vi "Autonomous Independent.vi"() -> ()   [LabVIEW 2017]
doc: "This VI is called when autonomous begins, and will automatically be terminated when autonomous ends. You can carry out timed or sensor driven robot movement independently without needing to return to the caller."
uses:
  <vilib>/Rock Robotics/WPI/Solenoid/WPI_SolenoidValue.ctl
  <vilib>/Rock Robotics/WPI/Utilities/WPI_GetSetVariantRefNum.vi
  <vilib>/Rock Robotics/Network Tables/NT Read String.vi
  <vilib>/Rock Robotics/Network Tables/NT Write Numeric Array.vi
  <vilib>/Rock Robotics/WPI/ThirdParty/Phoenix-LabVIEW/Motor Controller/Get/CTRE_Phoenix_MotorController_GetQuadratureData.vi
  Robot Global Data.vi
  <vilib>/addons/control/pid/pid.llb/PID (DBL).vi
  <vilib>/Rock Robotics/WPI/RobotDrive/WPI_RobotDriveArcadeDrive_Standard(NoSaturation).vi
  <vilib>/Rock Robotics/WPI/Solenoid/WPI_SolenoidSetEnum.vi
  <vilib>/Rock Robotics/WPI/Solenoid/Deprecated/WPI_SolenoidGetBool.vi
  <vilib>/Rock Robotics/WPI/ThirdParty/Phoenix-LabVIEW/Motor Controller/Get/CTRE_Phoenix_MotorController_GetGeneralStatus.vi
  <vilib>/addons/control/pid/NI_PID_pid.lvlib
panel:
  out "Place 2 Scale":bool
  out "Place 1 Scale":bool
  out "Robots Decision 2":string
  out "Place Switch and Scale":bool
  out "Drive Forward":bool
  out "Place 2 Switch":bool
  out "Center Place 1 Switch":bool
  out "Game Data":string
  out "Right":bool
  out "Center":bool
  out "Left":bool
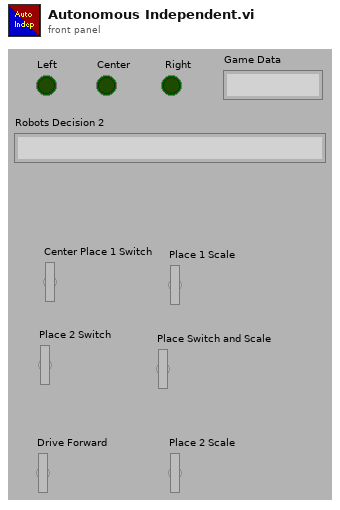
[diagram p1: front panel]
types:
  T1 = enum16{"Drive Forward", "None", "Right", "Center", "Left"}
  T2 = typedef "WPI_JoystickDevRef.ctl" = cluster{"Device":T3}
  T3 = typedef "WPI_JoystickDeviceEnum.ctl" = enum16{"USB 0", "USB 1", "USB 2", "USB 3", "USB 4", "USB 5"}
  T4 = enum16{"Place 2 Scale Left", "Place 2 Scale Right", "Place Scale Right", "Place Switch and Scale Right", "Place 2 Switch Right", "Center Place 2 Switch Right", "Center Place 1 Switch Right", "Center Place 2 Switch Left", "Center Place 1 Switch Left", "Place Scale Left", "Place Switch and Scale Left", "Place 2 Switch Left", "Drive forward", "Do Nothing"}
  T5 = enum16{"Place 2 Scale", "Place 1 Scale", "Place Switch and Scale", "Place 2 Switch", "Center Place 2 Switch", "Center Place 1 Switch", "None"}
  T6 = typedef "WPI_SolenoidValue.ctl" = enum16{"Off", "On", "Forward", "Reverse"}
  T7 = cluster{"proportional gain (Kc)":dbl, "integral time (Ti, min)":dbl, "derivative time (Td, min)":dbl}
  T8 = typedef "WPI_MotorControlDeviceRef.ctl" = cluster{"DeviceStatus":errorcluster, "Type":T9, "PWM":cluster{"PWM Channel":T10, "DeadBand":T11}, "CAN":cluster{"Device Number":u8, "SetOutput VI Ref":variant, "GetOutput VI Ref":variant, "Enable VI Ref":variant, "Disable VI Ref":variant, "Data":variant}, "Invert":bool, "DIO PWM":cluster{"PWM \"Enable\" Channel":T10, "DIOChannel":T12, "PWM Rate":dbl}}
  T9 = typedef "WPI_MotorControlType.ctl" = enum16{"PWM", "CAN", "DIO PWM"}
  T10 = typedef "FPGA_DIOPWMChannel.ctl" = enum8{"PWM 0", "PWM 1", "PWM 2", "PWM 3", "PWM 4", "PWM 5", "PWM 6", "PWM 7", "PWM 8", "PWM 9", "PWM MXP 0", "PWM MXP 1", "PWM MXP 2", "PWM MXP 3", "PWM MXP 4", "PWM MXP 5", "PWM MXP 6", "PWM MXP 7", "PWM MXP 8", "PWM MXP 9", "Invalid"}
  T11 = typedef "WPI_PWMDeadband.ctl" = cluster{"Name":string, "maxPositivePwm":i32, "minPositivePwm":i32, "centerPwm":i32, "maxNegativePwm":i32, "minNegativePwm":i32, "angularRange":u16}
  T12 = typedef "FPGA_DIOChannel.ctl" = enum8{"DIO 0", "DIO 1", "DIO 2", "DIO 3", "DIO 4", "DIO 5", "DIO 6", "DIO 7", "DIO 8", "DIO 9", "DIO MXP 0", "DIO MXP 1", "DIO MXP 2", "DIO MXP 3", "DIO MXP 4", "DIO MXP 5", "DIO MXP 6", "DIO MXP 7", "DIO MXP 8", "DIO MXP 9", "DIO MXP 10", "DIO MXP 11", "DIO MXP 12", "DIO MXP 13", "DIO MXP 14", "DIO MXP 15", "SPI Port CS1", "SPI Port CS2", "SPI Port CS3", "SPI Port MISO", "SPI Port MOSI", "Invalid"}
  T13 = typedef "CTRE_PigeonIMU_DeviceRef.ctl" = cluster{"DeviceStatus":errorcluster, "Device Number":u8, "Type":T14, "Device ID":u32, "Handle":u64, "UsageFrame":u32, "Library Path":path}
  T14 = typedef "CTRE_PigeonIMU_ConnectionType.ctl" = u32
  T15 = typedef "WPI_RobotDriveDevRef.ctl" = cluster{"DevStatus":errorcluster, "Motors[]":T8[], "Square Inputs":bool, "Max Output":dbl}
  T16 = typedef "WPI_SolenoidDevRef.ctl" = cluster{"DevStatus":errorcluster, "Pneumatics Control Module":u8, "Forward Solenoid Channel":T17, "Reverse Solenoid Channel":T17}
  T17 = typedef "WPI_SolenoidChannel.ctl" = enum8{"Solenoid 0", "Solenoid 1", "Solenoid 2", "Solenoid 3", "Solenoid 4", "Solenoid 5", "Solenoid 6", "Solenoid 7", "Invalid"}
  T18 = typedef "WPI_DigitalInputDevRef.ctl" = cluster{"DevStatus":errorcluster, "DIO Channel":T12}
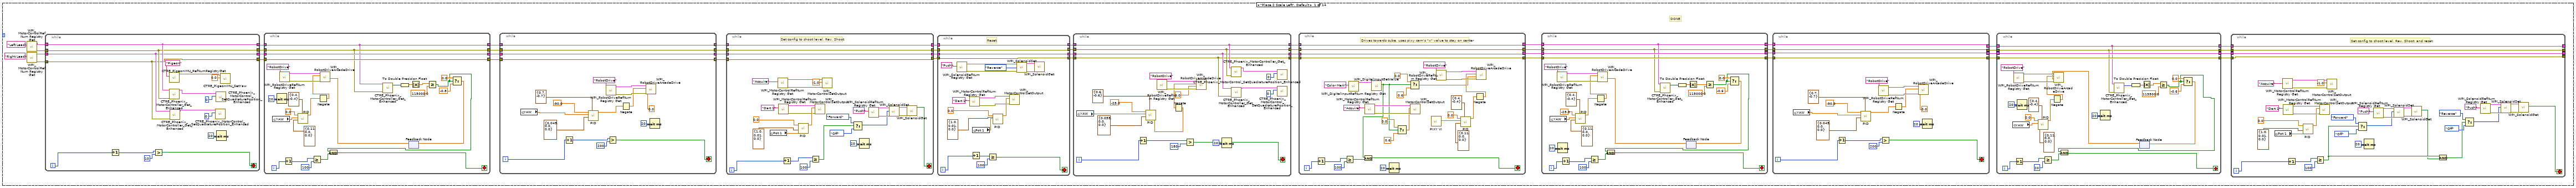
[diagram p2: hidden frame]
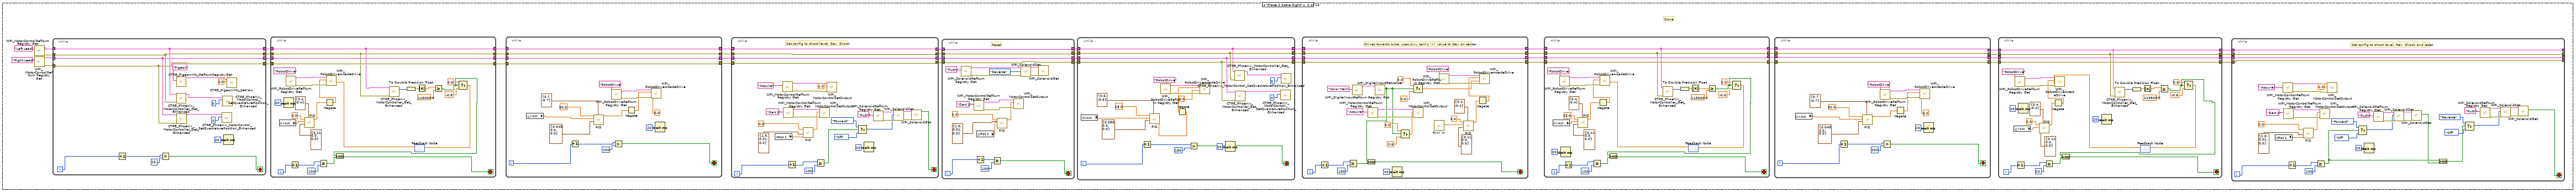
[diagram p3: hidden frame]
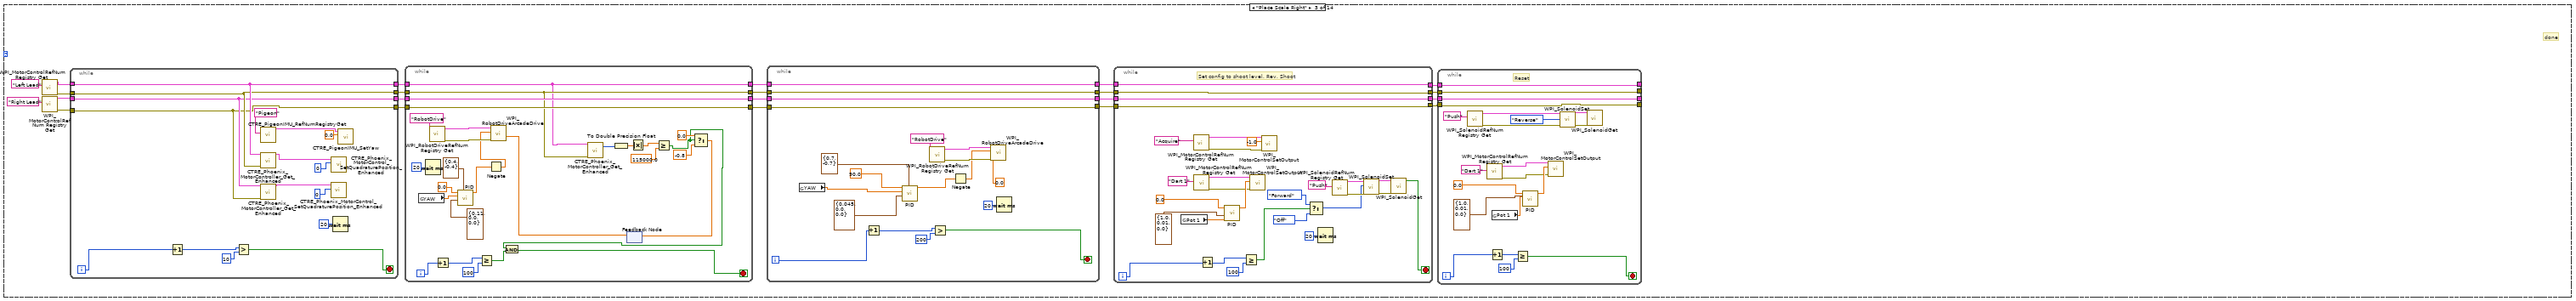
[diagram p4: hidden frame]
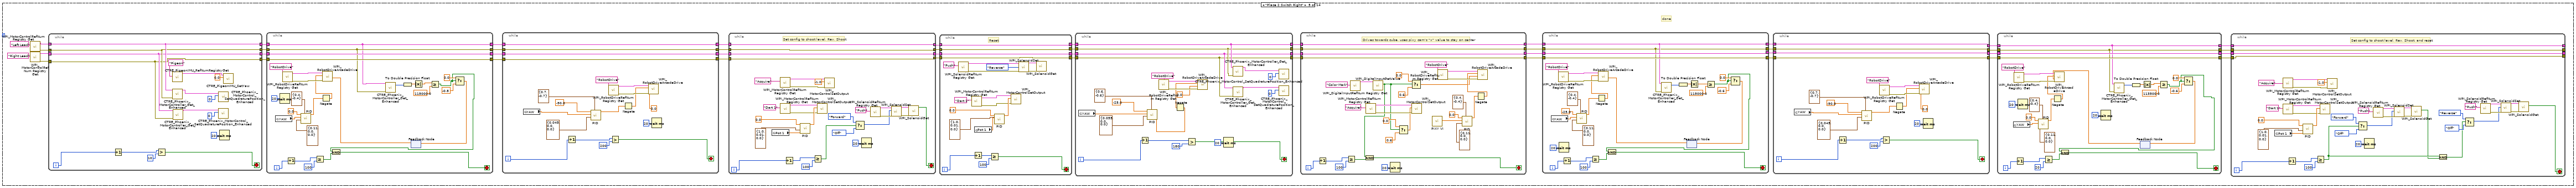
[diagram p5: hidden frame]
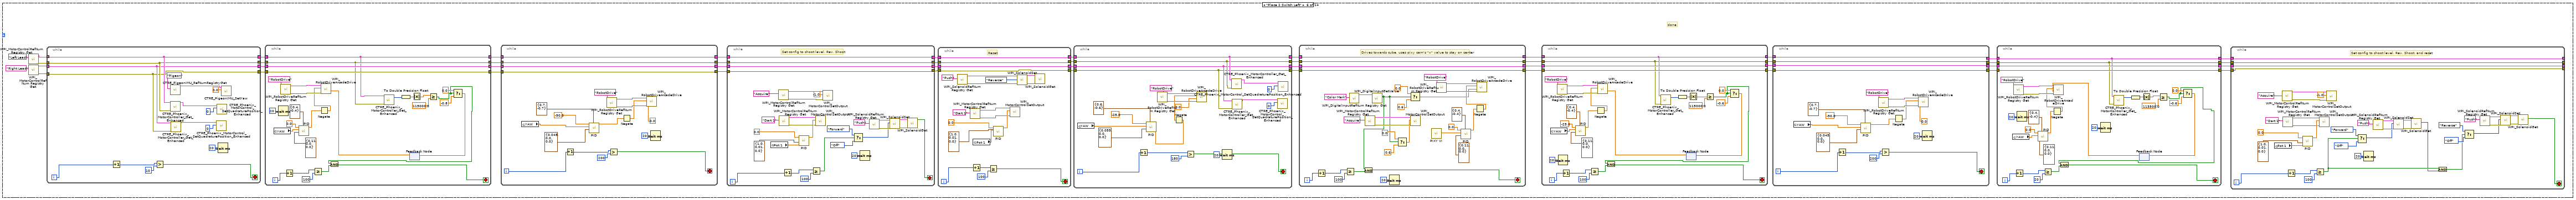
[diagram p6: hidden frame]
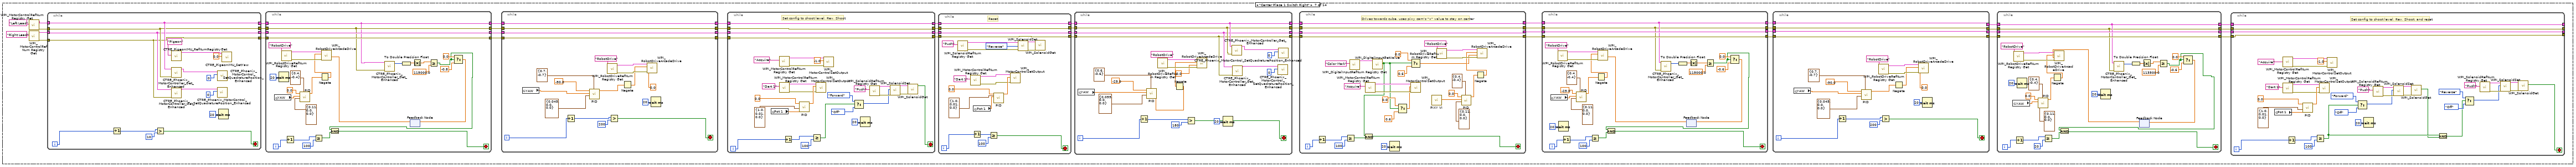
[diagram p7: hidden frame]
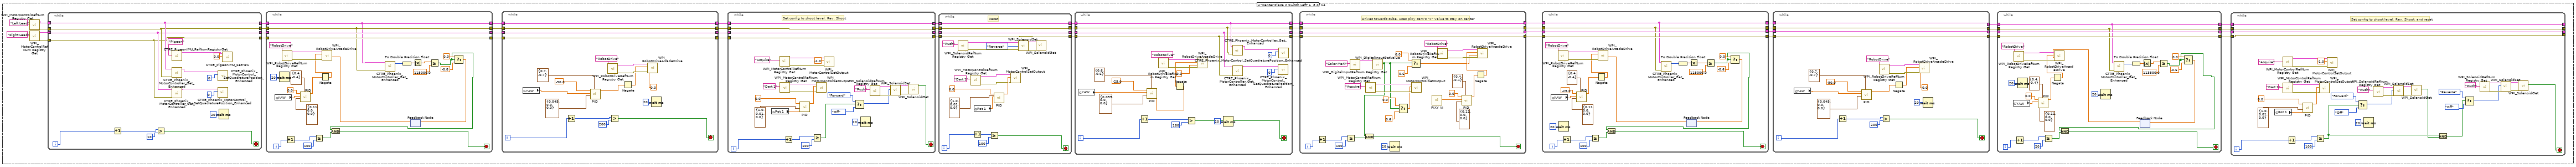
[diagram p8: hidden frame]
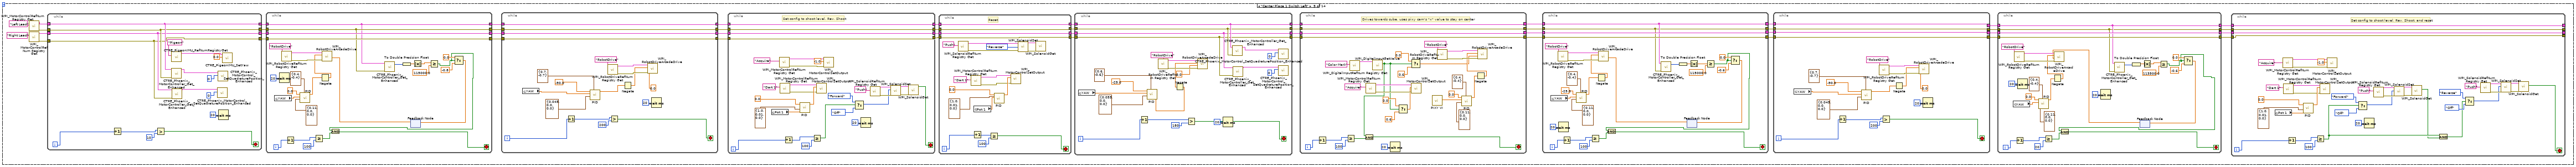
[diagram p9: hidden frame]
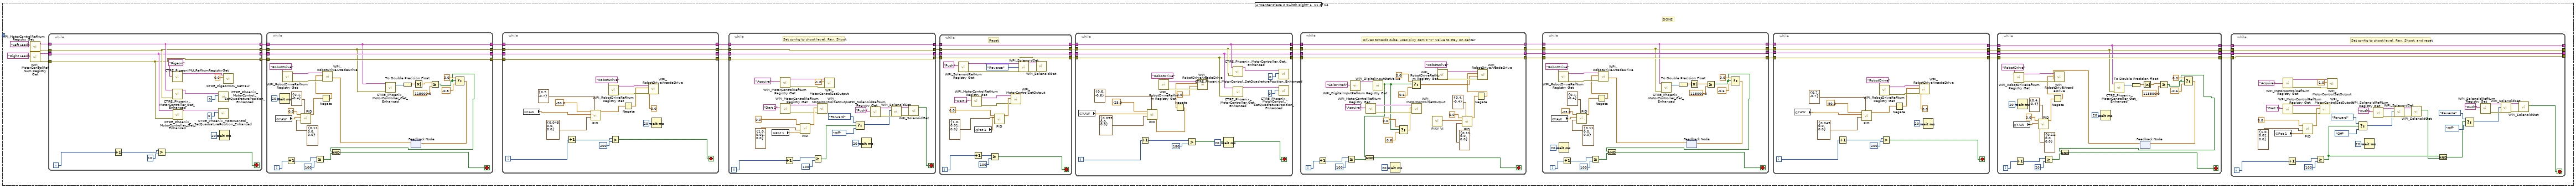
[diagram p11: hidden frame]
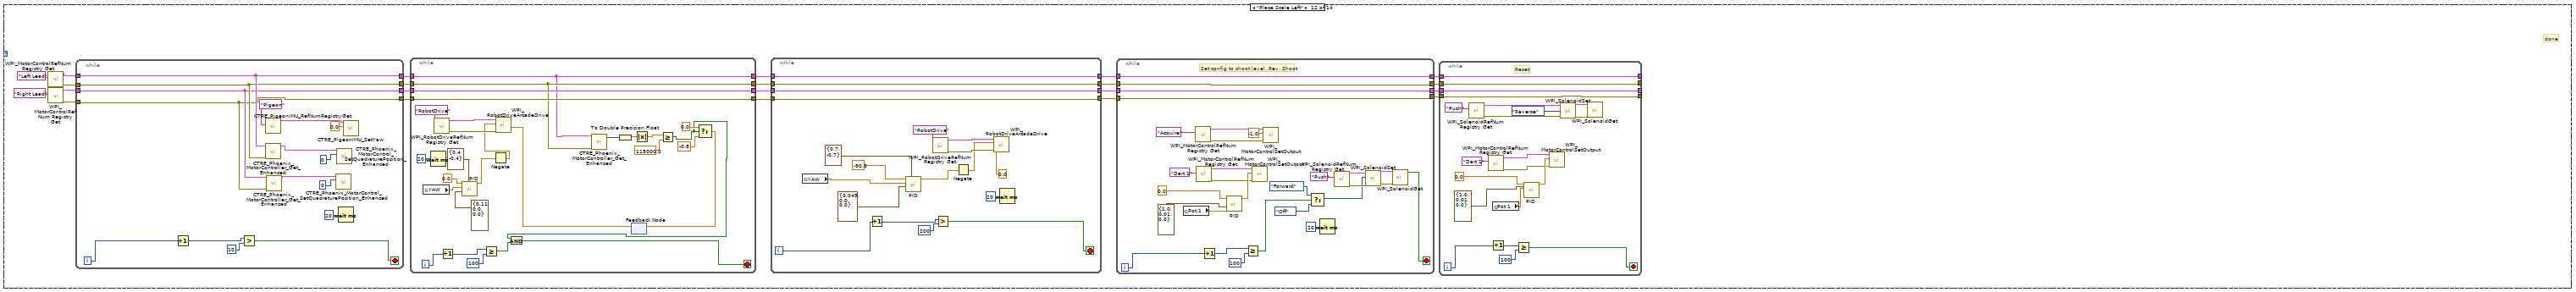
[diagram p12: hidden frame]
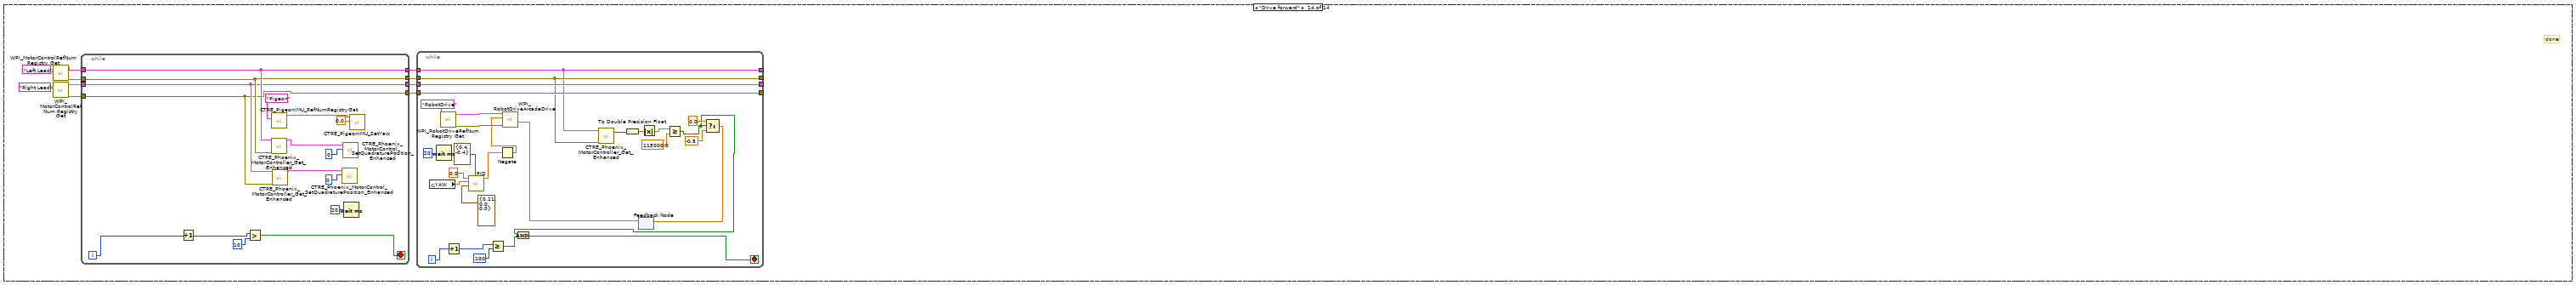
[diagram p14: hidden frame]
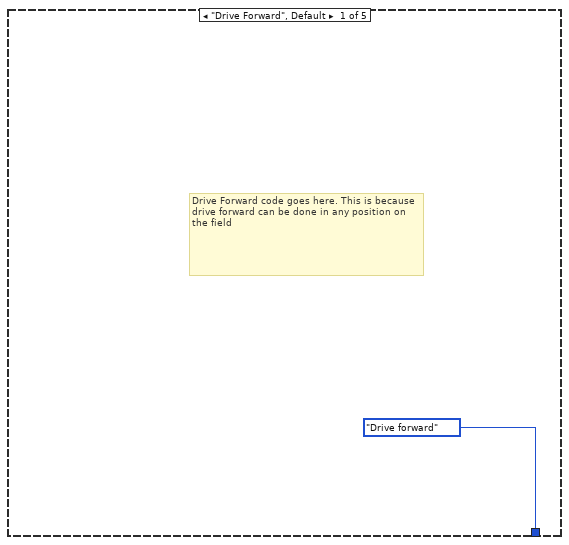
[diagram p15: hidden frame]
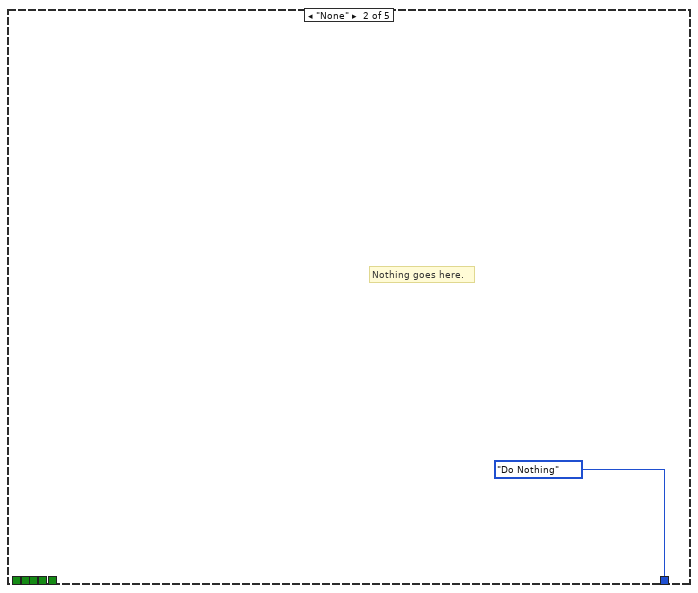
[diagram p16: hidden frame]
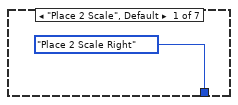
[diagram p17: hidden frame]
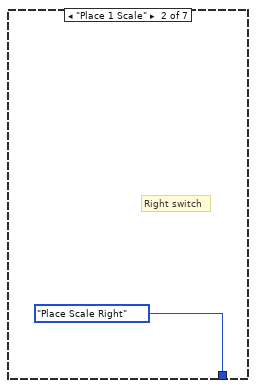
[diagram p18: hidden frame]
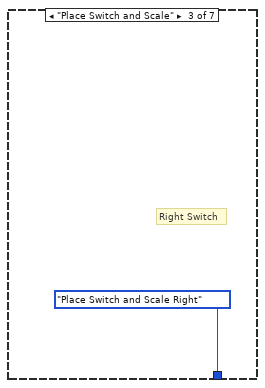
[diagram p19: hidden frame]
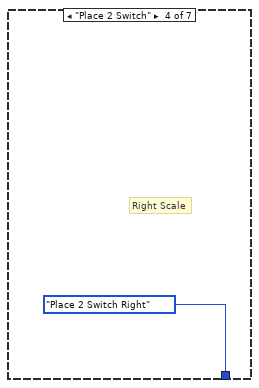
[diagram p20: hidden frame]
diagram:
  (unwired) "This function is run in parallel when the autonomous period begins. It will be terminated automatically when the period ends.\n\nNote that all Driver Station inputs are automatically latched and will not change once auto begins."
  # "5"
  # "LOGIC ALGORITHM"
  # "ALL AUTON STEPS GOES HERE"
  # "Players Choice"
  # "Order of difficulty"
  # "4"
  # "3"
  # "2"
  # "1"
  # "Game Data"
  # "Position"
  # "Position"
  # "LOGIC ALGORITHM"
  # "ALL AUTON STEPS GOES HERE"
  # "Position"
  # "This tells you the autonomous selected\nfrom the dashboard"
  # "Every 20ms, report that we are running autonomous\ncode. Loop will abort the same time as the VI."
  # "This gives you the joystick value\nthat is often the throttle"
  # "This tells you the driver position\nand alliance color"
  n1 = call <vilib>:"WPI_JoystickRefNum Registry Get.vi"("refnum name"="Autons") -> ("error out"=w43:errorcluster, "JoystickDevRef"=w44:T2)  [unwired: 9 in]
  n2 = call <vilib>:"WPI_JoystickGetValues.vi"("error in (no error)"=w43, "JoystickDevRef"=w44) -> ("Buttons"=w41:bool[])  [unwired: 5 in, 4 out]
  n3 = Index Array(array=w41) -> (element #1=w10:bool, element #2=w9:bool, element #3=w8:bool, element #4=w7:bool, element #5=w6:bool, element #6=w5:bool, element #7=w4:bool, element #8=w3:bool, element #9=w2:bool)  [unwired: 19 in, 10 out]
  "Left" <- w10
  "Center" <- w9
  "Right" <- w8
  "Center Place 1 Switch" <- w6
  "Place 2 Switch" <- w5
  "Drive Forward" <- w7
  "Place Switch and Scale" <- w2
  "Place 1 Scale" <- w4
  "Place 2 Scale" <- w3
  n4 = call <vilib>:"WPI_DriverStationGame Specific Data.vi"() -> ("Game Specific Data"=w1:string)  [unwired: 11 in]
  "Game Data" <- w1
  n5 = Select(t=T1."Right", s=w8, f=T1."None") -> (s? t:f=w37:T1)
  n6 = String Subset(string=w1, length (rest)=2 ("length (rest)")) -> (substring=w32:string)  [unwired: 1 in]
  n7 = Select(t=T1."Center", s=w9, f=w37) -> (s? t:f=w38:T1)
  n8 = Equal?(x=w32, y="RL") -> (x = y?=w26:bool)
  n9 = Equal?(x=w32, y="LR") -> (x = y?=w25:bool)
  n10 = Equal?(x=w32, y="LL") -> (x = y?=w28:bool)
  n11 = Equal?(x=w32, y="RR") -> (x = y?=w27:bool)
  n12 = Select(t=T1."Left", s=w10, f=w38) -> (s? t:f=w15:T1)
  n13 = Select(t=enum16{"None", "LR", "RL", "LL", "RR"}."LR", s=w25, f=enum16{"None", "LR", "RL", "LL", "RR"}."None") -> (s? t:f=w22:enum16{"None", "LR", "RL", "LL", "RR"})
  n14 = Select(t=enum16{"None", "LR", "RL", "LL", "RR"}."RL", s=w26, f=w22) -> (s? t:f=w23:enum16{"None", "LR", "RL", "LL", "RR"})
  n15 = Select(t=enum16{"None", "LR", "RL", "LL", "RR"}."RR", s=w27, f=w23) -> (s? t:f=w24:enum16{"None", "LR", "RL", "LL", "RR"})
  n16 = Select(t=enum16{"None", "LR", "RL", "LL", "RR"}."LL", s=w28, f=w24) -> (s? t:f=w16:enum16{"None", "LR", "RL", "LL", "RR"})
  n17 = Select(t=T1."Drive Forward", s=w7, f=w15) -> (s? t:f=w13:T1)
  n18 = case shown="\"Right\"" w13 {
    tunnel: w16 -> [_ _ w59 w140 w244]
    tunnel: w6 -> [_ _ w56 w136 w243]
    tunnel: w5 -> [_ _ w57 w137 w242]
    tunnel: w4 -> [_ _ w55 w138 w241]
    tunnel: w2 -> [_ _ w58 w139 w240]
    tunnel: w3 -> [_ _ w54 w134 w238]
    tunnel: [T4."Drive forward" T4."Do Nothing" w53 w135 w239] -> w11
    frame "Drive Forward", Default {
      # "Drive Forward code goes here. This is because drive forward can be done in any position on the field"
    }
    frame "None" {
      # "Nothing goes here."
    }
    frame "Right" {
      # "Game Data"
      n19 = case shown="\"RR\"" w59 {
        tunnel: w58 -> [w68 _ w91 w111 _]
        tunnel: w55 -> [w73 _ w89 w113 _]
        tunnel: w57 -> [w72 _ w88 w114 _]
        tunnel: w56 -> [w71 _ w87 w115 _]
        tunnel: w54 -> [w67 _ w90 w112 _]
        tunnel: [w61 T4."Drive forward" w86 w109 T4."Do Nothing"] -> w53
        frame "RR" {
          # "Can do any auton"
          # "Right RR"
          n20 = Select(t=T5."Place Switch and Scale", s=w68, f=T5."None") -> (s? t:f=w69:T5)
          n21 = Select(t=T5."Place 2 Scale", s=w67, f=w69) -> (s? t:f=w76:T5)
          n22 = Select(t=T5."Place 1 Scale", s=w73, f=w76) -> (s? t:f=w75:T5)
          n23 = Select(t=T5."Place 2 Switch", s=w72, f=w75) -> (s? t:f=w74:T5)
          n24 = Select(t=T5."Place 1 Scale", s=w71, f=w74) -> (s? t:f=w70:T5)
          n25 = case shown="\"None\"" w70 {
            tunnel: [T4."Place 2 Scale Right" T4."Place Scale Right" T4."Place Switch and Scale Right" T4."Place 2 Switch Right" T4."Do Nothing" T4."Do Nothing" T4."Do Nothing"] -> w61
            frame "Place 2 Scale", Default {
            }
            frame "Place 1 Scale" {
              # "Right switch"
            }
            frame "Place Switch and Scale" {
              # "Right Switch"
            }
            frame "Place 2 Switch" {
              # "Right Scale"
            }
            frame "Center Place 2 Switch" {
              # "Right Side"
            }
            frame "Center Place 1 Switch" {
            }
            frame "None" {
            }
          }
        }
        frame "LL" {
          # "All code gets written into a seperate case strucutre that is linked with the robot deicision made here.\nThis allows us to use the auton code \"universal\" and acts as an extension for ease of writing as well."
          # "You can not score a cube so drive forward code goes here"
          # "Right LL"
        }
        frame "RL" {
          # "Can do any auton"
          # "Right RL"
          n26 = Select(t=T5."Place 2 Switch", s=w91, f=T5."None") -> (s? t:f=w97:T5)
          n27 = Select(t=T5."Place 2 Switch", s=w90, f=w97) -> (s? t:f=w101:T5)
          n28 = Select(t=T5."Place 2 Switch", s=w89, f=w101) -> (s? t:f=w100:T5)
          n29 = Select(t=T5."Place 2 Switch", s=w88, f=w100) -> (s? t:f=w99:T5)
          n30 = Select(t=T5."Place 2 Switch", s=w87, f=w99) -> (s? t:f=w98:T5)
          n31 = case shown="\"Center Place 2 Switch\"" w98 {
            tunnel: [T4."Place 2 Scale Right" T4."Place Scale Right" T4."Place Switch and Scale Right" T4."Place 2 Switch Right" T4."Do Nothing" T4."Do Nothing" T4."Do Nothing"] -> w86
            frame "Place 2 Scale", Default {
            }
            frame "Place 1 Scale" {
              # "Right switch"
            }
            frame "Place Switch and Scale" {
              # "Right Switch"
            }
            frame "Place 2 Switch" {
              # "Right Scale"
            }
            frame "Center Place 2 Switch" {
              # "Right Side"
            }
            frame "Center Place 1 Switch" {
            }
            frame "None" {
            }
          }
        }
        frame "LR" {
          # "Can do any auton"
          # "Right LR"
          n32 = Select(t=T5."Place 2 Scale", s=w111, f=T5."None") -> (s? t:f=w121:T5)
          n33 = Select(t=T5."Place 2 Scale", s=w112, f=w121) -> (s? t:f=w125:T5)
          n34 = Select(t=T5."Place 1 Scale", s=w113, f=w125) -> (s? t:f=w124:T5)
          n35 = Select(t=T5."Place 2 Scale", s=w114, f=w124) -> (s? t:f=w123:T5)
          n36 = Select(t=T5."Place 2 Scale", s=w115, f=w123) -> (s? t:f=w122:T5)
          n37 = case shown="\"Place 1 Scale\"" w122 {
            tunnel: [T4."Place 2 Scale Right" T4."Place Scale Right" T4."Place Switch and Scale Right" T4."Place 2 Switch Right" T4."Do Nothing" T4."Do Nothing" T4."Do Nothing"] -> w109
            frame "Place 2 Scale", Default {
            }
            frame "Place 1 Scale" {
              # "Right switch"
            }
            frame "Place Switch and Scale" {
              # "Right Switch"
            }
            frame "Place 2 Switch" {
              # "Right Scale"
            }
            frame "Center Place 2 Switch" {
              # "Right Side"
            }
            frame "Center Place 1 Switch" {
            }
            frame "None" {
            }
          }
        }
        frame "None" {
          # "Nothing goes here."
        }
      }
    }
    frame "Center" {
      # "Game Data"
      n38 = case shown="\"LR\"" w140 {
        tunnel: w139 -> [w146 w170 w191 w216 _]
        tunnel: w138 -> [w144 w168 w192 w217 _]
        tunnel: w137 -> [w143 w167 w193 w218 _]
        tunnel: w136 -> [w142 w166 w194 w219 _]
        tunnel: [w141 w165 w189 w214 T4."Do Nothing"] -> w135
        tunnel: w134 -> [w145 w169 w190 w213 _]
        frame "RR" {
          # "Can do any auton"
          # "Center RR"
          n39 = Select(t=T5."Place 2 Switch", s=w146, f=T5."None") -> (s? t:f=w153:T5)
          n40 = Select(t=T5."Place 2 Switch", s=w145, f=w153) -> (s? t:f=w157:T5)
          n41 = Select(t=T5."Place 2 Switch", s=w144, f=w157) -> (s? t:f=w156:T5)
          n42 = Select(t=T5."Place 2 Switch", s=w143, f=w156) -> (s? t:f=w155:T5)
          n43 = Select(t=T5."Center Place 1 Switch", s=w142, f=w155) -> (s? t:f=w154:T5)
          n44 = case shown="\"Place 2 Scale\", Default" w154 {
            tunnel: [T4."Place 2 Scale Right" T4."Place Scale Right" T4."Place Switch and Scale Right" T4."Center Place 2 Switch Right" T4."Center Place 2 Switch Right" T4."Center Place 1 Switch Right" T4."Do Nothing"] -> w141
            frame "Place 2 Scale", Default {
            }
            frame "Place 1 Scale" {
              # "Right switch"
            }
            frame "Place Switch and Scale" {
              # "Right Switch"
            }
            frame "Place 2 Switch" {
            }
            frame "Center Place 2 Switch" {
            }
            frame "Center Place 1 Switch" {
            }
            frame "None" {
            }
          }
        }
        frame "LL" {
          # "Can do any auton"
          # "Center LL"
          n45 = Select(t=T5."Place 2 Switch", s=w170, f=T5."None") -> (s? t:f=w177:T5)
          n46 = Select(t=T5."Place 2 Switch", s=w169, f=w177) -> (s? t:f=w181:T5)
          n47 = Select(t=T5."Place 2 Switch", s=w168, f=w181) -> (s? t:f=w180:T5)
          n48 = Select(t=T5."Place 2 Switch", s=w167, f=w180) -> (s? t:f=w179:T5)
          n49 = Select(t=T5."Center Place 1 Switch", s=w166, f=w179) -> (s? t:f=w178:T5)
          n50 = case shown="\"None\"" w178 {
            tunnel: [T4."Place 2 Scale Right" T4."Place Scale Right" T4."Place Switch and Scale Right" T4."Center Place 2 Switch Left" T4."Center Place 2 Switch Left" T4."Center Place 1 Switch Left" T4."Do Nothing"] -> w165
            frame "Place 2 Scale", Default {
            }
            frame "Place 1 Scale" {
              # "Right switch"
            }
            frame "Place Switch and Scale" {
              # "Right Switch"
            }
            frame "Place 2 Switch" {
            }
            frame "Center Place 2 Switch" {
            }
            frame "Center Place 1 Switch" {
            }
            frame "None" {
            }
          }
        }
        frame "RL" {
          # "Can do any auton"
          # "Center RL"
          n51 = Select(t=T5."Place 2 Switch", s=w191, f=T5."None") -> (s? t:f=w201:T5)
          n52 = Select(t=T5."Place 2 Switch", s=w190, f=w201) -> (s? t:f=w205:T5)
          n53 = Select(t=T5."Place 2 Switch", s=w192, f=w205) -> (s? t:f=w204:T5)
          n54 = Select(t=T5."Place 2 Switch", s=w193, f=w204) -> (s? t:f=w203:T5)
          n55 = Select(t=T5."Center Place 1 Switch", s=w194, f=w203) -> (s? t:f=w202:T5)
          n56 = case shown="\"Center Place 1 Switch\"" w202 {
            tunnel: [T4."Place 2 Scale Right" T4."Place Scale Right" T4."Place Switch and Scale Right" T4."Center Place 2 Switch Right" T4."Center Place 2 Switch Right" T4."Center Place 1 Switch Right" T4."Do Nothing"] -> w189
            frame "Place 2 Scale", Default {
            }
            frame "Place 1 Scale" {
              # "Right switch"
            }
            frame "Place Switch and Scale" {
              # "Right Switch"
            }
            frame "Place 2 Switch" {
            }
            frame "Center Place 2 Switch" {
            }
            frame "Center Place 1 Switch" {
            }
            frame "None" {
            }
          }
        }
        frame "LR" {
          # "Can do any auton"
          # "Center LR"
          n57 = Select(t=T5."Place 2 Switch", s=w216, f=T5."None") -> (s? t:f=w225:T5)
          n58 = Select(t=T5."Place 2 Switch", s=w213, f=w225) -> (s? t:f=w229:T5)
          n59 = Select(t=T5."Place 2 Switch", s=w217, f=w229) -> (s? t:f=w228:T5)
          n60 = Select(t=T5."Place 2 Switch", s=w218, f=w228) -> (s? t:f=w227:T5)
          n61 = Select(t=T5."Center Place 1 Switch", s=w219, f=w227) -> (s? t:f=w226:T5)
          n62 = case shown="\"Center Place 1 Switch\"" w226 {
            tunnel: [T4."Place 2 Scale Right" T4."Place Scale Right" T4."Place Switch and Scale Right" T4."Center Place 2 Switch Left" T4."Center Place 2 Switch Left" T4."Center Place 1 Switch Left" T4."Do Nothing"] -> w214
            frame "Place 2 Scale", Default {
            }
            frame "Place 1 Scale" {
              # "Right switch"
            }
            frame "Place Switch and Scale" {
              # "Right Switch"
            }
            frame "Place 2 Switch" {
            }
            frame "Center Place 2 Switch" {
            }
            frame "Center Place 1 Switch" {
            }
            frame "None" {
            }
          }
        }
        frame "None" {
          # "Nothing goes here."
        }
      }
    }
    frame "Left" {
      n63 = case shown="\"RR\"" w244 {
        tunnel: w243 -> [_ w246 w270 w294 _]
        tunnel: w242 -> [_ w247 w271 w295 _]
        tunnel: w241 -> [_ w248 w272 w296 _]
        tunnel: w240 -> [_ w250 w274 w298 _]
        tunnel: [T4."Drive forward" w251 w275 w299 T4."Do Nothing"] -> w239
        tunnel: w238 -> [_ w249 w273 w297 _]
        frame "RR" {
          # "Game Data"
          # "You can not score a cube so drive forward code goes here"
          # "Left RR"
        }
        frame "LL" {
          # "Can do any auton"
          # "Left LL"
          n64 = Select(t=T5."Place Switch and Scale", s=w250, f=T5."None") -> (s? t:f=w258:T5)
          n65 = Select(t=T5."Place 2 Scale", s=w249, f=w258) -> (s? t:f=w262:T5)
          n66 = Select(t=T5."Place 1 Scale", s=w248, f=w262) -> (s? t:f=w261:T5)
          n67 = Select(t=T5."Place 2 Switch", s=w247, f=w261) -> (s? t:f=w260:T5)
          n68 = Select(t=T5."Place Switch and Scale", s=w246, f=w260) -> (s? t:f=w259:T5)
          n69 = case shown="\"None\"" w259 {
            tunnel: [T4."Place 2 Scale Left" T4."Place Scale Left" T4."Place Switch and Scale Left" T4."Place 2 Switch Left" T4."Center Place 2 Switch Right" T4."Center Place 1 Switch Right" T4."Do Nothing"] -> w251
            frame "Place 2 Scale", Default {
            }
            frame "Place 1 Scale" {
              # "Right switch"
            }
            frame "Place Switch and Scale" {
            }
            frame "Place 2 Switch" {
            }
            frame "Center Place 2 Switch" {
            }
            frame "Center Place 1 Switch" {
            }
            frame "None" {
            }
          }
        }
        frame "RL" {
          # "Can do any auton"
          # "Left RL"
          n70 = Select(t=T5."Place 2 Scale", s=w274, f=T5."None") -> (s? t:f=w282:T5)
          n71 = Select(t=T5."Place 2 Scale", s=w273, f=w282) -> (s? t:f=w286:T5)
          n72 = Select(t=T5."Place 1 Scale", s=w272, f=w286) -> (s? t:f=w285:T5)
          n73 = Select(t=T5."Place 2 Scale", s=w271, f=w285) -> (s? t:f=w284:T5)
          n74 = Select(t=T5."Place 2 Scale", s=w270, f=w284) -> (s? t:f=w283:T5)
          n75 = case shown="\"None\"" w283 {
            tunnel: [T4."Place 2 Scale Left" T4."Place Scale Left" T4."Place Switch and Scale Right" T4."Place 2 Switch Left" T4."Center Place 2 Switch Right" T4."Center Place 1 Switch Right" T4."Do Nothing"] -> w275
            frame "Place 2 Scale", Default {
            }
            frame "Place 1 Scale" {
              # "Right switch"
            }
            frame "Place Switch and Scale" {
              # "Right Switch"
            }
            frame "Place 2 Switch" {
            }
            frame "Center Place 2 Switch" {
            }
            frame "Center Place 1 Switch" {
            }
            frame "None" {
            }
          }
        }
        frame "LR" {
          # "Can do any auton"
          # "Left LR"
          n76 = Select(t=T5."Place 2 Switch", s=w298, f=T5."None") -> (s? t:f=w306:T5)
          n77 = Select(t=T5."Place 2 Switch", s=w297, f=w306) -> (s? t:f=w310:T5)
          n78 = Select(t=T5."Place 2 Switch", s=w296, f=w310) -> (s? t:f=w309:T5)
          n79 = Select(t=T5."Place 2 Switch", s=w295, f=w309) -> (s? t:f=w308:T5)
          n80 = Select(t=T5."Place 2 Switch", s=w294, f=w308) -> (s? t:f=w307:T5)
          n81 = case shown="\"Place 2 Switch\"" w307 {
            tunnel: [T4."Place 2 Scale Right" T4."Place Scale Right" T4."Place Switch and Scale Right" T4."Place 2 Switch Left" T4."Center Place 2 Switch Right" T4."Center Place 1 Switch Right" T4."Do Nothing"] -> w299
            frame "Place 2 Scale", Default {
            }
            frame "Place 1 Scale" {
              # "Right switch"
            }
            frame "Place Switch and Scale" {
              # "Right Switch"
            }
            frame "Place 2 Switch" {
            }
            frame "Center Place 2 Switch" {
            }
            frame "Center Place 1 Switch" {
            }
            frame "None" {
            }
          }
        }
        frame "None" {
          # "Nothing goes here."
        }
      }
    }
  }
  n82 = case shown="\"Place Switch and Scale Right\"" w11 {
    frame "Place 2 Scale Left", Default {
      # "DONE"
      n83 = call <vilib>:"WPI_MotorControlRefNum Registry Get.vi"("refnum name"="Left Lead") -> ("error out"=w323:errorcluster, "MotorControlDevRef"=w324:T8)  [unwired: 9 in]
      n84 = call <vilib>:"WPI_MotorControlRefNum Registry Get.vi"("refnum name"="Right Lead") -> ("error out"=w321:errorcluster, "MotorControlDevRef"=w322:T8)  [unwired: 9 in]
      n85 = while {
        tunnel: w324 -> [w606]
        tunnel: w323 -> [w605]
        tunnel: w322 -> [w604]
        tunnel: w321 -> [w603]
        tunnel: [w606] -> w364
        tunnel: [w605] -> w363
        tunnel: [w604] -> w362
        tunnel: [w603] -> w361
        i -> [w616]
        stop <- w615 stop-if-true
        n86 = Increment(x=w616) -> (x+1=w618:i32)
        n87 = Greater?(x=w618, y=10) -> (0:w615:bool)
        n88 = call <vilib>:"CTRE_PigeonIMU_RefNumRegistryGet.vi"("refnum name"="Pigeon") -> ("PigeonIMUDevRef"=w613:T13)  [unwired: 9 in, 1 out]
        n89 = call-poly <vilib>:"CTRE_Phoenix_MotorController_Get_Enhanced.vi"("PhoenixMotorControlDevRef"=w606, "error in"=w605) -> ("PhoenixMotorControlDevRef"=w608:T8)  [unwired: 10 in, 3 out]
        n90 = call-poly <vilib>:"CTRE_Phoenix_MotorController_Get_Enhanced.vi"("PhoenixMotorControlDevRef"=w604, "error in"=w603) -> ("PhoenixMotorControlDevRef"=w607:T8)  [unwired: 10 in, 3 out]
        n91 = call "CTRE_Phoenix_MotorControl_SetQuadraturePosition_Enhanced.vi"("New Position"=0, "PhoenixMotorControlDevRef"=w607) -> ()  [unwired: 8 in, 2 out]
        n92 = call "CTRE_Phoenix_MotorControl_SetQuadraturePosition_Enhanced.vi"("New Position"=0, "PhoenixMotorControlDevRef"=w608) -> ()  [unwired: 8 in, 2 out]
        n93 = Wait (ms)(milliseconds to wait=u32 20) -> ()  [unwired: 1 out]
        n94 = call <vilib>:"CTRE_PigeonIMU_SetYaw.vi"("Value"=0.0, "PigeonIMUDevRef"=w613) -> ()  [unwired: 8 in, 2 out]
      }
      n95 = while {
        tunnel: [w621] -> w360
        tunnel: w364 -> [w621]
        tunnel: [w622] -> w359
        tunnel: w363 -> [w622]
        tunnel: [w629] -> w358
        tunnel: w362 -> [w629]
        tunnel: [w628] -> w357
        tunnel: w361 -> [w628]
        i -> [w645]
        stop <- w641 stop-if-true
        n96 = global read "Robot Global Data.vi" "YAW"() -> (w630:dbl)
        n97 = Wait (ms)(milliseconds to wait=u32 20) -> ()  [unwired: 1 out]
        n98 = call <vilib>:"WPI_RobotDriveRefNum Registry Get.vi"("refnum name"="RobotDrive") -> ("error out"=w626:errorcluster, "RobotDriveDevRef"=w627:T15)  [unwired: 9 in]
        n99 = Increment(x=w645) -> (x+1=w644:i32)
        n100 = call-poly <vilib>:"PID.vi"("output range"=cluster{"output high":dbl, "output low":dbl} {"output high"=0.4, "output low"=-0.4}, "PID gains"=T7 {"proportional gain (Kc)"=0.11, "integral time (Ti, min)"=0.0, "derivative time (Td, min)"=0.0}, "process variable"=w630, "setpoint"=0.0) -> ("output"=w620:dbl)  [unwired: 6 in, 1 out]
        n101 = Greater Or Equal?(x=w644, y=100) -> (x >= y?=w642:bool)
        n102 = Negate(x=w620) -> (-x=w619:dbl)
        n103 = call-poly <vilib>:"CTRE_Phoenix_MotorController_Get_Enhanced.vi"("PhoenixMotorControlDevRef"=w621, "error in"=w622) -> ("Quadrature Position"=w640:i32)  [unwired: 10 in, 3 out]
        n104 = To Double Precision Float(number=w640) -> (double precision float=w639:dbl)
        n105 = feedback #1() -> (w623:dbl)  [unwired: 1 in]
        n106 = call-poly <vilib>:"WPI_RobotDriveArcadeDrive.vi"("error in (no error)"=w626, "Y axis value"=w623, "X axis value"=w619, "RobotDriveDevRef"=w627) -> ()  [unwired: 5 in, 3 out]
        n107 = Absolute Value(x=w639) -> (abs(x)=w635:dbl)
        n108 = Greater Or Equal?(x=w635, y=115000.0 ("upper limit")) -> (x >= y?=w624:bool)
        n109 = And(x=w624, y=w642) -> (x .and. y?=w641:bool)
        n110 = Select(t=0.0, s=w624, f=-0.8) -> (s? t:f=w636:dbl)
        n111 = feedback-in #1(w636) -> ()
      }
      n112 = while {
        tunnel: w360 -> [w593]
        tunnel: w359 -> [w592]
        tunnel: w358 -> [w591]
        tunnel: w357 -> [w590]
        tunnel: [w593] -> w356
        tunnel: [w592] -> w355
        tunnel: [w591] -> w354
        tunnel: [w590] -> w353
        i -> [w596]
        stop <- w594 stop-if-true
        n113 = global read "Robot Global Data.vi" "YAW"() -> (w600:dbl)
        n114 = Increment(x=w596) -> (x+1=w598:i32)
        n115 = call-poly <vilib>:"PID.vi"("output range"=cluster{"output high":dbl, "output low":dbl} {"output high"=0.7, "output low"=-0.7}, "PID gains"=T7 {"proportional gain (Kc)"=0.045, "integral time (Ti, min)"=0.0, "derivative time (Td, min)"=0.0}, "process variable"=w600, "setpoint"=-90.0) -> ("output"=w585:dbl)  [unwired: 6 in, 1 out]
        n116 = call <vilib>:"WPI_RobotDriveRefNum Registry Get.vi"("refnum name"="RobotDrive") -> ("error out"=w588:errorcluster, "RobotDriveDevRef"=w589:T15)  [unwired: 9 in]
        n117 = Greater?(x=w598, y=200) -> (0:w594:bool)
        n118 = Negate(x=w585) -> (-x=w584:dbl)
        n119 = call-poly <vilib>:"WPI_RobotDriveArcadeDrive.vi"("error in (no error)"=w588, "Y axis value"=0.0, "X axis value"=w584, "RobotDriveDevRef"=w589) -> ()  [unwired: 5 in, 3 out]
        n120 = Wait (ms)(milliseconds to wait=u32 20) -> ()  [unwired: 1 out]
      }
      n121 = while {
        tunnel: [w493] -> w352
        tunnel: w356 -> [w493]
        tunnel: [w492] -> w351
        tunnel: w355 -> [w492]
        tunnel: [w491] -> w350
        tunnel: w354 -> [w491]
        tunnel: [w494] -> w349
        tunnel: w353 -> [w494]
        i -> [w487]
        stop <- w473 stop-if-true
        # "Set config to shoot level, Rev, Shoot"
        n122 = global read "Robot Global Data.vi" "Pot 1"() -> (w495:dbl)
        n123 = call <vilib>:"WPI_MotorControlRefNum Registry Get.vi"("refnum name"="Acquire") -> ("error out"=w488:errorcluster, "MotorControlDevRef"=w489:T8)  [unwired: 9 in]
        n124 = call <vilib>:"WPI_MotorControlRefNum Registry Get.vi"("refnum name"="Dart 1") -> ("error out"=w499:errorcluster, "MotorControlDevRef"=w498:T8)  [unwired: 9 in]
        n125 = Increment(x=w487) -> (x+1=w474:i32)
        n126 = call-poly <vilib>:"PID.vi"("PID gains"=T7 {"proportional gain (Kc)"=1.0, "integral time (Ti, min)"=0.01, "derivative time (Td, min)"=0.0}, "process variable"=w495, "setpoint"=0.0) -> ("output"=w500:dbl)  [unwired: 7 in, 1 out]
        n127 = Greater Or Equal?(x=w474, y=100) -> (x >= y?=w479:bool)
        n128 = call <vilib>:"WPI_MotorControlSetOutput.vi"("error in (no error)"=w499, "Output"=w500, "MotorControlDevRef"=w498) -> ()  [unwired: 6 in, 3 out]
        n129 = call <vilib>:"WPI_MotorControlSetOutput.vi"("error in (no error)"=w488, "Output"=-1.0, "MotorControlDevRef"=w489) -> ()  [unwired: 6 in, 3 out]
        n130 = Select(t=WPI_SolenoidValue."Forward" ("Value"), s=w479, f=WPI_SolenoidValue."Off" ("Value")) -> (s? t:f=w482:T6)
        n131 = Wait (ms)(milliseconds to wait=u32 20) -> ()  [unwired: 1 out]
        n132 = call <vilib>:"WPI_SolenoidRefNum Registry Get.vi"("refnum name"="Push") -> ("error out"=w483:errorcluster, "SolenoidDevRef"=w484:T16)  [unwired: 9 in]
        n133 = call-poly <vilib>:"WPI_SolenoidSet.vi"("error in (no error)"=w483, "Value"=w482, "SolenoidDevRef"=w484) -> ("error out"=w475:errorcluster, "SolenoidDevRef"=w476:T16)  [unwired: 7 in]
        n134 = call-poly <vilib>:"WPI_SolenoidGet.vi"("error in (no error)"=w475, "SolenoidDevRef"=w476) -> ("Value"=w473:bool)  [unwired: 7 in, 2 out]
      }
      n135 = while {
        tunnel: w352 -> [w379]
        tunnel: w351 -> [w378]
        tunnel: w350 -> [w377]
        tunnel: w349 -> [w376]
        tunnel: [w379] -> w348
        tunnel: [w378] -> w347
        tunnel: [w377] -> w346
        tunnel: [w376] -> w345
        i -> [w367]
        stop <- w366 stop-if-true
        # "Reset"
        n136 = call <vilib>:"WPI_SolenoidRefNum Registry Get.vi"("refnum name"="Push") -> ("error out"=w383:errorcluster, "SolenoidDevRef"=w384:T16)  [unwired: 9 in]
        n137 = call <vilib>:"WPI_MotorControlRefNum Registry Get.vi"("refnum name"="Dart 1") -> ("error out"=w374:errorcluster, "MotorControlDevRef"=w373:T8)  [unwired: 9 in]
        n138 = Increment(x=w367) -> (x+1=w380:i32)
        n139 = global read "Robot Global Data.vi" "Pot 1"() -> (w370:dbl)
        n140 = Greater Or Equal?(x=w380, y=100) -> (x >= y?=w366:bool)
        n141 = call-poly <vilib>:"PID.vi"("PID gains"=T7 {"proportional gain (Kc)"=1.0, "integral time (Ti, min)"=0.01, "derivative time (Td, min)"=0.0}, "process variable"=w370, "setpoint"=0.0) -> ("output"=w375:dbl)  [unwired: 7 in, 1 out]
        n142 = call <vilib>:"WPI_MotorControlSetOutput.vi"("error in (no error)"=w374, "Output"=w375, "MotorControlDevRef"=w373) -> ()  [unwired: 6 in, 3 out]
        n143 = call-poly <vilib>:"WPI_SolenoidSet.vi"("error in (no error)"=w383, "Value"=WPI_SolenoidValue."Reverse", "SolenoidDevRef"=w384) -> ("error out"=w381:errorcluster, "SolenoidDevRef"=w382:T16)  [unwired: 7 in]
        n144 = call-poly <vilib>:"WPI_SolenoidGet.vi"("error in (no error)"=w381, "SolenoidDevRef"=w382) -> ()  [unwired: 7 in, 3 out]
      }
      n145 = while {
        tunnel: [w564] -> w344
        tunnel: w348 -> [w564]
        tunnel: [w563] -> w343
        tunnel: w347 -> [w563]
        tunnel: [w562] -> w342
        tunnel: w346 -> [w562]
        tunnel: [w561] -> w341
        tunnel: w345 -> [w561]
        i -> [w577]
        stop <- w575 stop-if-true
        n146 = global read "Robot Global Data.vi" "YAW"() -> (w581:dbl)
        n147 = Increment(x=w577) -> (x+1=w579:i32)
        n148 = call-poly <vilib>:"PID.vi"("output range"=cluster{"output high":dbl, "output low":dbl} {"output high"=0.6, "output low"=-0.6}, "PID gains"=T7 {"proportional gain (Kc)"=0.055, "integral time (Ti, min)"=0.0, "derivative time (Td, min)"=0.0}, "process variable"=w581, "setpoint"=-25.0) -> ("output"=w571:dbl)  [unwired: 6 in, 1 out]
        n149 = call <vilib>:"WPI_RobotDriveRefNum Registry Get.vi"("refnum name"="RobotDrive") -> ("error out"=w572:errorcluster, "RobotDriveDevRef"=w573:T15)  [unwired: 9 in]
        n150 = Negate(x=w571) -> (-x=w570:dbl)
        n151 = Greater?(x=w579, y=180) -> (0:w575:bool)
        n152 = call-poly <vilib>:"WPI_RobotDriveArcadeDrive.vi"("error in (no error)"=w572, "Y axis value"=0.0, "X axis value"=w570, "RobotDriveDevRef"=w573) -> ()  [unwired: 5 in, 3 out]
        n153 = Wait (ms)(milliseconds to wait=u32 20) -> ()  [unwired: 1 out]
        n154 = call-poly <vilib>:"CTRE_Phoenix_MotorController_Get_Enhanced.vi"("PhoenixMotorControlDevRef"=w564, "error in"=w563) -> ("PhoenixMotorControlDevRef"=w566:T8)  [unwired: 8 in, 5 out]
        n155 = call-poly <vilib>:"CTRE_Phoenix_MotorController_Get_Enhanced.vi"("PhoenixMotorControlDevRef"=w562, "error in"=w561) -> ("PhoenixMotorControlDevRef"=w565:T8)  [unwired: 8 in, 5 out]
        n156 = call "CTRE_Phoenix_MotorControl_SetQuadraturePosition_Enhanced.vi"("New Position"=0, "PhoenixMotorControlDevRef"=w565) -> ()  [unwired: 8 in, 2 out]
        n157 = call "CTRE_Phoenix_MotorControl_SetQuadraturePosition_Enhanced.vi"("New Position"=0, "PhoenixMotorControlDevRef"=w566) -> ()  [unwired: 8 in, 2 out]
      }
      n158 = while {
        tunnel: [w534] -> w340
        tunnel: w344 -> [w534]
        tunnel: [w533] -> w339
        tunnel: w343 -> [w533]
        tunnel: [w532] -> w338
        tunnel: w342 -> [w532]
        tunnel: [w531] -> w337
        tunnel: w341 -> [w531]
        i -> [w559]
        stop <- w555 stop-if-true
        # "Drives towards cube, uses pixy cam's \"x\" value to stay on center"
        n159 = Increment(x=w559) -> (x+1=w558:i32)
        n160 = Greater Or Equal?(x=w558, y=100) -> (x >= y?=w556:bool)
        n161 = call <vilib>:"WPI_DigitalInputRefNum Registry Get.vi"("refnum name"="Color Mark") -> ("DigitalInputDevRef"=w545:T18)  [unwired: 9 in, 1 out]
        n162 = call <vilib>:"WPI_MotorControlRefNum Registry Get.vi"("refnum name"="Acquire") -> ("error out"=w542:errorcluster, "MotorControlDevRef"=w543:T8)  [unwired: 9 in]
        n163 = call <vilib>:"WPI_DigitalInputGetValue.vi"("DigitalInputDevRef"=w545) -> ("Value"=w535:bool)  [unwired: 8 in, 2 out]
        n164 = And(x=w535, y=w556) -> (x .and. y?=w555:bool)
        n165 = Wait (ms)(milliseconds to wait=u32 20) -> ()  [unwired: 1 out]
        n166 = Select(t=0.0, s=w535, f=0.6) -> (s? t:f=w536:dbl)
        n167 = Select(t=0.0, s=w535, f=0.6) -> (s? t:f=w539:dbl)
        n168 = call <vilib>:"WPI_MotorControlSetOutput.vi"("error in (no error)"=w542, "Output"=w536, "MotorControlDevRef"=w543) -> ()  [unwired: 6 in, 3 out]
        n169 = call "PIXY VI.vi"() -> ("X"=w546:dbl)  [unwired: 14 in, 5 out]
        n170 = call <vilib>:"WPI_RobotDriveRefNum Registry Get.vi"("refnum name"="RobotDrive") -> ("error out"=w551:errorcluster, "RobotDriveDevRef"=w552:T15)  [unwired: 9 in]
        n171 = call-poly <vilib>:"PID.vi"("output range"=cluster{"output high":dbl, "output low":dbl} {"output high"=0.4, "output low"=-0.4}, "PID gains"=T7 {"proportional gain (Kc)"=0.11, "integral time (Ti, min)"=0.0, "derivative time (Td, min)"=0.0}, "process variable"=w546, "setpoint"=0.0) -> ("output"=w549:dbl)  [unwired: 6 in, 1 out]
        n172 = Negate(x=w549) -> (-x=w548:dbl)
        n173 = call-poly <vilib>:"WPI_RobotDriveArcadeDrive.vi"("error in (no error)"=w551, "Y axis value"=w539, "X axis value"=w548, "RobotDriveDevRef"=w552) -> ()  [unwired: 5 in, 3 out]
      }
      n174 = while {
        tunnel: [w445] -> w336
        tunnel: w340 -> [w445]
        tunnel: [w444] -> w335
        tunnel: w339 -> [w444]
        tunnel: [w447] -> w334
        tunnel: w338 -> [w447]
        tunnel: [w446] -> w333
        tunnel: w337 -> [w446]
        i -> [w470]
        stop <- w466 stop-if-true
        n175 = global read "Robot Global Data.vi" "YAW"() -> (w455:dbl)
        n176 = call <vilib>:"WPI_RobotDriveRefNum Registry Get.vi"("refnum name"="RobotDrive") -> ("error out"=w453:errorcluster, "RobotDriveDevRef"=w454:T15)  [unwired: 9 in]
        n177 = Wait (ms)(milliseconds to wait=u32 20) -> ()  [unwired: 1 out]
        n178 = Increment(x=w470) -> (x+1=w469:i32)
        n179 = call-poly <vilib>:"PID.vi"("output range"=cluster{"output high":dbl, "output low":dbl} {"output high"=0.4, "output low"=-0.4}, "PID gains"=T7 {"proportional gain (Kc)"=0.11, "integral time (Ti, min)"=0.0, "derivative time (Td, min)"=0.0}, "process variable"=w455, "setpoint"=-25.0) -> ("output"=w449:dbl)  [unwired: 6 in, 1 out]
        n180 = Greater Or Equal?(x=w469, y=100) -> (x >= y?=w467:bool)
        n181 = Negate(x=w449) -> (-x=w448:dbl)
        n182 = call-poly <vilib>:"CTRE_Phoenix_MotorController_Get_Enhanced.vi"("PhoenixMotorControlDevRef"=w445, "error in"=w444) -> ("Quadrature Position"=w465:i32)  [unwired: 10 in, 3 out]
        n183 = To Double Precision Float(number=w465) -> (double precision float=w464:dbl)
        n184 = feedback #2() -> (w450:dbl)  [unwired: 1 in]
        n185 = call-poly <vilib>:"WPI_RobotDriveArcadeDrive.vi"("error in (no error)"=w453, "Y axis value"=w450, "X axis value"=w448, "RobotDriveDevRef"=w454) -> ()  [unwired: 5 in, 3 out]
        n186 = Absolute Value(x=w464) -> (abs(x)=w460:dbl)
        n187 = Greater Or Equal?(x=w460, y=115000.0 ("upper limit")) -> (x >= y?=w451:bool)
        n188 = And(x=w451, y=w467) -> (x .and. y?=w466:bool)
        n189 = Select(t=0.0, s=w451, f=-0.6) -> (s? t:f=w461:dbl)
        n190 = feedback-in #2(w461) -> ()
      }
      n191 = while {
        tunnel: w336 -> [w428]
        tunnel: w335 -> [w427]
        tunnel: w334 -> [w426]
        tunnel: w333 -> [w425]
        tunnel: [w428] -> w332
        tunnel: [w427] -> w331
        tunnel: [w426] -> w330
        tunnel: [w425] -> w329
        i -> [w437]
        stop <- w435 stop-if-true
        n192 = global read "Robot Global Data.vi" "YAW"() -> (w441:dbl)
        n193 = Increment(x=w437) -> (x+1=w439:i32)
        n194 = call-poly <vilib>:"PID.vi"("output range"=cluster{"output high":dbl, "output low":dbl} {"output high"=0.7, "output low"=-0.7}, "PID gains"=T7 {"proportional gain (Kc)"=0.045, "integral time (Ti, min)"=0.0, "derivative time (Td, min)"=0.0}, "process variable"=w441, "setpoint"=-90.0) -> ("output"=w430:dbl)  [unwired: 6 in, 1 out]
        n195 = call <vilib>:"WPI_RobotDriveRefNum Registry Get.vi"("refnum name"="RobotDrive") -> ("error out"=w433:errorcluster, "RobotDriveDevRef"=w434:T15)  [unwired: 9 in]
        n196 = Greater?(x=w439, y=200) -> (0:w435:bool)
        n197 = Negate(x=w430) -> (-x=w429:dbl)
        n198 = call-poly <vilib>:"WPI_RobotDriveArcadeDrive.vi"("error in (no error)"=w433, "Y axis value"=0.0, "X axis value"=w429, "RobotDriveDevRef"=w434) -> ()  [unwired: 5 in, 3 out]
        n199 = Wait (ms)(milliseconds to wait=u32 20) -> ()  [unwired: 1 out]
      }
      n200 = while {
        tunnel: [w502] -> w328
        tunnel: w332 -> [w502]
        tunnel: w331 -> [w501]
        tunnel: [w501] -> w327
        tunnel: [w504] -> w326
        tunnel: w330 -> [w504]
        tunnel: [w503] -> w325
        tunnel: w329 -> [w503]
        i -> [w528]
        stop <- w524 stop-if-true
        n201 = global read "Robot Global Data.vi" "YAW"() -> (w512:dbl)
        n202 = call <vilib>:"WPI_RobotDriveRefNum Registry Get.vi"("refnum name"="RobotDrive") -> ("error out"=w510:errorcluster, "RobotDriveDevRef"=w511:T15)  [unwired: 9 in]
        n203 = Increment(x=w528) -> (x+1=w527:i32)
        n204 = Wait (ms)(milliseconds to wait=u32 20) -> ()  [unwired: 1 out]
        n205 = call-poly <vilib>:"PID.vi"("output range"=cluster{"output high":dbl, "output low":dbl} {"output high"=0.4, "output low"=-0.4}, "PID gains"=T7 {"proportional gain (Kc)"=0.11, "integral time (Ti, min)"=0.0, "derivative time (Td, min)"=0.0}, "process variable"=w512, "setpoint"=0.0) -> ("output"=w508:dbl)  [unwired: 6 in, 1 out]
        n206 = Greater Or Equal?(x=w527, y=20) -> (x >= y?=w525:bool)
        n207 = Negate(x=w508) -> (-x=w507:dbl)
        n208 = Wait (ms)(milliseconds to wait=u32 20) -> ()  [unwired: 1 out]
        n209 = call-poly <vilib>:"CTRE_Phoenix_MotorController_Get_Enhanced.vi"("PhoenixMotorControlDevRef"=w502, "error in"=w501) -> ("Quadrature Position"=w523:i32)  [unwired: 10 in, 3 out]
        n210 = To Double Precision Float(number=w523) -> (double precision float=w522:dbl)
        n211 = feedback #3() -> (w506:dbl)  [unwired: 1 in]
        n212 = call-poly <vilib>:"WPI_RobotDriveArcadeDrive.vi"("error in (no error)"=w510, "Y axis value"=w506, "X axis value"=w507, "RobotDriveDevRef"=w511) -> ()  [unwired: 5 in, 3 out]
        n213 = Absolute Value(x=w522) -> (abs(x)=w518:dbl)
        n214 = Greater Or Equal?(x=w518, y=113500.0 ("upper limit")) -> (x >= y?=w516:bool)
        n215 = And(x=w516, y=w525) -> (x .and. y?=w524:bool)
        n216 = Select(t=0.0, s=w516, f=-0.6) -> (s? t:f=w519:dbl)
        n217 = feedback-in #3(w519) -> ()
      }
      n218 = while {
        tunnel: [w390] -> _
        tunnel: w328 -> [w390]
        tunnel: [w389] -> _
        tunnel: w327 -> [w389]
        tunnel: [w388] -> _
        tunnel: w326 -> [w388]
        tunnel: [w387] -> _
        tunnel: w325 -> [w387]
        i -> [w414]
        stop <- w391 stop-if-true
        # "Set config to shoot level, Rev, Shoot, and reset"
        n219 = global read "Robot Global Data.vi" "Pot 1"() -> (w419:dbl)
        n220 = call <vilib>:"WPI_MotorControlRefNum Registry Get.vi"("refnum name"="Acquire") -> ("error out"=w416:errorcluster, "MotorControlDevRef"=w417:T8)  [unwired: 9 in]
        n221 = call <vilib>:"WPI_MotorControlRefNum Registry Get.vi"("refnum name"="Dart 1") -> ("error out"=w423:errorcluster, "MotorControlDevRef"=w422:T8)  [unwired: 9 in]
        n222 = Increment(x=w414) -> (x+1=w415:i32)
        n223 = call-poly <vilib>:"PID.vi"("PID gains"=T7 {"proportional gain (Kc)"=1.0, "integral time (Ti, min)"=0.01, "derivative time (Td, min)"=0.0}, "process variable"=w419, "setpoint"=0.0) -> ("output"=w424:dbl)  [unwired: 7 in, 1 out]
        n224 = Greater Or Equal?(x=w415, y=100) -> (x >= y?=w406:bool)
        n225 = call <vilib>:"WPI_MotorControlSetOutput.vi"("error in (no error)"=w423, "Output"=w424, "MotorControlDevRef"=w422) -> ()  [unwired: 6 in, 3 out]
        n226 = call <vilib>:"WPI_MotorControlSetOutput.vi"("error in (no error)"=w416, "Output"=-1.0, "MotorControlDevRef"=w417) -> ()  [unwired: 6 in, 3 out]
        n227 = Select(t=WPI_SolenoidValue."Forward" ("Value"), s=w406, f=WPI_SolenoidValue."Off" ("Value")) -> (s? t:f=w409:T6)
        n228 = Wait (ms)(milliseconds to wait=u32 20) -> ()  [unwired: 1 out]
        n229 = call <vilib>:"WPI_SolenoidRefNum Registry Get.vi"("refnum name"="Push") -> ("error out"=w410:errorcluster, "SolenoidDevRef"=w411:T16)  [unwired: 9 in]
        n230 = call-poly <vilib>:"WPI_SolenoidSet.vi"("error in (no error)"=w410, "Value"=w409, "SolenoidDevRef"=w411) -> ("error out"=w402:errorcluster, "SolenoidDevRef"=w403:T16)  [unwired: 7 in]
        n231 = call-poly <vilib>:"WPI_SolenoidGet.vi"("error in (no error)"=w402, "SolenoidDevRef"=w403) -> ("Value"=w401:bool)  [unwired: 7 in, 2 out]
        n232 = And(x=w406, y=w401) -> (x .and. y?=w392:bool)
        n233 = Select(t=WPI_SolenoidValue."Reverse" ("Value"), s=w392, f=WPI_SolenoidValue."Off" ("Value")) -> (s? t:f=w397:T6)
        n234 = call <vilib>:"WPI_SolenoidRefNum Registry Get.vi"("refnum name"="Push") -> ("error out"=w398:errorcluster, "SolenoidDevRef"=w399:T16)  [unwired: 9 in]
        n235 = call-poly <vilib>:"WPI_SolenoidSet.vi"("error in (no error)"=w398, "Value"=w397, "SolenoidDevRef"=w399) -> ("error out"=w393:errorcluster, "SolenoidDevRef"=w394:T16)  [unwired: 7 in]
        n236 = call-poly <vilib>:"WPI_SolenoidGet.vi"("error in (no error)"=w393, "SolenoidDevRef"=w394) -> ("Value"=w391:bool)  [unwired: 7 in, 2 out]
      }
    }
    frame "Place 2 Scale Right" {
      # "Done"
      n237 = call <vilib>:"WPI_MotorControlRefNum Registry Get.vi"("refnum name"="Left Lead") -> ("error out"=w651:errorcluster, "MotorControlDevRef"=w652:T8)  [unwired: 9 in]
      n238 = call <vilib>:"WPI_MotorControlRefNum Registry Get.vi"("refnum name"="Right Lead") -> ("error out"=w649:errorcluster, "MotorControlDevRef"=w650:T8)  [unwired: 9 in]
      n239 = while {
        tunnel: w652 -> [w934]
        tunnel: w651 -> [w933]
        tunnel: w650 -> [w932]
        tunnel: w649 -> [w931]
        tunnel: [w934] -> w692
        tunnel: [w933] -> w691
        tunnel: [w932] -> w690
        tunnel: [w931] -> w689
        i -> [w944]
        stop <- w943 stop-if-true
        n240 = Increment(x=w944) -> (x+1=w946:i32)
        n241 = Greater?(x=w946, y=10) -> (0:w943:bool)
        n242 = call <vilib>:"CTRE_PigeonIMU_RefNumRegistryGet.vi"("refnum name"="Pigeon") -> ("PigeonIMUDevRef"=w941:T13)  [unwired: 9 in, 1 out]
        n243 = call-poly <vilib>:"CTRE_Phoenix_MotorController_Get_Enhanced.vi"("PhoenixMotorControlDevRef"=w934, "error in"=w933) -> ("PhoenixMotorControlDevRef"=w936:T8)  [unwired: 10 in, 3 out]
        n244 = call-poly <vilib>:"CTRE_Phoenix_MotorController_Get_Enhanced.vi"("PhoenixMotorControlDevRef"=w932, "error in"=w931) -> ("PhoenixMotorControlDevRef"=w935:T8)  [unwired: 10 in, 3 out]
        n245 = call "CTRE_Phoenix_MotorControl_SetQuadraturePosition_Enhanced.vi"("New Position"=0, "PhoenixMotorControlDevRef"=w935) -> ()  [unwired: 8 in, 2 out]
        n246 = call "CTRE_Phoenix_MotorControl_SetQuadraturePosition_Enhanced.vi"("New Position"=0, "PhoenixMotorControlDevRef"=w936) -> ()  [unwired: 8 in, 2 out]
        n247 = Wait (ms)(milliseconds to wait=u32 20) -> ()  [unwired: 1 out]
        n248 = call <vilib>:"CTRE_PigeonIMU_SetYaw.vi"("Value"=0.0, "PigeonIMUDevRef"=w941) -> ()  [unwired: 8 in, 2 out]
      }
      n249 = while {
        tunnel: [w949] -> w688
        tunnel: w692 -> [w949]
        tunnel: [w950] -> w687
        tunnel: w691 -> [w950]
        tunnel: [w957] -> w686
        tunnel: w690 -> [w957]
        tunnel: [w956] -> w685
        tunnel: w689 -> [w956]
        i -> [w973]
        stop <- w969 stop-if-true
        n250 = global read "Robot Global Data.vi" "YAW"() -> (w958:dbl)
        n251 = Wait (ms)(milliseconds to wait=u32 20) -> ()  [unwired: 1 out]
        n252 = call <vilib>:"WPI_RobotDriveRefNum Registry Get.vi"("refnum name"="RobotDrive") -> ("error out"=w954:errorcluster, "RobotDriveDevRef"=w955:T15)  [unwired: 9 in]
        n253 = Increment(x=w973) -> (x+1=w972:i32)
        n254 = call-poly <vilib>:"PID.vi"("output range"=cluster{"output high":dbl, "output low":dbl} {"output high"=0.4, "output low"=-0.4}, "PID gains"=T7 {"proportional gain (Kc)"=0.11, "integral time (Ti, min)"=0.0, "derivative time (Td, min)"=0.0}, "process variable"=w958, "setpoint"=0.0) -> ("output"=w948:dbl)  [unwired: 6 in, 1 out]
        n255 = Greater Or Equal?(x=w972, y=100) -> (x >= y?=w970:bool)
        n256 = Negate(x=w948) -> (-x=w947:dbl)
        n257 = call-poly <vilib>:"CTRE_Phoenix_MotorController_Get_Enhanced.vi"("PhoenixMotorControlDevRef"=w949, "error in"=w950) -> ("Quadrature Position"=w968:i32)  [unwired: 10 in, 3 out]
        n258 = To Double Precision Float(number=w968) -> (double precision float=w967:dbl)
        n259 = feedback #4() -> (w951:dbl)  [unwired: 1 in]
        n260 = call-poly <vilib>:"WPI_RobotDriveArcadeDrive.vi"("error in (no error)"=w954, "Y axis value"=w951, "X axis value"=w947, "RobotDriveDevRef"=w955) -> ()  [unwired: 5 in, 3 out]
        n261 = Absolute Value(x=w967) -> (abs(x)=w963:dbl)
        n262 = Greater Or Equal?(x=w963, y=115000.0 ("upper limit")) -> (x >= y?=w952:bool)
        n263 = And(x=w952, y=w970) -> (x .and. y?=w969:bool)
        n264 = Select(t=0.0, s=w952, f=-0.8) -> (s? t:f=w964:dbl)
        n265 = feedback-in #4(w964) -> ()
      }
      n266 = while {
        tunnel: w688 -> [w921]
        tunnel: w687 -> [w920]
        tunnel: w686 -> [w919]
        tunnel: w685 -> [w918]
        tunnel: [w921] -> w684
        tunnel: [w920] -> w683
        tunnel: [w919] -> w682
        tunnel: [w918] -> w681
        i -> [w924]
        stop <- w922 stop-if-true
        n267 = global read "Robot Global Data.vi" "YAW"() -> (w928:dbl)
        n268 = Increment(x=w924) -> (x+1=w926:i32)
        n269 = call-poly <vilib>:"PID.vi"("output range"=cluster{"output high":dbl, "output low":dbl} {"output high"=0.7, "output low"=-0.7}, "PID gains"=T7 {"proportional gain (Kc)"=0.045, "integral time (Ti, min)"=0.0, "derivative time (Td, min)"=0.0}, "process variable"=w928, "setpoint"=90.0) -> ("output"=w913:dbl)  [unwired: 6 in, 1 out]
        n270 = call <vilib>:"WPI_RobotDriveRefNum Registry Get.vi"("refnum name"="RobotDrive") -> ("error out"=w916:errorcluster, "RobotDriveDevRef"=w917:T15)  [unwired: 9 in]
        n271 = Greater?(x=w926, y=200) -> (0:w922:bool)
        n272 = Negate(x=w913) -> (-x=w912:dbl)
        n273 = call-poly <vilib>:"WPI_RobotDriveArcadeDrive.vi"("error in (no error)"=w916, "Y axis value"=0.0, "X axis value"=w912, "RobotDriveDevRef"=w917) -> ()  [unwired: 5 in, 3 out]
        n274 = Wait (ms)(milliseconds to wait=u32 20) -> ()  [unwired: 1 out]
      }
      n275 = while {
        tunnel: [w821] -> w680
        tunnel: w684 -> [w821]
        tunnel: [w820] -> w679
        tunnel: w683 -> [w820]
        tunnel: [w819] -> w678
        tunnel: w682 -> [w819]
        tunnel: [w822] -> w677
        tunnel: w681 -> [w822]
        i -> [w815]
        stop <- w801 stop-if-true
        # "Set config to shoot level, Rev, Shoot"
        n276 = global read "Robot Global Data.vi" "Pot 1"() -> (w823:dbl)
        n277 = call <vilib>:"WPI_MotorControlRefNum Registry Get.vi"("refnum name"="Acquire") -> ("error out"=w816:errorcluster, "MotorControlDevRef"=w817:T8)  [unwired: 9 in]
        n278 = call <vilib>:"WPI_MotorControlRefNum Registry Get.vi"("refnum name"="Dart 1") -> ("error out"=w827:errorcluster, "MotorControlDevRef"=w826:T8)  [unwired: 9 in]
        n279 = Increment(x=w815) -> (x+1=w802:i32)
        n280 = call-poly <vilib>:"PID.vi"("PID gains"=T7 {"proportional gain (Kc)"=1.0, "integral time (Ti, min)"=0.01, "derivative time (Td, min)"=0.0}, "process variable"=w823, "setpoint"=0.0) -> ("output"=w828:dbl)  [unwired: 7 in, 1 out]
        n281 = Greater Or Equal?(x=w802, y=100) -> (x >= y?=w807:bool)
        n282 = call <vilib>:"WPI_MotorControlSetOutput.vi"("error in (no error)"=w827, "Output"=w828, "MotorControlDevRef"=w826) -> ()  [unwired: 6 in, 3 out]
        n283 = call <vilib>:"WPI_MotorControlSetOutput.vi"("error in (no error)"=w816, "Output"=-1.0, "MotorControlDevRef"=w817) -> ()  [unwired: 6 in, 3 out]
        n284 = Select(t=WPI_SolenoidValue."Forward" ("Value"), s=w807, f=WPI_SolenoidValue."Off" ("Value")) -> (s? t:f=w810:T6)
        n285 = Wait (ms)(milliseconds to wait=u32 20) -> ()  [unwired: 1 out]
        n286 = call <vilib>:"WPI_SolenoidRefNum Registry Get.vi"("refnum name"="Push") -> ("error out"=w811:errorcluster, "SolenoidDevRef"=w812:T16)  [unwired: 9 in]
        n287 = call-poly <vilib>:"WPI_SolenoidSet.vi"("error in (no error)"=w811, "Value"=w810, "SolenoidDevRef"=w812) -> ("error out"=w803:errorcluster, "SolenoidDevRef"=w804:T16)  [unwired: 7 in]
        n288 = call-poly <vilib>:"WPI_SolenoidGet.vi"("error in (no error)"=w803, "SolenoidDevRef"=w804) -> ("Value"=w801:bool)  [unwired: 7 in, 2 out]
      }
      n289 = while {
        tunnel: w680 -> [w707]
        tunnel: w679 -> [w706]
        tunnel: w678 -> [w705]
        tunnel: w677 -> [w704]
        tunnel: [w707] -> w676
        tunnel: [w706] -> w675
        tunnel: [w705] -> w674
        tunnel: [w704] -> w673
        i -> [w695]
        stop <- w694 stop-if-true
        # "Reset"
        n290 = call <vilib>:"WPI_SolenoidRefNum Registry Get.vi"("refnum name"="Push") -> ("error out"=w711:errorcluster, "SolenoidDevRef"=w712:T16)  [unwired: 9 in]
        n291 = call <vilib>:"WPI_MotorControlRefNum Registry Get.vi"("refnum name"="Dart 1") -> ("error out"=w702:errorcluster, "MotorControlDevRef"=w701:T8)  [unwired: 9 in]
        n292 = Increment(x=w695) -> (x+1=w708:i32)
        n293 = global read "Robot Global Data.vi" "Pot 1"() -> (w698:dbl)
        n294 = Greater Or Equal?(x=w708, y=100) -> (x >= y?=w694:bool)
        n295 = call-poly <vilib>:"PID.vi"("PID gains"=T7 {"proportional gain (Kc)"=1.0, "integral time (Ti, min)"=0.01, "derivative time (Td, min)"=0.0}, "process variable"=w698, "setpoint"=0.0) -> ("output"=w703:dbl)  [unwired: 7 in, 1 out]
        n296 = call <vilib>:"WPI_MotorControlSetOutput.vi"("error in (no error)"=w702, "Output"=w703, "MotorControlDevRef"=w701) -> ()  [unwired: 6 in, 3 out]
        n297 = call-poly <vilib>:"WPI_SolenoidSet.vi"("error in (no error)"=w711, "Value"=WPI_SolenoidValue."Reverse", "SolenoidDevRef"=w712) -> ("error out"=w709:errorcluster, "SolenoidDevRef"=w710:T16)  [unwired: 7 in]
        n298 = call-poly <vilib>:"WPI_SolenoidGet.vi"("error in (no error)"=w709, "SolenoidDevRef"=w710) -> ()  [unwired: 7 in, 3 out]
      }
      n299 = while {
        tunnel: [w892] -> w672
        tunnel: w676 -> [w892]
        tunnel: [w891] -> w671
        tunnel: w675 -> [w891]
        tunnel: [w890] -> w670
        tunnel: w674 -> [w890]
        tunnel: [w889] -> w669
        tunnel: w673 -> [w889]
        i -> [w905]
        stop <- w903 stop-if-true
        n300 = global read "Robot Global Data.vi" "YAW"() -> (w909:dbl)
        n301 = Increment(x=w905) -> (x+1=w907:i32)
        n302 = call-poly <vilib>:"PID.vi"("output range"=cluster{"output high":dbl, "output low":dbl} {"output high"=0.6, "output low"=-0.6}, "PID gains"=T7 {"proportional gain (Kc)"=0.055, "integral time (Ti, min)"=0.0, "derivative time (Td, min)"=0.0}, "process variable"=w909, "setpoint"=25.0) -> ("output"=w899:dbl)  [unwired: 6 in, 1 out]
        n303 = call <vilib>:"WPI_RobotDriveRefNum Registry Get.vi"("refnum name"="RobotDrive") -> ("error out"=w900:errorcluster, "RobotDriveDevRef"=w901:T15)  [unwired: 9 in]
        n304 = Negate(x=w899) -> (-x=w898:dbl)
        n305 = Greater?(x=w907, y=180) -> (0:w903:bool)
        n306 = call-poly <vilib>:"WPI_RobotDriveArcadeDrive.vi"("error in (no error)"=w900, "Y axis value"=0.0, "X axis value"=w898, "RobotDriveDevRef"=w901) -> ()  [unwired: 5 in, 3 out]
        n307 = Wait (ms)(milliseconds to wait=u32 20) -> ()  [unwired: 1 out]
        n308 = call-poly <vilib>:"CTRE_Phoenix_MotorController_Get_Enhanced.vi"("PhoenixMotorControlDevRef"=w892, "error in"=w891) -> ("PhoenixMotorControlDevRef"=w894:T8)  [unwired: 8 in, 5 out]
        n309 = call-poly <vilib>:"CTRE_Phoenix_MotorController_Get_Enhanced.vi"("PhoenixMotorControlDevRef"=w890, "error in"=w889) -> ("PhoenixMotorControlDevRef"=w893:T8)  [unwired: 8 in, 5 out]
        n310 = call "CTRE_Phoenix_MotorControl_SetQuadraturePosition_Enhanced.vi"("New Position"=0, "PhoenixMotorControlDevRef"=w893) -> ()  [unwired: 8 in, 2 out]
        n311 = call "CTRE_Phoenix_MotorControl_SetQuadraturePosition_Enhanced.vi"("New Position"=0, "PhoenixMotorControlDevRef"=w894) -> ()  [unwired: 8 in, 2 out]
      }
      n312 = while {
        tunnel: [w862] -> w668
        tunnel: w672 -> [w862]
        tunnel: [w861] -> w667
        tunnel: w671 -> [w861]
        tunnel: [w860] -> w666
        tunnel: w670 -> [w860]
        tunnel: [w859] -> w665
        tunnel: w669 -> [w859]
        i -> [w887]
        stop <- w883 stop-if-true
        # "Drives towards cube, uses pixy cam's \"x\" value to stay on center"
        n313 = Increment(x=w887) -> (x+1=w886:i32)
        n314 = Greater Or Equal?(x=w886, y=100) -> (x >= y?=w884:bool)
        n315 = call <vilib>:"WPI_DigitalInputRefNum Registry Get.vi"("refnum name"="Color Mark") -> ("DigitalInputDevRef"=w873:T18)  [unwired: 9 in, 1 out]
        n316 = call <vilib>:"WPI_MotorControlRefNum Registry Get.vi"("refnum name"="Acquire") -> ("error out"=w870:errorcluster, "MotorControlDevRef"=w871:T8)  [unwired: 9 in]
        n317 = call <vilib>:"WPI_DigitalInputGetValue.vi"("DigitalInputDevRef"=w873) -> ("Value"=w863:bool)  [unwired: 8 in, 2 out]
        n318 = And(x=w863, y=w884) -> (x .and. y?=w883:bool)
        n319 = Wait (ms)(milliseconds to wait=u32 20) -> ()  [unwired: 1 out]
        n320 = Select(t=0.0, s=w863, f=0.6) -> (s? t:f=w864:dbl)
        n321 = Select(t=0.0, s=w863, f=0.6) -> (s? t:f=w867:dbl)
        n322 = call <vilib>:"WPI_MotorControlSetOutput.vi"("error in (no error)"=w870, "Output"=w864, "MotorControlDevRef"=w871) -> ()  [unwired: 6 in, 3 out]
        n323 = call "PIXY VI.vi"() -> ("X"=w874:dbl)  [unwired: 14 in, 5 out]
        n324 = call <vilib>:"WPI_RobotDriveRefNum Registry Get.vi"("refnum name"="RobotDrive") -> ("error out"=w879:errorcluster, "RobotDriveDevRef"=w880:T15)  [unwired: 9 in]
        n325 = call-poly <vilib>:"PID.vi"("output range"=cluster{"output high":dbl, "output low":dbl} {"output high"=0.4, "output low"=-0.4}, "PID gains"=T7 {"proportional gain (Kc)"=0.11, "integral time (Ti, min)"=0.0, "derivative time (Td, min)"=0.0}, "process variable"=w874, "setpoint"=0.0) -> ("output"=w877:dbl)  [unwired: 6 in, 1 out]
        n326 = Negate(x=w877) -> (-x=w876:dbl)
        n327 = call-poly <vilib>:"WPI_RobotDriveArcadeDrive.vi"("error in (no error)"=w879, "Y axis value"=w867, "X axis value"=w876, "RobotDriveDevRef"=w880) -> ()  [unwired: 5 in, 3 out]
      }
      n328 = while {
        tunnel: [w773] -> w664
        tunnel: w668 -> [w773]
        tunnel: [w772] -> w663
        tunnel: w667 -> [w772]
        tunnel: [w775] -> w662
        tunnel: w666 -> [w775]
        tunnel: [w774] -> w661
        tunnel: w665 -> [w774]
        i -> [w798]
        stop <- w794 stop-if-true
        n329 = global read "Robot Global Data.vi" "YAW"() -> (w783:dbl)
        n330 = call <vilib>:"WPI_RobotDriveRefNum Registry Get.vi"("refnum name"="RobotDrive") -> ("error out"=w781:errorcluster, "RobotDriveDevRef"=w782:T15)  [unwired: 9 in]
        n331 = Wait (ms)(milliseconds to wait=u32 20) -> ()  [unwired: 1 out]
        n332 = Increment(x=w798) -> (x+1=w797:i32)
        n333 = call-poly <vilib>:"PID.vi"("output range"=cluster{"output high":dbl, "output low":dbl} {"output high"=0.4, "output low"=-0.4}, "PID gains"=T7 {"proportional gain (Kc)"=0.11, "integral time (Ti, min)"=0.0, "derivative time (Td, min)"=0.0}, "process variable"=w783, "setpoint"=25.0) -> ("output"=w777:dbl)  [unwired: 6 in, 1 out]
        n334 = Greater Or Equal?(x=w797, y=100) -> (x >= y?=w795:bool)
        n335 = Negate(x=w777) -> (-x=w776:dbl)
        n336 = call-poly <vilib>:"CTRE_Phoenix_MotorController_Get_Enhanced.vi"("PhoenixMotorControlDevRef"=w773, "error in"=w772) -> ("Quadrature Position"=w793:i32)  [unwired: 10 in, 3 out]
        n337 = To Double Precision Float(number=w793) -> (double precision float=w792:dbl)
        n338 = feedback #5() -> (w778:dbl)  [unwired: 1 in]
        n339 = call-poly <vilib>:"WPI_RobotDriveArcadeDrive.vi"("error in (no error)"=w781, "Y axis value"=w778, "X axis value"=w776, "RobotDriveDevRef"=w782) -> ()  [unwired: 5 in, 3 out]
        n340 = Absolute Value(x=w792) -> (abs(x)=w788:dbl)
        n341 = Greater Or Equal?(x=w788, y=115000.0 ("upper limit")) -> (x >= y?=w779:bool)
        n342 = And(x=w779, y=w795) -> (x .and. y?=w794:bool)
        n343 = Select(t=0.0, s=w779, f=-0.6) -> (s? t:f=w789:dbl)
        n344 = feedback-in #5(w789) -> ()
      }
      n345 = while {
        tunnel: w664 -> [w756]
        tunnel: w663 -> [w755]
        tunnel: w662 -> [w754]
        tunnel: w661 -> [w753]
        tunnel: [w756] -> w660
        tunnel: [w755] -> w659
        tunnel: [w754] -> w658
        tunnel: [w753] -> w657
        i -> [w765]
        stop <- w763 stop-if-true
        n346 = global read "Robot Global Data.vi" "YAW"() -> (w769:dbl)
        n347 = Increment(x=w765) -> (x+1=w767:i32)
        n348 = call-poly <vilib>:"PID.vi"("output range"=cluster{"output high":dbl, "output low":dbl} {"output high"=0.7, "output low"=-0.7}, "PID gains"=T7 {"proportional gain (Kc)"=0.045, "integral time (Ti, min)"=0.0, "derivative time (Td, min)"=0.0}, "process variable"=w769, "setpoint"=90.0) -> ("output"=w758:dbl)  [unwired: 6 in, 1 out]
        n349 = call <vilib>:"WPI_RobotDriveRefNum Registry Get.vi"("refnum name"="RobotDrive") -> ("error out"=w761:errorcluster, "RobotDriveDevRef"=w762:T15)  [unwired: 9 in]
        n350 = Greater?(x=w767, y=200) -> (0:w763:bool)
        n351 = Negate(x=w758) -> (-x=w757:dbl)
        n352 = call-poly <vilib>:"WPI_RobotDriveArcadeDrive.vi"("error in (no error)"=w761, "Y axis value"=0.0, "X axis value"=w757, "RobotDriveDevRef"=w762) -> ()  [unwired: 5 in, 3 out]
        n353 = Wait (ms)(milliseconds to wait=u32 20) -> ()  [unwired: 1 out]
      }
      n354 = while {
        tunnel: [w830] -> w656
        tunnel: w660 -> [w830]
        tunnel: w659 -> [w829]
        tunnel: [w829] -> w655
        tunnel: [w832] -> w654
        tunnel: w658 -> [w832]
        tunnel: [w831] -> w653
        tunnel: w657 -> [w831]
        i -> [w856]
        stop <- w852 stop-if-true
        n355 = global read "Robot Global Data.vi" "YAW"() -> (w840:dbl)
        n356 = call <vilib>:"WPI_RobotDriveRefNum Registry Get.vi"("refnum name"="RobotDrive") -> ("error out"=w838:errorcluster, "RobotDriveDevRef"=w839:T15)  [unwired: 9 in]
        n357 = Increment(x=w856) -> (x+1=w855:i32)
        n358 = Wait (ms)(milliseconds to wait=u32 20) -> ()  [unwired: 1 out]
        n359 = call-poly <vilib>:"PID.vi"("output range"=cluster{"output high":dbl, "output low":dbl} {"output high"=0.4, "output low"=-0.4}, "PID gains"=T7 {"proportional gain (Kc)"=0.11, "integral time (Ti, min)"=0.0, "derivative time (Td, min)"=0.0}, "process variable"=w840, "setpoint"=0.0) -> ("output"=w836:dbl)  [unwired: 6 in, 1 out]
        n360 = Greater Or Equal?(x=w855, y=20) -> (x >= y?=w853:bool)
        n361 = Negate(x=w836) -> (-x=w835:dbl)
        n362 = Wait (ms)(milliseconds to wait=u32 20) -> ()  [unwired: 1 out]
        n363 = call-poly <vilib>:"CTRE_Phoenix_MotorController_Get_Enhanced.vi"("PhoenixMotorControlDevRef"=w830, "error in"=w829) -> ("Quadrature Position"=w851:i32)  [unwired: 10 in, 3 out]
        n364 = To Double Precision Float(number=w851) -> (double precision float=w850:dbl)
        n365 = feedback #6() -> (w834:dbl)  [unwired: 1 in]
        n366 = call-poly <vilib>:"WPI_RobotDriveArcadeDrive.vi"("error in (no error)"=w838, "Y axis value"=w834, "X axis value"=w835, "RobotDriveDevRef"=w839) -> ()  [unwired: 5 in, 3 out]
        n367 = Absolute Value(x=w850) -> (abs(x)=w846:dbl)
        n368 = Greater Or Equal?(x=w846, y=113500.0 ("upper limit")) -> (x >= y?=w844:bool)
        n369 = And(x=w844, y=w853) -> (x .and. y?=w852:bool)
        n370 = Select(t=0.0, s=w844, f=-0.6) -> (s? t:f=w847:dbl)
        n371 = feedback-in #6(w847) -> ()
      }
      n372 = while {
        tunnel: [w718] -> _
        tunnel: w656 -> [w718]
        tunnel: [w717] -> _
        tunnel: w655 -> [w717]
        tunnel: [w716] -> _
        tunnel: w654 -> [w716]
        tunnel: [w715] -> _
        tunnel: w653 -> [w715]
        i -> [w742]
        stop <- w719 stop-if-true
        # "Set config to shoot level, Rev, Shoot, and reset"
        n373 = global read "Robot Global Data.vi" "Pot 1"() -> (w747:dbl)
        n374 = call <vilib>:"WPI_MotorControlRefNum Registry Get.vi"("refnum name"="Acquire") -> ("error out"=w744:errorcluster, "MotorControlDevRef"=w745:T8)  [unwired: 9 in]
        n375 = call <vilib>:"WPI_MotorControlRefNum Registry Get.vi"("refnum name"="Dart 1") -> ("error out"=w751:errorcluster, "MotorControlDevRef"=w750:T8)  [unwired: 9 in]
        n376 = Increment(x=w742) -> (x+1=w743:i32)
        n377 = call-poly <vilib>:"PID.vi"("PID gains"=T7 {"proportional gain (Kc)"=1.0, "integral time (Ti, min)"=0.01, "derivative time (Td, min)"=0.0}, "process variable"=w747, "setpoint"=0.0) -> ("output"=w752:dbl)  [unwired: 7 in, 1 out]
        n378 = Greater Or Equal?(x=w743, y=100) -> (x >= y?=w734:bool)
        n379 = call <vilib>:"WPI_MotorControlSetOutput.vi"("error in (no error)"=w751, "Output"=w752, "MotorControlDevRef"=w750) -> ()  [unwired: 6 in, 3 out]
        n380 = call <vilib>:"WPI_MotorControlSetOutput.vi"("error in (no error)"=w744, "Output"=-1.0, "MotorControlDevRef"=w745) -> ()  [unwired: 6 in, 3 out]
        n381 = Select(t=WPI_SolenoidValue."Forward" ("Value"), s=w734, f=WPI_SolenoidValue."Off" ("Value")) -> (s? t:f=w737:T6)
        n382 = Wait (ms)(milliseconds to wait=u32 20) -> ()  [unwired: 1 out]
        n383 = call <vilib>:"WPI_SolenoidRefNum Registry Get.vi"("refnum name"="Push") -> ("error out"=w738:errorcluster, "SolenoidDevRef"=w739:T16)  [unwired: 9 in]
        n384 = call-poly <vilib>:"WPI_SolenoidSet.vi"("error in (no error)"=w738, "Value"=w737, "SolenoidDevRef"=w739) -> ("error out"=w730:errorcluster, "SolenoidDevRef"=w731:T16)  [unwired: 7 in]
        n385 = call-poly <vilib>:"WPI_SolenoidGet.vi"("error in (no error)"=w730, "SolenoidDevRef"=w731) -> ("Value"=w729:bool)  [unwired: 7 in, 2 out]
        n386 = And(x=w734, y=w729) -> (x .and. y?=w720:bool)
        n387 = Select(t=WPI_SolenoidValue."Reverse" ("Value"), s=w720, f=WPI_SolenoidValue."Off" ("Value")) -> (s? t:f=w725:T6)
        n388 = call <vilib>:"WPI_SolenoidRefNum Registry Get.vi"("refnum name"="Push") -> ("error out"=w726:errorcluster, "SolenoidDevRef"=w727:T16)  [unwired: 9 in]
        n389 = call-poly <vilib>:"WPI_SolenoidSet.vi"("error in (no error)"=w726, "Value"=w725, "SolenoidDevRef"=w727) -> ("error out"=w721:errorcluster, "SolenoidDevRef"=w722:T16)  [unwired: 7 in]
        n390 = call-poly <vilib>:"WPI_SolenoidGet.vi"("error in (no error)"=w721, "SolenoidDevRef"=w722) -> ("Value"=w719:bool)  [unwired: 7 in, 2 out]
      }
    }
    frame "Place Scale Right" {
      # "done"
      n391 = call <vilib>:"WPI_MotorControlRefNum Registry Get.vi"("refnum name"="Left Lead") -> ("error out"=w979:errorcluster, "MotorControlDevRef"=w980:T8)  [unwired: 9 in]
      n392 = call <vilib>:"WPI_MotorControlRefNum Registry Get.vi"("refnum name"="Right Lead") -> ("error out"=w977:errorcluster, "MotorControlDevRef"=w978:T8)  [unwired: 9 in]
      n393 = while {
        tunnel: w980 -> [w1069]
        tunnel: w979 -> [w1068]
        tunnel: w978 -> [w1067]
        tunnel: w977 -> [w1066]
        tunnel: [w1069] -> w996
        tunnel: [w1068] -> w995
        tunnel: [w1067] -> w994
        tunnel: [w1066] -> w993
        i -> [w1079]
        stop <- w1078 stop-if-true
        n394 = Increment(x=w1079) -> (x+1=w1081:i32)
        n395 = Greater?(x=w1081, y=10) -> (0:w1078:bool)
        n396 = call <vilib>:"CTRE_PigeonIMU_RefNumRegistryGet.vi"("refnum name"="Pigeon") -> ("PigeonIMUDevRef"=w1076:T13)  [unwired: 9 in, 1 out]
        n397 = call-poly <vilib>:"CTRE_Phoenix_MotorController_Get_Enhanced.vi"("PhoenixMotorControlDevRef"=w1069, "error in"=w1068) -> ("PhoenixMotorControlDevRef"=w1071:T8)  [unwired: 10 in, 3 out]
        n398 = call-poly <vilib>:"CTRE_Phoenix_MotorController_Get_Enhanced.vi"("PhoenixMotorControlDevRef"=w1067, "error in"=w1066) -> ("PhoenixMotorControlDevRef"=w1070:T8)  [unwired: 10 in, 3 out]
        n399 = call "CTRE_Phoenix_MotorControl_SetQuadraturePosition_Enhanced.vi"("New Position"=0, "PhoenixMotorControlDevRef"=w1070) -> ()  [unwired: 8 in, 2 out]
        n400 = call "CTRE_Phoenix_MotorControl_SetQuadraturePosition_Enhanced.vi"("New Position"=0, "PhoenixMotorControlDevRef"=w1071) -> ()  [unwired: 8 in, 2 out]
        n401 = Wait (ms)(milliseconds to wait=u32 20) -> ()  [unwired: 1 out]
        n402 = call <vilib>:"CTRE_PigeonIMU_SetYaw.vi"("Value"=0.0, "PigeonIMUDevRef"=w1076) -> ()  [unwired: 8 in, 2 out]
      }
      n403 = while {
        tunnel: [w1084] -> w992
        tunnel: w996 -> [w1084]
        tunnel: [w1085] -> w991
        tunnel: w995 -> [w1085]
        tunnel: [w1092] -> w990
        tunnel: w994 -> [w1092]
        tunnel: [w1091] -> w989
        tunnel: w993 -> [w1091]
        i -> [w1108]
        stop <- w1104 stop-if-true
        n404 = global read "Robot Global Data.vi" "YAW"() -> (w1093:dbl)
        n405 = Wait (ms)(milliseconds to wait=u32 20) -> ()  [unwired: 1 out]
        n406 = call <vilib>:"WPI_RobotDriveRefNum Registry Get.vi"("refnum name"="RobotDrive") -> ("error out"=w1089:errorcluster, "RobotDriveDevRef"=w1090:T15)  [unwired: 9 in]
        n407 = Increment(x=w1108) -> (x+1=w1107:i32)
        n408 = call-poly <vilib>:"PID.vi"("output range"=cluster{"output high":dbl, "output low":dbl} {"output high"=0.4, "output low"=-0.4}, "PID gains"=T7 {"proportional gain (Kc)"=0.11, "integral time (Ti, min)"=0.0, "derivative time (Td, min)"=0.0}, "process variable"=w1093, "setpoint"=0.0) -> ("output"=w1083:dbl)  [unwired: 6 in, 1 out]
        n409 = Greater Or Equal?(x=w1107, y=100) -> (x >= y?=w1105:bool)
        n410 = Negate(x=w1083) -> (-x=w1082:dbl)
        n411 = call-poly <vilib>:"CTRE_Phoenix_MotorController_Get_Enhanced.vi"("PhoenixMotorControlDevRef"=w1084, "error in"=w1085) -> ("Quadrature Position"=w1103:i32)  [unwired: 10 in, 3 out]
        n412 = To Double Precision Float(number=w1103) -> (double precision float=w1102:dbl)
        n413 = feedback #7() -> (w1086:dbl)  [unwired: 1 in]
        n414 = call-poly <vilib>:"WPI_RobotDriveArcadeDrive.vi"("error in (no error)"=w1089, "Y axis value"=w1086, "X axis value"=w1082, "RobotDriveDevRef"=w1090) -> ()  [unwired: 5 in, 3 out]
        n415 = Absolute Value(x=w1102) -> (abs(x)=w1098:dbl)
        n416 = Greater Or Equal?(x=w1098, y=115000.0 ("upper limit")) -> (x >= y?=w1087:bool)
        n417 = And(x=w1087, y=w1105) -> (x .and. y?=w1104:bool)
        n418 = Select(t=0.0, s=w1087, f=-0.8) -> (s? t:f=w1099:dbl)
        n419 = feedback-in #7(w1099) -> ()
      }
      n420 = while {
        tunnel: w992 -> [w1056]
        tunnel: w991 -> [w1055]
        tunnel: w990 -> [w1054]
        tunnel: w989 -> [w1053]
        tunnel: [w1056] -> w988
        tunnel: [w1055] -> w987
        tunnel: [w1054] -> w986
        tunnel: [w1053] -> w985
        i -> [w1059]
        stop <- w1057 stop-if-true
        n421 = global read "Robot Global Data.vi" "YAW"() -> (w1063:dbl)
        n422 = Increment(x=w1059) -> (x+1=w1061:i32)
        n423 = call-poly <vilib>:"PID.vi"("output range"=cluster{"output high":dbl, "output low":dbl} {"output high"=0.7, "output low"=-0.7}, "PID gains"=T7 {"proportional gain (Kc)"=0.045, "integral time (Ti, min)"=0.0, "derivative time (Td, min)"=0.0}, "process variable"=w1063, "setpoint"=90.0) -> ("output"=w1048:dbl)  [unwired: 6 in, 1 out]
        n424 = call <vilib>:"WPI_RobotDriveRefNum Registry Get.vi"("refnum name"="RobotDrive") -> ("error out"=w1051:errorcluster, "RobotDriveDevRef"=w1052:T15)  [unwired: 9 in]
        n425 = Greater?(x=w1061, y=200) -> (0:w1057:bool)
        n426 = Negate(x=w1048) -> (-x=w1047:dbl)
        n427 = call-poly <vilib>:"WPI_RobotDriveArcadeDrive.vi"("error in (no error)"=w1051, "Y axis value"=0.0, "X axis value"=w1047, "RobotDriveDevRef"=w1052) -> ()  [unwired: 5 in, 3 out]
        n428 = Wait (ms)(milliseconds to wait=u32 20) -> ()  [unwired: 1 out]
      }
      n429 = while {
        tunnel: [w1039] -> w984
        tunnel: w988 -> [w1039]
        tunnel: [w1038] -> w983
        tunnel: w987 -> [w1038]
        tunnel: [w1037] -> w982
        tunnel: w986 -> [w1037]
        tunnel: [w1040] -> w981
        tunnel: w985 -> [w1040]
        i -> [w1033]
        stop <- w1019 stop-if-true
        # "Set config to shoot level, Rev, Shoot"
        n430 = global read "Robot Global Data.vi" "Pot 1"() -> (w1041:dbl)
        n431 = call <vilib>:"WPI_MotorControlRefNum Registry Get.vi"("refnum name"="Acquire") -> ("error out"=w1034:errorcluster, "MotorControlDevRef"=w1035:T8)  [unwired: 9 in]
        n432 = call <vilib>:"WPI_MotorControlRefNum Registry Get.vi"("refnum name"="Dart 1") -> ("error out"=w1045:errorcluster, "MotorControlDevRef"=w1044:T8)  [unwired: 9 in]
        n433 = Increment(x=w1033) -> (x+1=w1020:i32)
        n434 = call-poly <vilib>:"PID.vi"("PID gains"=T7 {"proportional gain (Kc)"=1.0, "integral time (Ti, min)"=0.01, "derivative time (Td, min)"=0.0}, "process variable"=w1041, "setpoint"=0.0) -> ("output"=w1046:dbl)  [unwired: 7 in, 1 out]
        n435 = Greater Or Equal?(x=w1020, y=100) -> (x >= y?=w1025:bool)
        n436 = call <vilib>:"WPI_MotorControlSetOutput.vi"("error in (no error)"=w1045, "Output"=w1046, "MotorControlDevRef"=w1044) -> ()  [unwired: 6 in, 3 out]
        n437 = call <vilib>:"WPI_MotorControlSetOutput.vi"("error in (no error)"=w1034, "Output"=-1.0, "MotorControlDevRef"=w1035) -> ()  [unwired: 6 in, 3 out]
        n438 = Select(t=WPI_SolenoidValue."Forward" ("Value"), s=w1025, f=WPI_SolenoidValue."Off" ("Value")) -> (s? t:f=w1028:T6)
        n439 = Wait (ms)(milliseconds to wait=u32 20) -> ()  [unwired: 1 out]
        n440 = call <vilib>:"WPI_SolenoidRefNum Registry Get.vi"("refnum name"="Push") -> ("error out"=w1029:errorcluster, "SolenoidDevRef"=w1030:T16)  [unwired: 9 in]
        n441 = call-poly <vilib>:"WPI_SolenoidSet.vi"("error in (no error)"=w1029, "Value"=w1028, "SolenoidDevRef"=w1030) -> ("error out"=w1021:errorcluster, "SolenoidDevRef"=w1022:T16)  [unwired: 7 in]
        n442 = call-poly <vilib>:"WPI_SolenoidGet.vi"("error in (no error)"=w1021, "SolenoidDevRef"=w1022) -> ("Value"=w1019:bool)  [unwired: 7 in, 2 out]
      }
      n443 = while {
        tunnel: w984 -> [w1011]
        tunnel: w983 -> [w1010]
        tunnel: w982 -> [w1009]
        tunnel: w981 -> [w1008]
        tunnel: [w1011] -> _
        tunnel: [w1010] -> _
        tunnel: [w1009] -> _
        tunnel: [w1008] -> _
        i -> [w999]
        stop <- w998 stop-if-true
        # "Reset"
        n444 = call <vilib>:"WPI_SolenoidRefNum Registry Get.vi"("refnum name"="Push") -> ("error out"=w1015:errorcluster, "SolenoidDevRef"=w1016:T16)  [unwired: 9 in]
        n445 = call <vilib>:"WPI_MotorControlRefNum Registry Get.vi"("refnum name"="Dart 1") -> ("error out"=w1006:errorcluster, "MotorControlDevRef"=w1005:T8)  [unwired: 9 in]
        n446 = Increment(x=w999) -> (x+1=w1012:i32)
        n447 = global read "Robot Global Data.vi" "Pot 1"() -> (w1002:dbl)
        n448 = Greater Or Equal?(x=w1012, y=100) -> (x >= y?=w998:bool)
        n449 = call-poly <vilib>:"PID.vi"("PID gains"=T7 {"proportional gain (Kc)"=1.0, "integral time (Ti, min)"=0.01, "derivative time (Td, min)"=0.0}, "process variable"=w1002, "setpoint"=0.0) -> ("output"=w1007:dbl)  [unwired: 7 in, 1 out]
        n450 = call <vilib>:"WPI_MotorControlSetOutput.vi"("error in (no error)"=w1006, "Output"=w1007, "MotorControlDevRef"=w1005) -> ()  [unwired: 6 in, 3 out]
        n451 = call-poly <vilib>:"WPI_SolenoidSet.vi"("error in (no error)"=w1015, "Value"=WPI_SolenoidValue."Reverse", "SolenoidDevRef"=w1016) -> ("error out"=w1013:errorcluster, "SolenoidDevRef"=w1014:T16)  [unwired: 7 in]
        n452 = call-poly <vilib>:"WPI_SolenoidGet.vi"("error in (no error)"=w1013, "SolenoidDevRef"=w1014) -> ()  [unwired: 7 in, 3 out]
      }
    }
    frame "Place Switch and Scale Right" {
      # "DONE"
      n453 = call <vilib>:"WPI_MotorControlRefNum Registry Get.vi"("refnum name"="Left Lead") -> ("error out"=w1146:errorcluster, "MotorControlDevRef"=w1147:T8)  [unwired: 9 in]
      n454 = call <vilib>:"WPI_MotorControlRefNum Registry Get.vi"("refnum name"="Right Lead") -> ("error out"=w1144:errorcluster, "MotorControlDevRef"=w1145:T8)  [unwired: 9 in]
      n455 = while {
        tunnel: w1147 -> [w1375]
        tunnel: w1146 -> [w1374]
        tunnel: w1145 -> [w1373]
        tunnel: w1144 -> [w1372]
        tunnel: [w1375] -> w1155
        tunnel: [w1374] -> w1154
        tunnel: [w1373] -> w1153
        tunnel: [w1372] -> w1152
        i -> [w1385]
        stop <- w1384 stop-if-true
        n456 = Increment(x=w1385) -> (x+1=w1387:i32)
        n457 = Greater?(x=w1387, y=10) -> (0:w1384:bool)
        n458 = call <vilib>:"CTRE_PigeonIMU_RefNumRegistryGet.vi"("refnum name"="Pigeon") -> ("PigeonIMUDevRef"=w1382:T13)  [unwired: 9 in, 1 out]
        n459 = call-poly <vilib>:"CTRE_Phoenix_MotorController_Get_Enhanced.vi"("PhoenixMotorControlDevRef"=w1375, "error in"=w1374) -> ("PhoenixMotorControlDevRef"=w1377:T8)  [unwired: 10 in, 3 out]
        n460 = call-poly <vilib>:"CTRE_Phoenix_MotorController_Get_Enhanced.vi"("PhoenixMotorControlDevRef"=w1373, "error in"=w1372) -> ("PhoenixMotorControlDevRef"=w1376:T8)  [unwired: 10 in, 3 out]
        n461 = call "CTRE_Phoenix_MotorControl_SetQuadraturePosition_Enhanced.vi"("New Position"=0, "PhoenixMotorControlDevRef"=w1376) -> ()  [unwired: 8 in, 2 out]
        n462 = call "CTRE_Phoenix_MotorControl_SetQuadraturePosition_Enhanced.vi"("New Position"=0, "PhoenixMotorControlDevRef"=w1377) -> ()  [unwired: 8 in, 2 out]
        n463 = Wait (ms)(milliseconds to wait=u32 20) -> ()  [unwired: 1 out]
        n464 = call <vilib>:"CTRE_PigeonIMU_SetYaw.vi"("Value"=0.0, "PigeonIMUDevRef"=w1382) -> ()  [unwired: 8 in, 2 out]
      }
      n465 = while {
        tunnel: [w1390] -> w1151
        tunnel: w1155 -> [w1390]
        tunnel: [w1391] -> w1150
        tunnel: w1154 -> [w1391]
        tunnel: [w1398] -> w1149
        tunnel: w1153 -> [w1398]
        tunnel: [w1397] -> w1148
        tunnel: w1152 -> [w1397]
        i -> [w1414]
        stop <- w1410 stop-if-true
        n466 = global read "Robot Global Data.vi" "YAW"() -> (w1399:dbl)
        n467 = Wait (ms)(milliseconds to wait=u32 20) -> ()  [unwired: 1 out]
        n468 = call <vilib>:"WPI_RobotDriveRefNum Registry Get.vi"("refnum name"="RobotDrive") -> ("error out"=w1395:errorcluster, "RobotDriveDevRef"=w1396:T15)  [unwired: 9 in]
        n469 = Increment(x=w1414) -> (x+1=w1413:i32)
        n470 = call-poly <vilib>:"PID.vi"("output range"=cluster{"output high":dbl, "output low":dbl} {"output high"=0.4, "output low"=-0.4}, "PID gains"=T7 {"proportional gain (Kc)"=0.11, "integral time (Ti, min)"=0.0, "derivative time (Td, min)"=0.0}, "process variable"=w1399, "setpoint"=0.0) -> ("output"=w1389:dbl)  [unwired: 6 in, 1 out]
        n471 = Greater Or Equal?(x=w1413, y=100) -> (x >= y?=w1411:bool)
        n472 = Negate(x=w1389) -> (-x=w1388:dbl)
        n473 = call-poly <vilib>:"CTRE_Phoenix_MotorController_Get_Enhanced.vi"("PhoenixMotorControlDevRef"=w1390, "error in"=w1391) -> ("Quadrature Position"=w1409:i32)  [unwired: 10 in, 3 out]
        n474 = To Double Precision Float(number=w1409) -> (double precision float=w1408:dbl)
        n475 = feedback #8() -> (w1392:dbl)  [unwired: 1 in]
        n476 = call-poly <vilib>:"WPI_RobotDriveArcadeDrive.vi"("error in (no error)"=w1395, "Y axis value"=w1392, "X axis value"=w1388, "RobotDriveDevRef"=w1396) -> ()  [unwired: 5 in, 3 out]
        n477 = Absolute Value(x=w1408) -> (abs(x)=w1404:dbl)
        n478 = Greater Or Equal?(x=w1404, y=115000.0 ("upper limit")) -> (x >= y?=w1393:bool)
        n479 = And(x=w1393, y=w1411) -> (x .and. y?=w1410:bool)
        n480 = Select(t=0.0, s=w1393, f=-0.8) -> (s? t:f=w1405:dbl)
        n481 = feedback-in #8(w1405) -> ()
      }
      n482 = while {
        tunnel: w1151 -> [w1362]
        tunnel: w1150 -> [w1361]
        tunnel: w1149 -> [w1360]
        tunnel: w1148 -> [w1359]
        tunnel: [w1362] -> w1133
        tunnel: [w1361] -> w1132
        tunnel: [w1360] -> w1131
        tunnel: [w1359] -> w1130
        i -> [w1365]
        stop <- w1363 stop-if-true
        n483 = global read "Robot Global Data.vi" "YAW"() -> (w1369:dbl)
        n484 = Increment(x=w1365) -> (x+1=w1367:i32)
        n485 = call-poly <vilib>:"PID.vi"("output range"=cluster{"output high":dbl, "output low":dbl} {"output high"=0.7, "output low"=-0.7}, "PID gains"=T7 {"proportional gain (Kc)"=0.045, "integral time (Ti, min)"=0.0, "derivative time (Td, min)"=0.0}, "process variable"=w1369, "setpoint"=90.0) -> ("output"=w1354:dbl)  [unwired: 6 in, 1 out]
        n486 = call <vilib>:"WPI_RobotDriveRefNum Registry Get.vi"("refnum name"="RobotDrive") -> ("error out"=w1357:errorcluster, "RobotDriveDevRef"=w1358:T15)  [unwired: 9 in]
        n487 = Greater?(x=w1367, y=200) -> (0:w1363:bool)
        n488 = Negate(x=w1354) -> (-x=w1353:dbl)
        n489 = call-poly <vilib>:"WPI_RobotDriveArcadeDrive.vi"("error in (no error)"=w1357, "Y axis value"=25.0, "X axis value"=w1353, "RobotDriveDevRef"=w1358) -> ()  [unwired: 5 in, 3 out]
        n490 = Wait (ms)(milliseconds to wait=u32 20) -> ()  [unwired: 1 out]
      }
      n491 = while {
        tunnel: [w1198] -> w1137
        tunnel: w1133 -> [w1198]
        tunnel: [w1197] -> w1136
        tunnel: w1132 -> [w1197]
        tunnel: [w1196] -> w1135
        tunnel: w1131 -> [w1196]
        tunnel: [w1199] -> w1134
        tunnel: w1130 -> [w1199]
        i -> [w1192]
        stop <- w1178 stop-if-true
        # "Set config to shoot level, Rev, Shoot"
        n492 = global read "Robot Global Data.vi" "Pot 1"() -> (w1200:dbl)
        n493 = call <vilib>:"WPI_MotorControlRefNum Registry Get.vi"("refnum name"="Acquire") -> ("error out"=w1193:errorcluster, "MotorControlDevRef"=w1194:T8)  [unwired: 9 in]
        n494 = call <vilib>:"WPI_MotorControlRefNum Registry Get.vi"("refnum name"="Dart 1") -> ("error out"=w1204:errorcluster, "MotorControlDevRef"=w1203:T8)  [unwired: 9 in]
        n495 = Increment(x=w1192) -> (x+1=w1179:i32)
        n496 = call-poly <vilib>:"PID.vi"("PID gains"=T7 {"proportional gain (Kc)"=1.0, "integral time (Ti, min)"=0.01, "derivative time (Td, min)"=0.0}, "process variable"=w1200, "setpoint"=0.0) -> ("output"=w1205:dbl)  [unwired: 7 in, 1 out]
        n497 = Greater Or Equal?(x=w1179, y=100) -> (x >= y?=w1184:bool)
        n498 = call <vilib>:"WPI_MotorControlSetOutput.vi"("error in (no error)"=w1204, "Output"=w1205, "MotorControlDevRef"=w1203) -> ()  [unwired: 6 in, 3 out]
        n499 = call <vilib>:"WPI_MotorControlSetOutput.vi"("error in (no error)"=w1193, "Output"=-1.0, "MotorControlDevRef"=w1194) -> ()  [unwired: 6 in, 3 out]
        n500 = Select(t=WPI_SolenoidValue."Forward" ("Value"), s=w1184, f=WPI_SolenoidValue."Off" ("Value")) -> (s? t:f=w1187:T6)
        n501 = Wait (ms)(milliseconds to wait=u32 20) -> ()  [unwired: 1 out]
        n502 = call <vilib>:"WPI_SolenoidRefNum Registry Get.vi"("refnum name"="Push") -> ("error out"=w1188:errorcluster, "SolenoidDevRef"=w1189:T16)  [unwired: 9 in]
        n503 = call-poly <vilib>:"WPI_SolenoidSet.vi"("error in (no error)"=w1188, "Value"=w1187, "SolenoidDevRef"=w1189) -> ("error out"=w1180:errorcluster, "SolenoidDevRef"=w1181:T16)  [unwired: 7 in]
        n504 = call-poly <vilib>:"WPI_SolenoidGet.vi"("error in (no error)"=w1180, "SolenoidDevRef"=w1181) -> ("Value"=w1178:bool)  [unwired: 7 in, 2 out]
      }
      n505 = while {
        tunnel: w1137 -> [w1170]
        tunnel: w1136 -> [w1169]
        tunnel: w1135 -> [w1168]
        tunnel: w1134 -> [w1167]
        tunnel: [w1170] -> w1129
        tunnel: [w1169] -> w1128
        tunnel: [w1168] -> w1127
        tunnel: [w1167] -> w1126
        i -> [w1158]
        stop <- w1157 stop-if-true
        # "Reset"
        n506 = call <vilib>:"WPI_SolenoidRefNum Registry Get.vi"("refnum name"="Push") -> ("error out"=w1174:errorcluster, "SolenoidDevRef"=w1175:T16)  [unwired: 9 in]
        n507 = call <vilib>:"WPI_MotorControlRefNum Registry Get.vi"("refnum name"="Dart 1") -> ("error out"=w1165:errorcluster, "MotorControlDevRef"=w1164:T8)  [unwired: 9 in]
        n508 = Increment(x=w1158) -> (x+1=w1171:i32)
        n509 = global read "Robot Global Data.vi" "Pot 1"() -> (w1161:dbl)
        n510 = call-poly <vilib>:"PID.vi"("PID gains"=T7 {"proportional gain (Kc)"=1.0, "integral time (Ti, min)"=0.01, "derivative time (Td, min)"=0.0}, "process variable"=w1161, "setpoint"=0.0) -> ("output"=w1166:dbl)  [unwired: 7 in, 1 out]
        n511 = call <vilib>:"WPI_MotorControlSetOutput.vi"("error in (no error)"=w1165, "Output"=w1166, "MotorControlDevRef"=w1164) -> ()  [unwired: 6 in, 3 out]
        n512 = call-poly <vilib>:"WPI_SolenoidSet.vi"("error in (no error)"=w1174, "Value"=WPI_SolenoidValue."Reverse", "SolenoidDevRef"=w1175) -> ("error out"=w1172:errorcluster, "SolenoidDevRef"=w1173:T16)  [unwired: 7 in]
        n513 = Greater Or Equal?(x=w1171, y=100) -> (x >= y?=w1157:bool)
        n514 = call-poly <vilib>:"WPI_SolenoidGet.vi"("error in (no error)"=w1172, "SolenoidDevRef"=w1173) -> ()  [unwired: 7 in, 3 out]
      }
      n515 = while {
        tunnel: w1129 -> [w1293]
        tunnel: w1128 -> [w1292]
        tunnel: w1127 -> [w1291]
        tunnel: w1126 -> [w1290]
        tunnel: [w1293] -> w1117
        tunnel: [w1292] -> w1114
        tunnel: [w1291] -> w1116
        tunnel: [w1290] -> w1115
        i -> [w1296]
        stop <- w1294 stop-if-true
        # "change deg"
        n516 = global read "Robot Global Data.vi" "YAW"() -> (w1300:dbl)
        n517 = Increment(x=w1296) -> (x+1=w1298:i32)
        n518 = call-poly <vilib>:"PID.vi"("output range"=cluster{"output high":dbl, "output low":dbl} {"output high"=0.7, "output low"=-0.7}, "PID gains"=T7 {"proportional gain (Kc)"=0.045, "integral time (Ti, min)"=0.0, "derivative time (Td, min)"=0.0}, "process variable"=w1300, "setpoint"=-25.0) -> ("output"=w1285:dbl)  [unwired: 6 in, 1 out]
        n519 = call <vilib>:"WPI_RobotDriveRefNum Registry Get.vi"("refnum name"="RobotDrive") -> ("error out"=w1288:errorcluster, "RobotDriveDevRef"=w1289:T15)  [unwired: 9 in]
        n520 = Greater?(x=w1298, y=200) -> (0:w1294:bool)
        n521 = Negate(x=w1285) -> (-x=w1284:dbl)
        n522 = call-poly <vilib>:"WPI_RobotDriveArcadeDrive.vi"("error in (no error)"=w1288, "Y axis value"=25.0, "X axis value"=w1284, "RobotDriveDevRef"=w1289) -> ()  [unwired: 5 in, 3 out]
        n523 = Wait (ms)(milliseconds to wait=u32 20) -> ()  [unwired: 1 out]
      }
      n524 = while {
        tunnel: [w1257] -> w1125
        tunnel: w1117 -> [w1257]
        tunnel: [w1253] -> w1124
        tunnel: [w1256] -> w1123
        tunnel: w1116 -> [w1256]
        tunnel: [w1255] -> w1122
        tunnel: w1115 -> [w1255]
        tunnel: w1114 -> [w1253]
        i -> [w1282]
        stop <- w1278 stop-if-true
        # "Drives towards cube, uses pixy cam's \"x\" value to stay on center"
        n525 = Increment(x=w1282) -> (x+1=w1281:i32)
        n526 = Greater Or Equal?(x=w1281, y=100) -> (x >= y?=w1279:bool)
        n527 = call <vilib>:"WPI_DigitalInputRefNum Registry Get.vi"("refnum name"="Color Mark") -> ("DigitalInputDevRef"=w1268:T18)  [unwired: 9 in, 1 out]
        n528 = call <vilib>:"WPI_MotorControlRefNum Registry Get.vi"("refnum name"="Acquire") -> ("error out"=w1265:errorcluster, "MotorControlDevRef"=w1266:T8)  [unwired: 9 in]
        n529 = call <vilib>:"WPI_DigitalInputGetValue.vi"("DigitalInputDevRef"=w1268) -> ("Value"=w1258:bool)  [unwired: 8 in, 2 out]
        n530 = And(x=w1258, y=w1279) -> (x .and. y?=w1278:bool)
        n531 = Wait (ms)(milliseconds to wait=u32 20) -> ()  [unwired: 1 out]
        n532 = Select(t=0.0, s=w1258, f=0.6) -> (s? t:f=w1259:dbl)
        n533 = Select(t=0.0, s=w1258, f=0.6) -> (s? t:f=w1262:dbl)
        n534 = call <vilib>:"WPI_MotorControlSetOutput.vi"("error in (no error)"=w1265, "Output"=w1259, "MotorControlDevRef"=w1266) -> ()  [unwired: 6 in, 3 out]
        n535 = call "PIXY VI.vi"() -> ("X"=w1269:dbl)  [unwired: 14 in, 5 out]
        n536 = call <vilib>:"WPI_RobotDriveRefNum Registry Get.vi"("refnum name"="RobotDrive") -> ("error out"=w1274:errorcluster, "RobotDriveDevRef"=w1275:T15)  [unwired: 9 in]
        n537 = call-poly <vilib>:"PID.vi"("output range"=cluster{"output high":dbl, "output low":dbl} {"output high"=0.4, "output low"=-0.4}, "PID gains"=T7 {"proportional gain (Kc)"=0.11, "integral time (Ti, min)"=0.0, "derivative time (Td, min)"=0.0}, "process variable"=w1269, "setpoint"=0.0) -> ("output"=w1272:dbl)  [unwired: 6 in, 1 out]
        n538 = Negate(x=w1272) -> (-x=w1271:dbl)
        n539 = call-poly <vilib>:"WPI_RobotDriveArcadeDrive.vi"("error in (no error)"=w1274, "Y axis value"=w1262, "X axis value"=w1271, "RobotDriveDevRef"=w1275) -> ()  [unwired: 5 in, 3 out]
      }
      n540 = while {
        tunnel: [w1227] -> w1110
        tunnel: w1125 -> [w1227]
        tunnel: [w1228] -> w1111
        tunnel: w1124 -> [w1228]
        tunnel: [w1235] -> w1112
        tunnel: w1123 -> [w1235]
        tunnel: [w1234] -> w1113
        tunnel: w1122 -> [w1234]
        i -> [w1251]
        stop <- w1247 stop-if-true
        n541 = global read "Robot Global Data.vi" "YAW"() -> (w1236:dbl)
        n542 = Wait (ms)(milliseconds to wait=u32 20) -> ()  [unwired: 1 out]
        n543 = call <vilib>:"WPI_RobotDriveRefNum Registry Get.vi"("refnum name"="RobotDrive") -> ("error out"=w1232:errorcluster, "RobotDriveDevRef"=w1233:T15)  [unwired: 9 in]
        n544 = Increment(x=w1251) -> (x+1=w1250:i32)
        n545 = call-poly <vilib>:"PID.vi"("output range"=cluster{"output high":dbl, "output low":dbl} {"output high"=0.4, "output low"=-0.4}, "PID gains"=T7 {"proportional gain (Kc)"=0.11, "integral time (Ti, min)"=0.0, "derivative time (Td, min)"=0.0}, "process variable"=w1236, "setpoint"=0.0) -> ("output"=w1226:dbl)  [unwired: 6 in, 1 out]
        n546 = Greater Or Equal?(x=w1250, y=100) -> (x >= y?=w1248:bool)
        n547 = Negate(x=w1226) -> (-x=w1225:dbl)
        n548 = call-poly <vilib>:"CTRE_Phoenix_MotorController_Get_Enhanced.vi"("PhoenixMotorControlDevRef"=w1227, "error in"=w1228) -> ("Quadrature Position"=w1246:i32)  [unwired: 10 in, 3 out]
        n549 = To Double Precision Float(number=w1246) -> (double precision float=w1245:dbl)
        n550 = feedback #9() -> (w1229:dbl)  [unwired: 1 in]
        n551 = call-poly <vilib>:"WPI_RobotDriveArcadeDrive.vi"("error in (no error)"=w1232, "Y axis value"=w1229, "X axis value"=w1225, "RobotDriveDevRef"=w1233) -> ()  [unwired: 5 in, 3 out]
        n552 = Absolute Value(x=w1245) -> (abs(x)=w1241:dbl)
        n553 = Greater Or Equal?(x=w1241, y=115000.0 ("upper limit")) -> (x >= y?=w1230:bool)
        n554 = And(x=w1230, y=w1248) -> (x .and. y?=w1247:bool)
        n555 = Select(t=0.0, s=w1230, f=-0.8) -> (s? t:f=w1242:dbl)
        n556 = feedback-in #9(w1242) -> ()
      }
      n557 = while {
        tunnel: w1110 -> [w1215]
        tunnel: w1111 -> [w1214]
        tunnel: w1112 -> [w1213]
        tunnel: w1113 -> [w1212]
        tunnel: [w1215] -> w1121
        tunnel: [w1214] -> w1120
        tunnel: [w1213] -> w1119
        tunnel: [w1212] -> w1118
        i -> [w1218]
        stop <- w1216 stop-if-true
        n558 = global read "Robot Global Data.vi" "YAW"() -> (w1222:dbl)
        n559 = Increment(x=w1218) -> (x+1=w1220:i32)
        n560 = call-poly <vilib>:"PID.vi"("output range"=cluster{"output high":dbl, "output low":dbl} {"output high"=0.7, "output low"=-0.7}, "PID gains"=T7 {"proportional gain (Kc)"=0.045, "integral time (Ti, min)"=0.0, "derivative time (Td, min)"=0.0}, "process variable"=w1222, "setpoint"=90.0) -> ("output"=w1207:dbl)  [unwired: 6 in, 1 out]
        n561 = call <vilib>:"WPI_RobotDriveRefNum Registry Get.vi"("refnum name"="RobotDrive") -> ("error out"=w1210:errorcluster, "RobotDriveDevRef"=w1211:T15)  [unwired: 9 in]
        n562 = Greater?(x=w1220, y=200) -> (0:w1216:bool)
        n563 = Negate(x=w1207) -> (-x=w1206:dbl)
        n564 = call-poly <vilib>:"WPI_RobotDriveArcadeDrive.vi"("error in (no error)"=w1210, "Y axis value"=25.0, "X axis value"=w1206, "RobotDriveDevRef"=w1211) -> ()  [unwired: 5 in, 3 out]
        n565 = Wait (ms)(milliseconds to wait=u32 20) -> ()  [unwired: 1 out]
      }
      n566 = while {
        tunnel: [w1345] -> w1141
        tunnel: w1121 -> [w1345]
        tunnel: [w1344] -> w1140
        tunnel: w1120 -> [w1344]
        tunnel: [w1343] -> w1139
        tunnel: w1119 -> [w1343]
        tunnel: [w1346] -> w1138
        tunnel: w1118 -> [w1346]
        i -> [w1339]
        stop <- w1325 stop-if-true
        # "Set config to shoot level, Rev, Shoot"
        n567 = global read "Robot Global Data.vi" "Pot 1"() -> (w1347:dbl)
        n568 = call <vilib>:"WPI_MotorControlRefNum Registry Get.vi"("refnum name"="Acquire") -> ("error out"=w1340:errorcluster, "MotorControlDevRef"=w1341:T8)  [unwired: 9 in]
        n569 = call <vilib>:"WPI_MotorControlRefNum Registry Get.vi"("refnum name"="Dart 1") -> ("error out"=w1351:errorcluster, "MotorControlDevRef"=w1350:T8)  [unwired: 9 in]
        n570 = Increment(x=w1339) -> (x+1=w1326:i32)
        n571 = call-poly <vilib>:"PID.vi"("PID gains"=T7 {"proportional gain (Kc)"=1.0, "integral time (Ti, min)"=0.01, "derivative time (Td, min)"=0.0}, "process variable"=w1347, "setpoint"=0.0) -> ("output"=w1352:dbl)  [unwired: 7 in, 1 out]
        n572 = Greater Or Equal?(x=w1326, y=100) -> (x >= y?=w1331:bool)
        n573 = call <vilib>:"WPI_MotorControlSetOutput.vi"("error in (no error)"=w1351, "Output"=w1352, "MotorControlDevRef"=w1350) -> ()  [unwired: 6 in, 3 out]
        n574 = call <vilib>:"WPI_MotorControlSetOutput.vi"("error in (no error)"=w1340, "Output"=-1.0, "MotorControlDevRef"=w1341) -> ()  [unwired: 6 in, 3 out]
        n575 = Select(t=WPI_SolenoidValue."Forward" ("Value"), s=w1331, f=WPI_SolenoidValue."Off" ("Value")) -> (s? t:f=w1334:T6)
        n576 = Wait (ms)(milliseconds to wait=u32 20) -> ()  [unwired: 1 out]
        n577 = call <vilib>:"WPI_SolenoidRefNum Registry Get.vi"("refnum name"="Push") -> ("error out"=w1335:errorcluster, "SolenoidDevRef"=w1336:T16)  [unwired: 9 in]
        n578 = call-poly <vilib>:"WPI_SolenoidSet.vi"("error in (no error)"=w1335, "Value"=w1334, "SolenoidDevRef"=w1336) -> ("error out"=w1327:errorcluster, "SolenoidDevRef"=w1328:T16)  [unwired: 7 in]
        n579 = call-poly <vilib>:"WPI_SolenoidGet.vi"("error in (no error)"=w1327, "SolenoidDevRef"=w1328) -> ("Value"=w1325:bool)  [unwired: 7 in, 2 out]
      }
      n580 = while {
        tunnel: w1141 -> [w1317]
        tunnel: w1140 -> [w1316]
        tunnel: w1139 -> [w1315]
        tunnel: w1138 -> [w1314]
        tunnel: [w1317] -> _
        tunnel: [w1316] -> _
        tunnel: [w1315] -> _
        tunnel: [w1314] -> _
        i -> [w1305]
        stop <- w1304 stop-if-true
        # "Reset"
        n581 = call <vilib>:"WPI_SolenoidRefNum Registry Get.vi"("refnum name"="Push") -> ("error out"=w1321:errorcluster, "SolenoidDevRef"=w1322:T16)  [unwired: 9 in]
        n582 = call <vilib>:"WPI_MotorControlRefNum Registry Get.vi"("refnum name"="Dart 1") -> ("error out"=w1312:errorcluster, "MotorControlDevRef"=w1311:T8)  [unwired: 9 in]
        n583 = Increment(x=w1305) -> (x+1=w1318:i32)
        n584 = global read "Robot Global Data.vi" "Pot 1"() -> (w1308:dbl)
        n585 = Greater Or Equal?(x=w1318, y=100) -> (x >= y?=w1304:bool)
        n586 = call-poly <vilib>:"PID.vi"("PID gains"=T7 {"proportional gain (Kc)"=1.0, "integral time (Ti, min)"=0.01, "derivative time (Td, min)"=0.0}, "process variable"=w1308, "setpoint"=0.0) -> ("output"=w1313:dbl)  [unwired: 7 in, 1 out]
        n587 = call <vilib>:"WPI_MotorControlSetOutput.vi"("error in (no error)"=w1312, "Output"=w1313, "MotorControlDevRef"=w1311) -> ()  [unwired: 6 in, 3 out]
        n588 = call-poly <vilib>:"WPI_SolenoidSet.vi"("error in (no error)"=w1321, "Value"=WPI_SolenoidValue."Reverse", "SolenoidDevRef"=w1322) -> ("error out"=w1319:errorcluster, "SolenoidDevRef"=w1320:T16)  [unwired: 7 in]
        n589 = call-poly <vilib>:"WPI_SolenoidGet.vi"("error in (no error)"=w1319, "SolenoidDevRef"=w1320) -> ()  [unwired: 7 in, 3 out]
      }
    }
    frame "Place 2 Switch Right" {
      # "done"
      n590 = call <vilib>:"WPI_MotorControlRefNum Registry Get.vi"("refnum name"="Left Lead") -> ("error out"=w1420:errorcluster, "MotorControlDevRef"=w1421:T8)  [unwired: 9 in]
      n591 = call <vilib>:"WPI_MotorControlRefNum Registry Get.vi"("refnum name"="Right Lead") -> ("error out"=w1418:errorcluster, "MotorControlDevRef"=w1419:T8)  [unwired: 9 in]
      n592 = while {
        tunnel: w1421 -> [w1703]
        tunnel: w1420 -> [w1702]
        tunnel: w1419 -> [w1701]
        tunnel: w1418 -> [w1700]
        tunnel: [w1703] -> w1461
        tunnel: [w1702] -> w1460
        tunnel: [w1701] -> w1459
        tunnel: [w1700] -> w1458
        i -> [w1713]
        stop <- w1712 stop-if-true
        n593 = Increment(x=w1713) -> (x+1=w1715:i32)
        n594 = Greater?(x=w1715, y=10) -> (0:w1712:bool)
        n595 = call <vilib>:"CTRE_PigeonIMU_RefNumRegistryGet.vi"("refnum name"="Pigeon") -> ("PigeonIMUDevRef"=w1710:T13)  [unwired: 9 in, 1 out]
        n596 = call-poly <vilib>:"CTRE_Phoenix_MotorController_Get_Enhanced.vi"("PhoenixMotorControlDevRef"=w1703, "error in"=w1702) -> ("PhoenixMotorControlDevRef"=w1705:T8)  [unwired: 10 in, 3 out]
        n597 = call-poly <vilib>:"CTRE_Phoenix_MotorController_Get_Enhanced.vi"("PhoenixMotorControlDevRef"=w1701, "error in"=w1700) -> ("PhoenixMotorControlDevRef"=w1704:T8)  [unwired: 10 in, 3 out]
        n598 = call "CTRE_Phoenix_MotorControl_SetQuadraturePosition_Enhanced.vi"("New Position"=0, "PhoenixMotorControlDevRef"=w1704) -> ()  [unwired: 8 in, 2 out]
        n599 = call "CTRE_Phoenix_MotorControl_SetQuadraturePosition_Enhanced.vi"("New Position"=0, "PhoenixMotorControlDevRef"=w1705) -> ()  [unwired: 8 in, 2 out]
        n600 = Wait (ms)(milliseconds to wait=u32 20) -> ()  [unwired: 1 out]
        n601 = call <vilib>:"CTRE_PigeonIMU_SetYaw.vi"("Value"=0.0, "PigeonIMUDevRef"=w1710) -> ()  [unwired: 8 in, 2 out]
      }
      n602 = while {
        tunnel: [w1718] -> w1457
        tunnel: w1461 -> [w1718]
        tunnel: [w1719] -> w1456
        tunnel: w1460 -> [w1719]
        tunnel: [w1726] -> w1455
        tunnel: w1459 -> [w1726]
        tunnel: [w1725] -> w1454
        tunnel: w1458 -> [w1725]
        i -> [w1742]
        stop <- w1738 stop-if-true
        n603 = global read "Robot Global Data.vi" "YAW"() -> (w1727:dbl)
        n604 = Wait (ms)(milliseconds to wait=u32 20) -> ()  [unwired: 1 out]
        n605 = call <vilib>:"WPI_RobotDriveRefNum Registry Get.vi"("refnum name"="RobotDrive") -> ("error out"=w1723:errorcluster, "RobotDriveDevRef"=w1724:T15)  [unwired: 9 in]
        n606 = Increment(x=w1742) -> (x+1=w1741:i32)
        n607 = call-poly <vilib>:"PID.vi"("output range"=cluster{"output high":dbl, "output low":dbl} {"output high"=0.4, "output low"=-0.4}, "PID gains"=T7 {"proportional gain (Kc)"=0.11, "integral time (Ti, min)"=0.0, "derivative time (Td, min)"=0.0}, "process variable"=w1727, "setpoint"=0.0) -> ("output"=w1717:dbl)  [unwired: 6 in, 1 out]
        n608 = Greater Or Equal?(x=w1741, y=100) -> (x >= y?=w1739:bool)
        n609 = Negate(x=w1717) -> (-x=w1716:dbl)
        n610 = call-poly <vilib>:"CTRE_Phoenix_MotorController_Get_Enhanced.vi"("PhoenixMotorControlDevRef"=w1718, "error in"=w1719) -> ("Quadrature Position"=w1737:i32)  [unwired: 10 in, 3 out]
        n611 = To Double Precision Float(number=w1737) -> (double precision float=w1736:dbl)
        n612 = feedback #10() -> (w1720:dbl)  [unwired: 1 in]
        n613 = call-poly <vilib>:"WPI_RobotDriveArcadeDrive.vi"("error in (no error)"=w1723, "Y axis value"=w1720, "X axis value"=w1716, "RobotDriveDevRef"=w1724) -> ()  [unwired: 5 in, 3 out]
        n614 = Absolute Value(x=w1736) -> (abs(x)=w1732:dbl)
        n615 = Greater Or Equal?(x=w1732, y=115000.0 ("upper limit")) -> (x >= y?=w1721:bool)
        n616 = And(x=w1721, y=w1739) -> (x .and. y?=w1738:bool)
        n617 = Select(t=0.0, s=w1721, f=-0.8) -> (s? t:f=w1733:dbl)
        n618 = feedback-in #10(w1733) -> ()
      }
      n619 = while {
        tunnel: w1457 -> [w1690]
        tunnel: w1456 -> [w1689]
        tunnel: w1455 -> [w1688]
        tunnel: w1454 -> [w1687]
        tunnel: [w1690] -> w1453
        tunnel: [w1689] -> w1452
        tunnel: [w1688] -> w1451
        tunnel: [w1687] -> w1450
        i -> [w1693]
        stop <- w1691 stop-if-true
        n620 = global read "Robot Global Data.vi" "YAW"() -> (w1697:dbl)
        n621 = Increment(x=w1693) -> (x+1=w1695:i32)
        n622 = call-poly <vilib>:"PID.vi"("output range"=cluster{"output high":dbl, "output low":dbl} {"output high"=0.7, "output low"=-0.7}, "PID gains"=T7 {"proportional gain (Kc)"=0.045, "integral time (Ti, min)"=0.0, "derivative time (Td, min)"=0.0}, "process variable"=w1697, "setpoint"=-90.0) -> ("output"=w1682:dbl)  [unwired: 6 in, 1 out]
        n623 = call <vilib>:"WPI_RobotDriveRefNum Registry Get.vi"("refnum name"="RobotDrive") -> ("error out"=w1685:errorcluster, "RobotDriveDevRef"=w1686:T15)  [unwired: 9 in]
        n624 = Greater?(x=w1695, y=200) -> (0:w1691:bool)
        n625 = Negate(x=w1682) -> (-x=w1681:dbl)
        n626 = call-poly <vilib>:"WPI_RobotDriveArcadeDrive.vi"("error in (no error)"=w1685, "Y axis value"=0.0, "X axis value"=w1681, "RobotDriveDevRef"=w1686) -> ()  [unwired: 5 in, 3 out]
        n627 = Wait (ms)(milliseconds to wait=u32 20) -> ()  [unwired: 1 out]
      }
      n628 = while {
        tunnel: [w1590] -> w1449
        tunnel: w1453 -> [w1590]
        tunnel: [w1589] -> w1448
        tunnel: w1452 -> [w1589]
        tunnel: [w1588] -> w1447
        tunnel: w1451 -> [w1588]
        tunnel: [w1591] -> w1446
        tunnel: w1450 -> [w1591]
        i -> [w1584]
        stop <- w1570 stop-if-true
        # "Set config to shoot level, Rev, Shoot"
        n629 = global read "Robot Global Data.vi" "Pot 1"() -> (w1592:dbl)
        n630 = call <vilib>:"WPI_MotorControlRefNum Registry Get.vi"("refnum name"="Acquire") -> ("error out"=w1585:errorcluster, "MotorControlDevRef"=w1586:T8)  [unwired: 9 in]
        n631 = call <vilib>:"WPI_MotorControlRefNum Registry Get.vi"("refnum name"="Dart 1") -> ("error out"=w1596:errorcluster, "MotorControlDevRef"=w1595:T8)  [unwired: 9 in]
        n632 = Increment(x=w1584) -> (x+1=w1571:i32)
        n633 = call-poly <vilib>:"PID.vi"("PID gains"=T7 {"proportional gain (Kc)"=1.0, "integral time (Ti, min)"=0.01, "derivative time (Td, min)"=0.0}, "process variable"=w1592, "setpoint"=0.0) -> ("output"=w1597:dbl)  [unwired: 7 in, 1 out]
        n634 = Greater Or Equal?(x=w1571, y=100) -> (x >= y?=w1576:bool)
        n635 = call <vilib>:"WPI_MotorControlSetOutput.vi"("error in (no error)"=w1596, "Output"=w1597, "MotorControlDevRef"=w1595) -> ()  [unwired: 6 in, 3 out]
        n636 = call <vilib>:"WPI_MotorControlSetOutput.vi"("error in (no error)"=w1585, "Output"=-1.0, "MotorControlDevRef"=w1586) -> ()  [unwired: 6 in, 3 out]
        n637 = Select(t=WPI_SolenoidValue."Forward" ("Value"), s=w1576, f=WPI_SolenoidValue."Off" ("Value")) -> (s? t:f=w1579:T6)
        n638 = Wait (ms)(milliseconds to wait=u32 20) -> ()  [unwired: 1 out]
        n639 = call <vilib>:"WPI_SolenoidRefNum Registry Get.vi"("refnum name"="Push") -> ("error out"=w1580:errorcluster, "SolenoidDevRef"=w1581:T16)  [unwired: 9 in]
        n640 = call-poly <vilib>:"WPI_SolenoidSet.vi"("error in (no error)"=w1580, "Value"=w1579, "SolenoidDevRef"=w1581) -> ("error out"=w1572:errorcluster, "SolenoidDevRef"=w1573:T16)  [unwired: 7 in]
        n641 = call-poly <vilib>:"WPI_SolenoidGet.vi"("error in (no error)"=w1572, "SolenoidDevRef"=w1573) -> ("Value"=w1570:bool)  [unwired: 7 in, 2 out]
      }
      n642 = while {
        tunnel: w1449 -> [w1476]
        tunnel: w1448 -> [w1475]
        tunnel: w1447 -> [w1474]
        tunnel: w1446 -> [w1473]
        tunnel: [w1476] -> w1445
        tunnel: [w1475] -> w1444
        tunnel: [w1474] -> w1443
        tunnel: [w1473] -> w1442
        i -> [w1464]
        stop <- w1463 stop-if-true
        # "Reset"
        n643 = call <vilib>:"WPI_SolenoidRefNum Registry Get.vi"("refnum name"="Push") -> ("error out"=w1480:errorcluster, "SolenoidDevRef"=w1481:T16)  [unwired: 9 in]
        n644 = call <vilib>:"WPI_MotorControlRefNum Registry Get.vi"("refnum name"="Dart 1") -> ("error out"=w1471:errorcluster, "MotorControlDevRef"=w1470:T8)  [unwired: 9 in]
        n645 = Increment(x=w1464) -> (x+1=w1477:i32)
        n646 = global read "Robot Global Data.vi" "Pot 1"() -> (w1467:dbl)
        n647 = Greater Or Equal?(x=w1477, y=100) -> (x >= y?=w1463:bool)
        n648 = call-poly <vilib>:"PID.vi"("PID gains"=T7 {"proportional gain (Kc)"=1.0, "integral time (Ti, min)"=0.01, "derivative time (Td, min)"=0.0}, "process variable"=w1467, "setpoint"=0.0) -> ("output"=w1472:dbl)  [unwired: 7 in, 1 out]
        n649 = call <vilib>:"WPI_MotorControlSetOutput.vi"("error in (no error)"=w1471, "Output"=w1472, "MotorControlDevRef"=w1470) -> ()  [unwired: 6 in, 3 out]
        n650 = call-poly <vilib>:"WPI_SolenoidSet.vi"("error in (no error)"=w1480, "Value"=WPI_SolenoidValue."Reverse", "SolenoidDevRef"=w1481) -> ("error out"=w1478:errorcluster, "SolenoidDevRef"=w1479:T16)  [unwired: 7 in]
        n651 = call-poly <vilib>:"WPI_SolenoidGet.vi"("error in (no error)"=w1478, "SolenoidDevRef"=w1479) -> ()  [unwired: 7 in, 3 out]
      }
      n652 = while {
        tunnel: [w1661] -> w1441
        tunnel: w1445 -> [w1661]
        tunnel: [w1660] -> w1440
        tunnel: w1444 -> [w1660]
        tunnel: [w1659] -> w1439
        tunnel: w1443 -> [w1659]
        tunnel: [w1658] -> w1438
        tunnel: w1442 -> [w1658]
        i -> [w1674]
        stop <- w1672 stop-if-true
        n653 = global read "Robot Global Data.vi" "YAW"() -> (w1678:dbl)
        n654 = Increment(x=w1674) -> (x+1=w1676:i32)
        n655 = call-poly <vilib>:"PID.vi"("output range"=cluster{"output high":dbl, "output low":dbl} {"output high"=0.6, "output low"=-0.6}, "PID gains"=T7 {"proportional gain (Kc)"=0.055, "integral time (Ti, min)"=0.0, "derivative time (Td, min)"=0.0}, "process variable"=w1678, "setpoint"=-25.0) -> ("output"=w1668:dbl)  [unwired: 6 in, 1 out]
        n656 = call <vilib>:"WPI_RobotDriveRefNum Registry Get.vi"("refnum name"="RobotDrive") -> ("error out"=w1669:errorcluster, "RobotDriveDevRef"=w1670:T15)  [unwired: 9 in]
        n657 = Negate(x=w1668) -> (-x=w1667:dbl)
        n658 = Greater?(x=w1676, y=180) -> (0:w1672:bool)
        n659 = call-poly <vilib>:"WPI_RobotDriveArcadeDrive.vi"("error in (no error)"=w1669, "Y axis value"=0.0, "X axis value"=w1667, "RobotDriveDevRef"=w1670) -> ()  [unwired: 5 in, 3 out]
        n660 = Wait (ms)(milliseconds to wait=u32 20) -> ()  [unwired: 1 out]
        n661 = call-poly <vilib>:"CTRE_Phoenix_MotorController_Get_Enhanced.vi"("PhoenixMotorControlDevRef"=w1661, "error in"=w1660) -> ("PhoenixMotorControlDevRef"=w1663:T8)  [unwired: 8 in, 5 out]
        n662 = call-poly <vilib>:"CTRE_Phoenix_MotorController_Get_Enhanced.vi"("PhoenixMotorControlDevRef"=w1659, "error in"=w1658) -> ("PhoenixMotorControlDevRef"=w1662:T8)  [unwired: 8 in, 5 out]
        n663 = call "CTRE_Phoenix_MotorControl_SetQuadraturePosition_Enhanced.vi"("New Position"=0, "PhoenixMotorControlDevRef"=w1662) -> ()  [unwired: 8 in, 2 out]
        n664 = call "CTRE_Phoenix_MotorControl_SetQuadraturePosition_Enhanced.vi"("New Position"=0, "PhoenixMotorControlDevRef"=w1663) -> ()  [unwired: 8 in, 2 out]
      }
      n665 = while {
        tunnel: [w1631] -> w1437
        tunnel: w1441 -> [w1631]
        tunnel: [w1630] -> w1436
        tunnel: w1440 -> [w1630]
        tunnel: [w1629] -> w1435
        tunnel: w1439 -> [w1629]
        tunnel: [w1628] -> w1434
        tunnel: w1438 -> [w1628]
        i -> [w1656]
        stop <- w1652 stop-if-true
        # "Drives towards cube, uses pixy cam's \"x\" value to stay on center"
        n666 = Increment(x=w1656) -> (x+1=w1655:i32)
        n667 = Greater Or Equal?(x=w1655, y=100) -> (x >= y?=w1653:bool)
        n668 = call <vilib>:"WPI_DigitalInputRefNum Registry Get.vi"("refnum name"="Color Mark") -> ("DigitalInputDevRef"=w1642:T18)  [unwired: 9 in, 1 out]
        n669 = call <vilib>:"WPI_MotorControlRefNum Registry Get.vi"("refnum name"="Acquire") -> ("error out"=w1639:errorcluster, "MotorControlDevRef"=w1640:T8)  [unwired: 9 in]
        n670 = call <vilib>:"WPI_DigitalInputGetValue.vi"("DigitalInputDevRef"=w1642) -> ("Value"=w1632:bool)  [unwired: 8 in, 2 out]
        n671 = And(x=w1632, y=w1653) -> (x .and. y?=w1652:bool)
        n672 = Wait (ms)(milliseconds to wait=u32 20) -> ()  [unwired: 1 out]
        n673 = Select(t=0.0, s=w1632, f=0.6) -> (s? t:f=w1633:dbl)
        n674 = Select(t=0.0, s=w1632, f=0.6) -> (s? t:f=w1636:dbl)
        n675 = call <vilib>:"WPI_MotorControlSetOutput.vi"("error in (no error)"=w1639, "Output"=w1633, "MotorControlDevRef"=w1640) -> ()  [unwired: 6 in, 3 out]
        n676 = call "PIXY VI.vi"() -> ("X"=w1643:dbl)  [unwired: 14 in, 5 out]
        n677 = call <vilib>:"WPI_RobotDriveRefNum Registry Get.vi"("refnum name"="RobotDrive") -> ("error out"=w1648:errorcluster, "RobotDriveDevRef"=w1649:T15)  [unwired: 9 in]
        n678 = call-poly <vilib>:"PID.vi"("output range"=cluster{"output high":dbl, "output low":dbl} {"output high"=0.4, "output low"=-0.4}, "PID gains"=T7 {"proportional gain (Kc)"=0.11, "integral time (Ti, min)"=0.0, "derivative time (Td, min)"=0.0}, "process variable"=w1643, "setpoint"=0.0) -> ("output"=w1646:dbl)  [unwired: 6 in, 1 out]
        n679 = Negate(x=w1646) -> (-x=w1645:dbl)
        n680 = call-poly <vilib>:"WPI_RobotDriveArcadeDrive.vi"("error in (no error)"=w1648, "Y axis value"=w1636, "X axis value"=w1645, "RobotDriveDevRef"=w1649) -> ()  [unwired: 5 in, 3 out]
      }
      n681 = while {
        tunnel: [w1542] -> w1433
        tunnel: w1437 -> [w1542]
        tunnel: [w1541] -> w1432
        tunnel: w1436 -> [w1541]
        tunnel: [w1544] -> w1431
        tunnel: w1435 -> [w1544]
        tunnel: [w1543] -> w1430
        tunnel: w1434 -> [w1543]
        i -> [w1567]
        stop <- w1563 stop-if-true
        n682 = global read "Robot Global Data.vi" "YAW"() -> (w1552:dbl)
        n683 = call <vilib>:"WPI_RobotDriveRefNum Registry Get.vi"("refnum name"="RobotDrive") -> ("error out"=w1550:errorcluster, "RobotDriveDevRef"=w1551:T15)  [unwired: 9 in]
        n684 = Wait (ms)(milliseconds to wait=u32 20) -> ()  [unwired: 1 out]
        n685 = Increment(x=w1567) -> (x+1=w1566:i32)
        n686 = call-poly <vilib>:"PID.vi"("output range"=cluster{"output high":dbl, "output low":dbl} {"output high"=0.4, "output low"=-0.4}, "PID gains"=T7 {"proportional gain (Kc)"=0.11, "integral time (Ti, min)"=0.0, "derivative time (Td, min)"=0.0}, "process variable"=w1552, "setpoint"=-25.0) -> ("output"=w1546:dbl)  [unwired: 6 in, 1 out]
        n687 = Greater Or Equal?(x=w1566, y=100) -> (x >= y?=w1564:bool)
        n688 = Negate(x=w1546) -> (-x=w1545:dbl)
        n689 = call-poly <vilib>:"CTRE_Phoenix_MotorController_Get_Enhanced.vi"("PhoenixMotorControlDevRef"=w1542, "error in"=w1541) -> ("Quadrature Position"=w1562:i32)  [unwired: 10 in, 3 out]
        n690 = To Double Precision Float(number=w1562) -> (double precision float=w1561:dbl)
        n691 = feedback #11() -> (w1547:dbl)  [unwired: 1 in]
        n692 = call-poly <vilib>:"WPI_RobotDriveArcadeDrive.vi"("error in (no error)"=w1550, "Y axis value"=w1547, "X axis value"=w1545, "RobotDriveDevRef"=w1551) -> ()  [unwired: 5 in, 3 out]
        n693 = Absolute Value(x=w1561) -> (abs(x)=w1557:dbl)
        n694 = Greater Or Equal?(x=w1557, y=115000.0 ("upper limit")) -> (x >= y?=w1548:bool)
        n695 = And(x=w1548, y=w1564) -> (x .and. y?=w1563:bool)
        n696 = Select(t=0.0, s=w1548, f=-0.6) -> (s? t:f=w1558:dbl)
        n697 = feedback-in #11(w1558) -> ()
      }
      n698 = while {
        tunnel: w1433 -> [w1525]
        tunnel: w1432 -> [w1524]
        tunnel: w1431 -> [w1523]
        tunnel: w1430 -> [w1522]
        tunnel: [w1525] -> w1429
        tunnel: [w1524] -> w1428
        tunnel: [w1523] -> w1427
        tunnel: [w1522] -> w1426
        i -> [w1534]
        stop <- w1532 stop-if-true
        n699 = global read "Robot Global Data.vi" "YAW"() -> (w1538:dbl)
        n700 = Increment(x=w1534) -> (x+1=w1536:i32)
        n701 = call-poly <vilib>:"PID.vi"("output range"=cluster{"output high":dbl, "output low":dbl} {"output high"=0.7, "output low"=-0.7}, "PID gains"=T7 {"proportional gain (Kc)"=0.045, "integral time (Ti, min)"=0.0, "derivative time (Td, min)"=0.0}, "process variable"=w1538, "setpoint"=-90.0) -> ("output"=w1527:dbl)  [unwired: 6 in, 1 out]
        n702 = call <vilib>:"WPI_RobotDriveRefNum Registry Get.vi"("refnum name"="RobotDrive") -> ("error out"=w1530:errorcluster, "RobotDriveDevRef"=w1531:T15)  [unwired: 9 in]
        n703 = Greater?(x=w1536, y=200) -> (0:w1532:bool)
        n704 = Negate(x=w1527) -> (-x=w1526:dbl)
        n705 = call-poly <vilib>:"WPI_RobotDriveArcadeDrive.vi"("error in (no error)"=w1530, "Y axis value"=0.0, "X axis value"=w1526, "RobotDriveDevRef"=w1531) -> ()  [unwired: 5 in, 3 out]
        n706 = Wait (ms)(milliseconds to wait=u32 20) -> ()  [unwired: 1 out]
      }
      n707 = while {
        tunnel: [w1599] -> w1425
        tunnel: w1429 -> [w1599]
        tunnel: w1428 -> [w1598]
        tunnel: [w1598] -> w1424
        tunnel: [w1601] -> w1423
        tunnel: w1427 -> [w1601]
        tunnel: [w1600] -> w1422
        tunnel: w1426 -> [w1600]
        i -> [w1625]
        stop <- w1621 stop-if-true
        n708 = global read "Robot Global Data.vi" "YAW"() -> (w1609:dbl)
        n709 = call <vilib>:"WPI_RobotDriveRefNum Registry Get.vi"("refnum name"="RobotDrive") -> ("error out"=w1607:errorcluster, "RobotDriveDevRef"=w1608:T15)  [unwired: 9 in]
        n710 = Increment(x=w1625) -> (x+1=w1624:i32)
        n711 = Wait (ms)(milliseconds to wait=u32 20) -> ()  [unwired: 1 out]
        n712 = call-poly <vilib>:"PID.vi"("output range"=cluster{"output high":dbl, "output low":dbl} {"output high"=0.4, "output low"=-0.4}, "PID gains"=T7 {"proportional gain (Kc)"=0.11, "integral time (Ti, min)"=0.0, "derivative time (Td, min)"=0.0}, "process variable"=w1609, "setpoint"=0.0) -> ("output"=w1605:dbl)  [unwired: 6 in, 1 out]
        n713 = Greater Or Equal?(x=w1624, y=20) -> (x >= y?=w1622:bool)
        n714 = Negate(x=w1605) -> (-x=w1604:dbl)
        n715 = Wait (ms)(milliseconds to wait=u32 20) -> ()  [unwired: 1 out]
        n716 = call-poly <vilib>:"CTRE_Phoenix_MotorController_Get_Enhanced.vi"("PhoenixMotorControlDevRef"=w1599, "error in"=w1598) -> ("Quadrature Position"=w1620:i32)  [unwired: 10 in, 3 out]
        n717 = To Double Precision Float(number=w1620) -> (double precision float=w1619:dbl)
        n718 = feedback #12() -> (w1603:dbl)  [unwired: 1 in]
        n719 = call-poly <vilib>:"WPI_RobotDriveArcadeDrive.vi"("error in (no error)"=w1607, "Y axis value"=w1603, "X axis value"=w1604, "RobotDriveDevRef"=w1608) -> ()  [unwired: 5 in, 3 out]
        n720 = Absolute Value(x=w1619) -> (abs(x)=w1615:dbl)
        n721 = Greater Or Equal?(x=w1615, y=113500.0 ("upper limit")) -> (x >= y?=w1613:bool)
        n722 = And(x=w1613, y=w1622) -> (x .and. y?=w1621:bool)
        n723 = Select(t=0.0, s=w1613, f=-0.6) -> (s? t:f=w1616:dbl)
        n724 = feedback-in #12(w1616) -> ()
      }
      n725 = while {
        tunnel: [w1487] -> _
        tunnel: w1425 -> [w1487]
        tunnel: [w1486] -> _
        tunnel: w1424 -> [w1486]
        tunnel: [w1485] -> _
        tunnel: w1423 -> [w1485]
        tunnel: [w1484] -> _
        tunnel: w1422 -> [w1484]
        i -> [w1511]
        stop <- w1488 stop-if-true
        # "Set config to shoot level, Rev, Shoot, and reset"
        n726 = global read "Robot Global Data.vi" "Pot 1"() -> (w1516:dbl)
        n727 = call <vilib>:"WPI_MotorControlRefNum Registry Get.vi"("refnum name"="Acquire") -> ("error out"=w1513:errorcluster, "MotorControlDevRef"=w1514:T8)  [unwired: 9 in]
        n728 = call <vilib>:"WPI_MotorControlRefNum Registry Get.vi"("refnum name"="Dart 1") -> ("error out"=w1520:errorcluster, "MotorControlDevRef"=w1519:T8)  [unwired: 9 in]
        n729 = Increment(x=w1511) -> (x+1=w1512:i32)
        n730 = call-poly <vilib>:"PID.vi"("PID gains"=T7 {"proportional gain (Kc)"=1.0, "integral time (Ti, min)"=0.01, "derivative time (Td, min)"=0.0}, "process variable"=w1516, "setpoint"=0.0) -> ("output"=w1521:dbl)  [unwired: 7 in, 1 out]
        n731 = Greater Or Equal?(x=w1512, y=100) -> (x >= y?=w1503:bool)
        n732 = call <vilib>:"WPI_MotorControlSetOutput.vi"("error in (no error)"=w1520, "Output"=w1521, "MotorControlDevRef"=w1519) -> ()  [unwired: 6 in, 3 out]
        n733 = call <vilib>:"WPI_MotorControlSetOutput.vi"("error in (no error)"=w1513, "Output"=-1.0, "MotorControlDevRef"=w1514) -> ()  [unwired: 6 in, 3 out]
        n734 = Select(t=WPI_SolenoidValue."Forward" ("Value"), s=w1503, f=WPI_SolenoidValue."Off" ("Value")) -> (s? t:f=w1506:T6)
        n735 = Wait (ms)(milliseconds to wait=u32 20) -> ()  [unwired: 1 out]
        n736 = call <vilib>:"WPI_SolenoidRefNum Registry Get.vi"("refnum name"="Push") -> ("error out"=w1507:errorcluster, "SolenoidDevRef"=w1508:T16)  [unwired: 9 in]
        n737 = call-poly <vilib>:"WPI_SolenoidSet.vi"("error in (no error)"=w1507, "Value"=w1506, "SolenoidDevRef"=w1508) -> ("error out"=w1499:errorcluster, "SolenoidDevRef"=w1500:T16)  [unwired: 7 in]
        n738 = call-poly <vilib>:"WPI_SolenoidGet.vi"("error in (no error)"=w1499, "SolenoidDevRef"=w1500) -> ("Value"=w1498:bool)  [unwired: 7 in, 2 out]
        n739 = And(x=w1503, y=w1498) -> (x .and. y?=w1489:bool)
        n740 = Select(t=WPI_SolenoidValue."Reverse" ("Value"), s=w1489, f=WPI_SolenoidValue."Off" ("Value")) -> (s? t:f=w1494:T6)
        n741 = call <vilib>:"WPI_SolenoidRefNum Registry Get.vi"("refnum name"="Push") -> ("error out"=w1495:errorcluster, "SolenoidDevRef"=w1496:T16)  [unwired: 9 in]
        n742 = call-poly <vilib>:"WPI_SolenoidSet.vi"("error in (no error)"=w1495, "Value"=w1494, "SolenoidDevRef"=w1496) -> ("error out"=w1490:errorcluster, "SolenoidDevRef"=w1491:T16)  [unwired: 7 in]
        n743 = call-poly <vilib>:"WPI_SolenoidGet.vi"("error in (no error)"=w1490, "SolenoidDevRef"=w1491) -> ("Value"=w1488:bool)  [unwired: 7 in, 2 out]
      }
    }
    frame "Place 2 Switch Left" {
      # "done"
      n744 = call <vilib>:"WPI_MotorControlRefNum Registry Get.vi"("refnum name"="Left Lead") -> ("error out"=w1748:errorcluster, "MotorControlDevRef"=w1749:T8)  [unwired: 9 in]
      n745 = call <vilib>:"WPI_MotorControlRefNum Registry Get.vi"("refnum name"="Right Lead") -> ("error out"=w1746:errorcluster, "MotorControlDevRef"=w1747:T8)  [unwired: 9 in]
      n746 = while {
        tunnel: w1749 -> [w2031]
        tunnel: w1748 -> [w2030]
        tunnel: w1747 -> [w2029]
        tunnel: w1746 -> [w2028]
        tunnel: [w2031] -> w1789
        tunnel: [w2030] -> w1788
        tunnel: [w2029] -> w1787
        tunnel: [w2028] -> w1786
        i -> [w2041]
        stop <- w2040 stop-if-true
        n747 = Increment(x=w2041) -> (x+1=w2043:i32)
        n748 = Greater?(x=w2043, y=10) -> (0:w2040:bool)
        n749 = call <vilib>:"CTRE_PigeonIMU_RefNumRegistryGet.vi"("refnum name"="Pigeon") -> ("PigeonIMUDevRef"=w2038:T13)  [unwired: 9 in, 1 out]
        n750 = call-poly <vilib>:"CTRE_Phoenix_MotorController_Get_Enhanced.vi"("PhoenixMotorControlDevRef"=w2031, "error in"=w2030) -> ("PhoenixMotorControlDevRef"=w2033:T8)  [unwired: 10 in, 3 out]
        n751 = call-poly <vilib>:"CTRE_Phoenix_MotorController_Get_Enhanced.vi"("PhoenixMotorControlDevRef"=w2029, "error in"=w2028) -> ("PhoenixMotorControlDevRef"=w2032:T8)  [unwired: 10 in, 3 out]
        n752 = call "CTRE_Phoenix_MotorControl_SetQuadraturePosition_Enhanced.vi"("New Position"=0, "PhoenixMotorControlDevRef"=w2032) -> ()  [unwired: 8 in, 2 out]
        n753 = call "CTRE_Phoenix_MotorControl_SetQuadraturePosition_Enhanced.vi"("New Position"=0, "PhoenixMotorControlDevRef"=w2033) -> ()  [unwired: 8 in, 2 out]
        n754 = Wait (ms)(milliseconds to wait=u32 20) -> ()  [unwired: 1 out]
        n755 = call <vilib>:"CTRE_PigeonIMU_SetYaw.vi"("Value"=0.0, "PigeonIMUDevRef"=w2038) -> ()  [unwired: 8 in, 2 out]
      }
      n756 = while {
        tunnel: [w2046] -> w1785
        tunnel: w1789 -> [w2046]
        tunnel: [w2047] -> w1784
        tunnel: w1788 -> [w2047]
        tunnel: [w2054] -> w1783
        tunnel: w1787 -> [w2054]
        tunnel: [w2053] -> w1782
        tunnel: w1786 -> [w2053]
        i -> [w2070]
        stop <- w2066 stop-if-true
        n757 = global read "Robot Global Data.vi" "YAW"() -> (w2055:dbl)
        n758 = Wait (ms)(milliseconds to wait=u32 20) -> ()  [unwired: 1 out]
        n759 = call <vilib>:"WPI_RobotDriveRefNum Registry Get.vi"("refnum name"="RobotDrive") -> ("error out"=w2051:errorcluster, "RobotDriveDevRef"=w2052:T15)  [unwired: 9 in]
        n760 = Increment(x=w2070) -> (x+1=w2069:i32)
        n761 = call-poly <vilib>:"PID.vi"("output range"=cluster{"output high":dbl, "output low":dbl} {"output high"=0.4, "output low"=-0.4}, "PID gains"=T7 {"proportional gain (Kc)"=0.11, "integral time (Ti, min)"=0.0, "derivative time (Td, min)"=0.0}, "process variable"=w2055, "setpoint"=0.0) -> ("output"=w2045:dbl)  [unwired: 6 in, 1 out]
        n762 = Greater Or Equal?(x=w2069, y=100) -> (x >= y?=w2067:bool)
        n763 = Negate(x=w2045) -> (-x=w2044:dbl)
        n764 = call-poly <vilib>:"CTRE_Phoenix_MotorController_Get_Enhanced.vi"("PhoenixMotorControlDevRef"=w2046, "error in"=w2047) -> ("Quadrature Position"=w2065:i32)  [unwired: 10 in, 3 out]
        n765 = To Double Precision Float(number=w2065) -> (double precision float=w2064:dbl)
        n766 = feedback #13() -> (w2048:dbl)  [unwired: 1 in]
        n767 = call-poly <vilib>:"WPI_RobotDriveArcadeDrive.vi"("error in (no error)"=w2051, "Y axis value"=w2048, "X axis value"=w2044, "RobotDriveDevRef"=w2052) -> ()  [unwired: 5 in, 3 out]
        n768 = Absolute Value(x=w2064) -> (abs(x)=w2060:dbl)
        n769 = Greater Or Equal?(x=w2060, y=115000.0 ("upper limit")) -> (x >= y?=w2049:bool)
        n770 = And(x=w2049, y=w2067) -> (x .and. y?=w2066:bool)
        n771 = Select(t=0.0, s=w2049, f=-0.8) -> (s? t:f=w2061:dbl)
        n772 = feedback-in #13(w2061) -> ()
      }
      n773 = while {
        tunnel: w1785 -> [w2018]
        tunnel: w1784 -> [w2017]
        tunnel: w1783 -> [w2016]
        tunnel: w1782 -> [w2015]
        tunnel: [w2018] -> w1781
        tunnel: [w2017] -> w1780
        tunnel: [w2016] -> w1779
        tunnel: [w2015] -> w1778
        i -> [w2021]
        stop <- w2019 stop-if-true
        n774 = global read "Robot Global Data.vi" "YAW"() -> (w2025:dbl)
        n775 = Increment(x=w2021) -> (x+1=w2023:i32)
        n776 = call-poly <vilib>:"PID.vi"("output range"=cluster{"output high":dbl, "output low":dbl} {"output high"=0.7, "output low"=-0.7}, "PID gains"=T7 {"proportional gain (Kc)"=0.045, "integral time (Ti, min)"=0.0, "derivative time (Td, min)"=0.0}, "process variable"=w2025, "setpoint"=-90.0) -> ("output"=w2010:dbl)  [unwired: 6 in, 1 out]
        n777 = call <vilib>:"WPI_RobotDriveRefNum Registry Get.vi"("refnum name"="RobotDrive") -> ("error out"=w2013:errorcluster, "RobotDriveDevRef"=w2014:T15)  [unwired: 9 in]
        n778 = Greater?(x=w2023, y=200) -> (0:w2019:bool)
        n779 = Negate(x=w2010) -> (-x=w2009:dbl)
        n780 = call-poly <vilib>:"WPI_RobotDriveArcadeDrive.vi"("error in (no error)"=w2013, "Y axis value"=0.0, "X axis value"=w2009, "RobotDriveDevRef"=w2014) -> ()  [unwired: 5 in, 3 out]
        n781 = Wait (ms)(milliseconds to wait=u32 20) -> ()  [unwired: 1 out]
      }
      n782 = while {
        tunnel: [w1918] -> w1777
        tunnel: w1781 -> [w1918]
        tunnel: [w1917] -> w1776
        tunnel: w1780 -> [w1917]
        tunnel: [w1916] -> w1775
        tunnel: w1779 -> [w1916]
        tunnel: [w1919] -> w1774
        tunnel: w1778 -> [w1919]
        i -> [w1912]
        stop <- w1898 stop-if-true
        # "Set config to shoot level, Rev, Shoot"
        n783 = global read "Robot Global Data.vi" "Pot 1"() -> (w1920:dbl)
        n784 = call <vilib>:"WPI_MotorControlRefNum Registry Get.vi"("refnum name"="Acquire") -> ("error out"=w1913:errorcluster, "MotorControlDevRef"=w1914:T8)  [unwired: 9 in]
        n785 = call <vilib>:"WPI_MotorControlRefNum Registry Get.vi"("refnum name"="Dart 1") -> ("error out"=w1924:errorcluster, "MotorControlDevRef"=w1923:T8)  [unwired: 9 in]
        n786 = Increment(x=w1912) -> (x+1=w1899:i32)
        n787 = call-poly <vilib>:"PID.vi"("PID gains"=T7 {"proportional gain (Kc)"=1.0, "integral time (Ti, min)"=0.01, "derivative time (Td, min)"=0.0}, "process variable"=w1920, "setpoint"=0.0) -> ("output"=w1925:dbl)  [unwired: 7 in, 1 out]
        n788 = Greater Or Equal?(x=w1899, y=100) -> (x >= y?=w1904:bool)
        n789 = call <vilib>:"WPI_MotorControlSetOutput.vi"("error in (no error)"=w1924, "Output"=w1925, "MotorControlDevRef"=w1923) -> ()  [unwired: 6 in, 3 out]
        n790 = call <vilib>:"WPI_MotorControlSetOutput.vi"("error in (no error)"=w1913, "Output"=-1.0, "MotorControlDevRef"=w1914) -> ()  [unwired: 6 in, 3 out]
        n791 = Select(t=WPI_SolenoidValue."Forward" ("Value"), s=w1904, f=WPI_SolenoidValue."Off" ("Value")) -> (s? t:f=w1907:T6)
        n792 = Wait (ms)(milliseconds to wait=u32 20) -> ()  [unwired: 1 out]
        n793 = call <vilib>:"WPI_SolenoidRefNum Registry Get.vi"("refnum name"="Push") -> ("error out"=w1908:errorcluster, "SolenoidDevRef"=w1909:T16)  [unwired: 9 in]
        n794 = call-poly <vilib>:"WPI_SolenoidSet.vi"("error in (no error)"=w1908, "Value"=w1907, "SolenoidDevRef"=w1909) -> ("error out"=w1900:errorcluster, "SolenoidDevRef"=w1901:T16)  [unwired: 7 in]
        n795 = call-poly <vilib>:"WPI_SolenoidGet.vi"("error in (no error)"=w1900, "SolenoidDevRef"=w1901) -> ("Value"=w1898:bool)  [unwired: 7 in, 2 out]
      }
      n796 = while {
        tunnel: w1777 -> [w1804]
        tunnel: w1776 -> [w1803]
        tunnel: w1775 -> [w1802]
        tunnel: w1774 -> [w1801]
        tunnel: [w1804] -> w1773
        tunnel: [w1803] -> w1772
        tunnel: [w1802] -> w1771
        tunnel: [w1801] -> w1770
        i -> [w1792]
        stop <- w1791 stop-if-true
        # "Reset"
        n797 = call <vilib>:"WPI_SolenoidRefNum Registry Get.vi"("refnum name"="Push") -> ("error out"=w1808:errorcluster, "SolenoidDevRef"=w1809:T16)  [unwired: 9 in]
        n798 = call <vilib>:"WPI_MotorControlRefNum Registry Get.vi"("refnum name"="Dart 1") -> ("error out"=w1799:errorcluster, "MotorControlDevRef"=w1798:T8)  [unwired: 9 in]
        n799 = Increment(x=w1792) -> (x+1=w1805:i32)
        n800 = global read "Robot Global Data.vi" "Pot 1"() -> (w1795:dbl)
        n801 = Greater Or Equal?(x=w1805, y=100) -> (x >= y?=w1791:bool)
        n802 = call-poly <vilib>:"PID.vi"("PID gains"=T7 {"proportional gain (Kc)"=1.0, "integral time (Ti, min)"=0.01, "derivative time (Td, min)"=0.0}, "process variable"=w1795, "setpoint"=0.0) -> ("output"=w1800:dbl)  [unwired: 7 in, 1 out]
        n803 = call <vilib>:"WPI_MotorControlSetOutput.vi"("error in (no error)"=w1799, "Output"=w1800, "MotorControlDevRef"=w1798) -> ()  [unwired: 6 in, 3 out]
        n804 = call-poly <vilib>:"WPI_SolenoidSet.vi"("error in (no error)"=w1808, "Value"=WPI_SolenoidValue."Reverse", "SolenoidDevRef"=w1809) -> ("error out"=w1806:errorcluster, "SolenoidDevRef"=w1807:T16)  [unwired: 7 in]
        n805 = call-poly <vilib>:"WPI_SolenoidGet.vi"("error in (no error)"=w1806, "SolenoidDevRef"=w1807) -> ()  [unwired: 7 in, 3 out]
      }
      n806 = while {
        tunnel: [w1989] -> w1769
        tunnel: w1773 -> [w1989]
        tunnel: [w1988] -> w1768
        tunnel: w1772 -> [w1988]
        tunnel: [w1987] -> w1767
        tunnel: w1771 -> [w1987]
        tunnel: [w1986] -> w1766
        tunnel: w1770 -> [w1986]
        i -> [w2002]
        stop <- w2000 stop-if-true
        n807 = global read "Robot Global Data.vi" "YAW"() -> (w2006:dbl)
        n808 = Increment(x=w2002) -> (x+1=w2004:i32)
        n809 = call-poly <vilib>:"PID.vi"("output range"=cluster{"output high":dbl, "output low":dbl} {"output high"=0.6, "output low"=-0.6}, "PID gains"=T7 {"proportional gain (Kc)"=0.055, "integral time (Ti, min)"=0.0, "derivative time (Td, min)"=0.0}, "process variable"=w2006, "setpoint"=-25.0) -> ("output"=w1996:dbl)  [unwired: 6 in, 1 out]
        n810 = call <vilib>:"WPI_RobotDriveRefNum Registry Get.vi"("refnum name"="RobotDrive") -> ("error out"=w1997:errorcluster, "RobotDriveDevRef"=w1998:T15)  [unwired: 9 in]
        n811 = Negate(x=w1996) -> (-x=w1995:dbl)
        n812 = Greater?(x=w2004, y=180) -> (0:w2000:bool)
        n813 = call-poly <vilib>:"WPI_RobotDriveArcadeDrive.vi"("error in (no error)"=w1997, "Y axis value"=0.0, "X axis value"=w1995, "RobotDriveDevRef"=w1998) -> ()  [unwired: 5 in, 3 out]
        n814 = Wait (ms)(milliseconds to wait=u32 20) -> ()  [unwired: 1 out]
        n815 = call-poly <vilib>:"CTRE_Phoenix_MotorController_Get_Enhanced.vi"("PhoenixMotorControlDevRef"=w1989, "error in"=w1988) -> ("PhoenixMotorControlDevRef"=w1991:T8)  [unwired: 8 in, 5 out]
        n816 = call-poly <vilib>:"CTRE_Phoenix_MotorController_Get_Enhanced.vi"("PhoenixMotorControlDevRef"=w1987, "error in"=w1986) -> ("PhoenixMotorControlDevRef"=w1990:T8)  [unwired: 8 in, 5 out]
        n817 = call "CTRE_Phoenix_MotorControl_SetQuadraturePosition_Enhanced.vi"("New Position"=0, "PhoenixMotorControlDevRef"=w1990) -> ()  [unwired: 8 in, 2 out]
        n818 = call "CTRE_Phoenix_MotorControl_SetQuadraturePosition_Enhanced.vi"("New Position"=0, "PhoenixMotorControlDevRef"=w1991) -> ()  [unwired: 8 in, 2 out]
      }
      n819 = while {
        tunnel: [w1959] -> w1765
        tunnel: w1769 -> [w1959]
        tunnel: [w1958] -> w1764
        tunnel: w1768 -> [w1958]
        tunnel: [w1957] -> w1763
        tunnel: w1767 -> [w1957]
        tunnel: [w1956] -> w1762
        tunnel: w1766 -> [w1956]
        i -> [w1984]
        stop <- w1980 stop-if-true
        # "Drives towards cube, uses pixy cam's \"x\" value to stay on center"
        n820 = Increment(x=w1984) -> (x+1=w1983:i32)
        n821 = Greater Or Equal?(x=w1983, y=100) -> (x >= y?=w1981:bool)
        n822 = call <vilib>:"WPI_DigitalInputRefNum Registry Get.vi"("refnum name"="Color Mark") -> ("DigitalInputDevRef"=w1970:T18)  [unwired: 9 in, 1 out]
        n823 = call <vilib>:"WPI_MotorControlRefNum Registry Get.vi"("refnum name"="Acquire") -> ("error out"=w1967:errorcluster, "MotorControlDevRef"=w1968:T8)  [unwired: 9 in]
        n824 = call <vilib>:"WPI_DigitalInputGetValue.vi"("DigitalInputDevRef"=w1970) -> ("Value"=w1960:bool)  [unwired: 8 in, 2 out]
        n825 = And(x=w1960, y=w1981) -> (x .and. y?=w1980:bool)
        n826 = Wait (ms)(milliseconds to wait=u32 20) -> ()  [unwired: 1 out]
        n827 = Select(t=0.0, s=w1960, f=0.6) -> (s? t:f=w1961:dbl)
        n828 = Select(t=0.0, s=w1960, f=0.6) -> (s? t:f=w1964:dbl)
        n829 = call <vilib>:"WPI_MotorControlSetOutput.vi"("error in (no error)"=w1967, "Output"=w1961, "MotorControlDevRef"=w1968) -> ()  [unwired: 6 in, 3 out]
        n830 = call "PIXY VI.vi"() -> ("X"=w1971:dbl)  [unwired: 14 in, 5 out]
        n831 = call <vilib>:"WPI_RobotDriveRefNum Registry Get.vi"("refnum name"="RobotDrive") -> ("error out"=w1976:errorcluster, "RobotDriveDevRef"=w1977:T15)  [unwired: 9 in]
        n832 = call-poly <vilib>:"PID.vi"("output range"=cluster{"output high":dbl, "output low":dbl} {"output high"=0.4, "output low"=-0.4}, "PID gains"=T7 {"proportional gain (Kc)"=0.11, "integral time (Ti, min)"=0.0, "derivative time (Td, min)"=0.0}, "process variable"=w1971, "setpoint"=0.0) -> ("output"=w1974:dbl)  [unwired: 6 in, 1 out]
        n833 = Negate(x=w1974) -> (-x=w1973:dbl)
        n834 = call-poly <vilib>:"WPI_RobotDriveArcadeDrive.vi"("error in (no error)"=w1976, "Y axis value"=w1964, "X axis value"=w1973, "RobotDriveDevRef"=w1977) -> ()  [unwired: 5 in, 3 out]
      }
      n835 = while {
        tunnel: [w1870] -> w1761
        tunnel: w1765 -> [w1870]
        tunnel: [w1869] -> w1760
        tunnel: w1764 -> [w1869]
        tunnel: [w1872] -> w1759
        tunnel: w1763 -> [w1872]
        tunnel: [w1871] -> w1758
        tunnel: w1762 -> [w1871]
        i -> [w1895]
        stop <- w1891 stop-if-true
        n836 = global read "Robot Global Data.vi" "YAW"() -> (w1880:dbl)
        n837 = call <vilib>:"WPI_RobotDriveRefNum Registry Get.vi"("refnum name"="RobotDrive") -> ("error out"=w1878:errorcluster, "RobotDriveDevRef"=w1879:T15)  [unwired: 9 in]
        n838 = Wait (ms)(milliseconds to wait=u32 20) -> ()  [unwired: 1 out]
        n839 = Increment(x=w1895) -> (x+1=w1894:i32)
        n840 = call-poly <vilib>:"PID.vi"("output range"=cluster{"output high":dbl, "output low":dbl} {"output high"=0.4, "output low"=-0.4}, "PID gains"=T7 {"proportional gain (Kc)"=0.11, "integral time (Ti, min)"=0.0, "derivative time (Td, min)"=0.0}, "process variable"=w1880, "setpoint"=-25.0) -> ("output"=w1874:dbl)  [unwired: 6 in, 1 out]
        n841 = Greater Or Equal?(x=w1894, y=100) -> (x >= y?=w1892:bool)
        n842 = Negate(x=w1874) -> (-x=w1873:dbl)
        n843 = call-poly <vilib>:"CTRE_Phoenix_MotorController_Get_Enhanced.vi"("PhoenixMotorControlDevRef"=w1870, "error in"=w1869) -> ("Quadrature Position"=w1890:i32)  [unwired: 10 in, 3 out]
        n844 = To Double Precision Float(number=w1890) -> (double precision float=w1889:dbl)
        n845 = feedback #14() -> (w1875:dbl)  [unwired: 1 in]
        n846 = call-poly <vilib>:"WPI_RobotDriveArcadeDrive.vi"("error in (no error)"=w1878, "Y axis value"=w1875, "X axis value"=w1873, "RobotDriveDevRef"=w1879) -> ()  [unwired: 5 in, 3 out]
        n847 = Absolute Value(x=w1889) -> (abs(x)=w1885:dbl)
        n848 = Greater Or Equal?(x=w1885, y=115000.0 ("upper limit")) -> (x >= y?=w1876:bool)
        n849 = And(x=w1876, y=w1892) -> (x .and. y?=w1891:bool)
        n850 = Select(t=0.0, s=w1876, f=-0.6) -> (s? t:f=w1886:dbl)
        n851 = feedback-in #14(w1886) -> ()
      }
      n852 = while {
        tunnel: w1761 -> [w1853]
        tunnel: w1760 -> [w1852]
        tunnel: w1759 -> [w1851]
        tunnel: w1758 -> [w1850]
        tunnel: [w1853] -> w1757
        tunnel: [w1852] -> w1756
        tunnel: [w1851] -> w1755
        tunnel: [w1850] -> w1754
        i -> [w1862]
        stop <- w1860 stop-if-true
        n853 = global read "Robot Global Data.vi" "YAW"() -> (w1866:dbl)
        n854 = Increment(x=w1862) -> (x+1=w1864:i32)
        n855 = call-poly <vilib>:"PID.vi"("output range"=cluster{"output high":dbl, "output low":dbl} {"output high"=0.7, "output low"=-0.7}, "PID gains"=T7 {"proportional gain (Kc)"=0.045, "integral time (Ti, min)"=0.0, "derivative time (Td, min)"=0.0}, "process variable"=w1866, "setpoint"=-90.0) -> ("output"=w1855:dbl)  [unwired: 6 in, 1 out]
        n856 = call <vilib>:"WPI_RobotDriveRefNum Registry Get.vi"("refnum name"="RobotDrive") -> ("error out"=w1858:errorcluster, "RobotDriveDevRef"=w1859:T15)  [unwired: 9 in]
        n857 = Greater?(x=w1864, y=200) -> (0:w1860:bool)
        n858 = Negate(x=w1855) -> (-x=w1854:dbl)
        n859 = call-poly <vilib>:"WPI_RobotDriveArcadeDrive.vi"("error in (no error)"=w1858, "Y axis value"=0.0, "X axis value"=w1854, "RobotDriveDevRef"=w1859) -> ()  [unwired: 5 in, 3 out]
        n860 = Wait (ms)(milliseconds to wait=u32 20) -> ()  [unwired: 1 out]
      }
      n861 = while {
        tunnel: [w1927] -> w1753
        tunnel: w1757 -> [w1927]
        tunnel: w1756 -> [w1926]
        tunnel: [w1926] -> w1752
        tunnel: [w1929] -> w1751
        tunnel: w1755 -> [w1929]
        tunnel: [w1928] -> w1750
        tunnel: w1754 -> [w1928]
        i -> [w1953]
        stop <- w1949 stop-if-true
        n862 = global read "Robot Global Data.vi" "YAW"() -> (w1937:dbl)
        n863 = call <vilib>:"WPI_RobotDriveRefNum Registry Get.vi"("refnum name"="RobotDrive") -> ("error out"=w1935:errorcluster, "RobotDriveDevRef"=w1936:T15)  [unwired: 9 in]
        n864 = Increment(x=w1953) -> (x+1=w1952:i32)
        n865 = Wait (ms)(milliseconds to wait=u32 20) -> ()  [unwired: 1 out]
        n866 = call-poly <vilib>:"PID.vi"("output range"=cluster{"output high":dbl, "output low":dbl} {"output high"=0.4, "output low"=-0.4}, "PID gains"=T7 {"proportional gain (Kc)"=0.11, "integral time (Ti, min)"=0.0, "derivative time (Td, min)"=0.0}, "process variable"=w1937, "setpoint"=0.0) -> ("output"=w1933:dbl)  [unwired: 6 in, 1 out]
        n867 = Greater Or Equal?(x=w1952, y=20) -> (x >= y?=w1950:bool)
        n868 = Negate(x=w1933) -> (-x=w1932:dbl)
        n869 = Wait (ms)(milliseconds to wait=u32 20) -> ()  [unwired: 1 out]
        n870 = call-poly <vilib>:"CTRE_Phoenix_MotorController_Get_Enhanced.vi"("PhoenixMotorControlDevRef"=w1927, "error in"=w1926) -> ("Quadrature Position"=w1948:i32)  [unwired: 10 in, 3 out]
        n871 = To Double Precision Float(number=w1948) -> (double precision float=w1947:dbl)
        n872 = feedback #15() -> (w1931:dbl)  [unwired: 1 in]
        n873 = call-poly <vilib>:"WPI_RobotDriveArcadeDrive.vi"("error in (no error)"=w1935, "Y axis value"=w1931, "X axis value"=w1932, "RobotDriveDevRef"=w1936) -> ()  [unwired: 5 in, 3 out]
        n874 = Absolute Value(x=w1947) -> (abs(x)=w1943:dbl)
        n875 = Greater Or Equal?(x=w1943, y=113500.0 ("upper limit")) -> (x >= y?=w1941:bool)
        n876 = And(x=w1941, y=w1950) -> (x .and. y?=w1949:bool)
        n877 = Select(t=0.0, s=w1941, f=-0.6) -> (s? t:f=w1944:dbl)
        n878 = feedback-in #15(w1944) -> ()
      }
      n879 = while {
        tunnel: [w1815] -> _
        tunnel: w1753 -> [w1815]
        tunnel: [w1814] -> _
        tunnel: w1752 -> [w1814]
        tunnel: [w1813] -> _
        tunnel: w1751 -> [w1813]
        tunnel: [w1812] -> _
        tunnel: w1750 -> [w1812]
        i -> [w1839]
        stop <- w1816 stop-if-true
        # "Set config to shoot level, Rev, Shoot, and reset"
        n880 = global read "Robot Global Data.vi" "Pot 1"() -> (w1844:dbl)
        n881 = call <vilib>:"WPI_MotorControlRefNum Registry Get.vi"("refnum name"="Acquire") -> ("error out"=w1841:errorcluster, "MotorControlDevRef"=w1842:T8)  [unwired: 9 in]
        n882 = call <vilib>:"WPI_MotorControlRefNum Registry Get.vi"("refnum name"="Dart 1") -> ("error out"=w1848:errorcluster, "MotorControlDevRef"=w1847:T8)  [unwired: 9 in]
        n883 = Increment(x=w1839) -> (x+1=w1840:i32)
        n884 = call-poly <vilib>:"PID.vi"("PID gains"=T7 {"proportional gain (Kc)"=1.0, "integral time (Ti, min)"=0.01, "derivative time (Td, min)"=0.0}, "process variable"=w1844, "setpoint"=0.0) -> ("output"=w1849:dbl)  [unwired: 7 in, 1 out]
        n885 = Greater Or Equal?(x=w1840, y=100) -> (x >= y?=w1831:bool)
        n886 = call <vilib>:"WPI_MotorControlSetOutput.vi"("error in (no error)"=w1848, "Output"=w1849, "MotorControlDevRef"=w1847) -> ()  [unwired: 6 in, 3 out]
        n887 = call <vilib>:"WPI_MotorControlSetOutput.vi"("error in (no error)"=w1841, "Output"=-1.0, "MotorControlDevRef"=w1842) -> ()  [unwired: 6 in, 3 out]
        n888 = Select(t=WPI_SolenoidValue."Forward" ("Value"), s=w1831, f=WPI_SolenoidValue."Off" ("Value")) -> (s? t:f=w1834:T6)
        n889 = Wait (ms)(milliseconds to wait=u32 20) -> ()  [unwired: 1 out]
        n890 = call <vilib>:"WPI_SolenoidRefNum Registry Get.vi"("refnum name"="Push") -> ("error out"=w1835:errorcluster, "SolenoidDevRef"=w1836:T16)  [unwired: 9 in]
        n891 = call-poly <vilib>:"WPI_SolenoidSet.vi"("error in (no error)"=w1835, "Value"=w1834, "SolenoidDevRef"=w1836) -> ("error out"=w1827:errorcluster, "SolenoidDevRef"=w1828:T16)  [unwired: 7 in]
        n892 = call-poly <vilib>:"WPI_SolenoidGet.vi"("error in (no error)"=w1827, "SolenoidDevRef"=w1828) -> ("Value"=w1826:bool)  [unwired: 7 in, 2 out]
        n893 = And(x=w1831, y=w1826) -> (x .and. y?=w1817:bool)
        n894 = Select(t=WPI_SolenoidValue."Reverse" ("Value"), s=w1817, f=WPI_SolenoidValue."Off" ("Value")) -> (s? t:f=w1822:T6)
        n895 = call <vilib>:"WPI_SolenoidRefNum Registry Get.vi"("refnum name"="Push") -> ("error out"=w1823:errorcluster, "SolenoidDevRef"=w1824:T16)  [unwired: 9 in]
        n896 = call-poly <vilib>:"WPI_SolenoidSet.vi"("error in (no error)"=w1823, "Value"=w1822, "SolenoidDevRef"=w1824) -> ("error out"=w1818:errorcluster, "SolenoidDevRef"=w1819:T16)  [unwired: 7 in]
        n897 = call-poly <vilib>:"WPI_SolenoidGet.vi"("error in (no error)"=w1818, "SolenoidDevRef"=w1819) -> ("Value"=w1816:bool)  [unwired: 7 in, 2 out]
      }
    }
    frame "Center Place 1 Switch Right" {
      n898 = call <vilib>:"WPI_MotorControlRefNum Registry Get.vi"("refnum name"="Left Lead") -> ("error out"=w2076:errorcluster, "MotorControlDevRef"=w2077:T8)  [unwired: 9 in]
      n899 = call <vilib>:"WPI_MotorControlRefNum Registry Get.vi"("refnum name"="Right Lead") -> ("error out"=w2074:errorcluster, "MotorControlDevRef"=w2075:T8)  [unwired: 9 in]
      n900 = while {
        tunnel: w2077 -> [w2359]
        tunnel: w2076 -> [w2358]
        tunnel: w2075 -> [w2357]
        tunnel: w2074 -> [w2356]
        tunnel: [w2359] -> w2117
        tunnel: [w2358] -> w2116
        tunnel: [w2357] -> w2115
        tunnel: [w2356] -> w2114
        i -> [w2369]
        stop <- w2368 stop-if-true
        n901 = Increment(x=w2369) -> (x+1=w2371:i32)
        n902 = Greater?(x=w2371, y=10) -> (0:w2368:bool)
        n903 = call <vilib>:"CTRE_PigeonIMU_RefNumRegistryGet.vi"("refnum name"="Pigeon") -> ("PigeonIMUDevRef"=w2366:T13)  [unwired: 9 in, 1 out]
        n904 = call-poly <vilib>:"CTRE_Phoenix_MotorController_Get_Enhanced.vi"("PhoenixMotorControlDevRef"=w2359, "error in"=w2358) -> ("PhoenixMotorControlDevRef"=w2361:T8)  [unwired: 10 in, 3 out]
        n905 = call-poly <vilib>:"CTRE_Phoenix_MotorController_Get_Enhanced.vi"("PhoenixMotorControlDevRef"=w2357, "error in"=w2356) -> ("PhoenixMotorControlDevRef"=w2360:T8)  [unwired: 10 in, 3 out]
        n906 = call "CTRE_Phoenix_MotorControl_SetQuadraturePosition_Enhanced.vi"("New Position"=0, "PhoenixMotorControlDevRef"=w2360) -> ()  [unwired: 8 in, 2 out]
        n907 = call "CTRE_Phoenix_MotorControl_SetQuadraturePosition_Enhanced.vi"("New Position"=0, "PhoenixMotorControlDevRef"=w2361) -> ()  [unwired: 8 in, 2 out]
        n908 = Wait (ms)(milliseconds to wait=u32 20) -> ()  [unwired: 1 out]
        n909 = call <vilib>:"CTRE_PigeonIMU_SetYaw.vi"("Value"=0.0, "PigeonIMUDevRef"=w2366) -> ()  [unwired: 8 in, 2 out]
      }
      n910 = while {
        tunnel: [w2374] -> w2113
        tunnel: w2117 -> [w2374]
        tunnel: [w2375] -> w2112
        tunnel: w2116 -> [w2375]
        tunnel: [w2382] -> w2111
        tunnel: w2115 -> [w2382]
        tunnel: [w2381] -> w2110
        tunnel: w2114 -> [w2381]
        i -> [w2398]
        stop <- w2394 stop-if-true
        n911 = global read "Robot Global Data.vi" "YAW"() -> (w2383:dbl)
        n912 = Wait (ms)(milliseconds to wait=u32 20) -> ()  [unwired: 1 out]
        n913 = call <vilib>:"WPI_RobotDriveRefNum Registry Get.vi"("refnum name"="RobotDrive") -> ("error out"=w2379:errorcluster, "RobotDriveDevRef"=w2380:T15)  [unwired: 9 in]
        n914 = Increment(x=w2398) -> (x+1=w2397:i32)
        n915 = call-poly <vilib>:"PID.vi"("output range"=cluster{"output high":dbl, "output low":dbl} {"output high"=0.4, "output low"=-0.4}, "PID gains"=T7 {"proportional gain (Kc)"=0.11, "integral time (Ti, min)"=0.0, "derivative time (Td, min)"=0.0}, "process variable"=w2383, "setpoint"=0.0) -> ("output"=w2373:dbl)  [unwired: 6 in, 1 out]
        n916 = Greater Or Equal?(x=w2397, y=100) -> (x >= y?=w2395:bool)
        n917 = Negate(x=w2373) -> (-x=w2372:dbl)
        n918 = call-poly <vilib>:"CTRE_Phoenix_MotorController_Get_Enhanced.vi"("PhoenixMotorControlDevRef"=w2374, "error in"=w2375) -> ("Quadrature Position"=w2393:i32)  [unwired: 10 in, 3 out]
        n919 = To Double Precision Float(number=w2393) -> (double precision float=w2392:dbl)
        n920 = feedback #16() -> (w2376:dbl)  [unwired: 1 in]
        n921 = call-poly <vilib>:"WPI_RobotDriveArcadeDrive.vi"("error in (no error)"=w2379, "Y axis value"=w2376, "X axis value"=w2372, "RobotDriveDevRef"=w2380) -> ()  [unwired: 5 in, 3 out]
        n922 = Absolute Value(x=w2392) -> (abs(x)=w2388:dbl)
        n923 = Greater Or Equal?(x=w2388, y=115000.0 ("upper limit")) -> (x >= y?=w2377:bool)
        n924 = And(x=w2377, y=w2395) -> (x .and. y?=w2394:bool)
        n925 = Select(t=0.0, s=w2377, f=-0.8) -> (s? t:f=w2389:dbl)
        n926 = feedback-in #16(w2389) -> ()
      }
      n927 = while {
        tunnel: w2113 -> [w2346]
        tunnel: w2112 -> [w2345]
        tunnel: w2111 -> [w2344]
        tunnel: w2110 -> [w2343]
        tunnel: [w2346] -> w2109
        tunnel: [w2345] -> w2108
        tunnel: [w2344] -> w2107
        tunnel: [w2343] -> w2106
        i -> [w2349]
        stop <- w2347 stop-if-true
        n928 = global read "Robot Global Data.vi" "YAW"() -> (w2353:dbl)
        n929 = Increment(x=w2349) -> (x+1=w2351:i32)
        n930 = call-poly <vilib>:"PID.vi"("output range"=cluster{"output high":dbl, "output low":dbl} {"output high"=0.7, "output low"=-0.7}, "PID gains"=T7 {"proportional gain (Kc)"=0.045, "integral time (Ti, min)"=0.0, "derivative time (Td, min)"=0.0}, "process variable"=w2353, "setpoint"=-90.0) -> ("output"=w2338:dbl)  [unwired: 6 in, 1 out]
        n931 = call <vilib>:"WPI_RobotDriveRefNum Registry Get.vi"("refnum name"="RobotDrive") -> ("error out"=w2341:errorcluster, "RobotDriveDevRef"=w2342:T15)  [unwired: 9 in]
        n932 = Greater?(x=w2351, y=200) -> (0:w2347:bool)
        n933 = Negate(x=w2338) -> (-x=w2337:dbl)
        n934 = call-poly <vilib>:"WPI_RobotDriveArcadeDrive.vi"("error in (no error)"=w2341, "Y axis value"=0.0, "X axis value"=w2337, "RobotDriveDevRef"=w2342) -> ()  [unwired: 5 in, 3 out]
        n935 = Wait (ms)(milliseconds to wait=u32 20) -> ()  [unwired: 1 out]
      }
      n936 = while {
        tunnel: [w2246] -> w2105
        tunnel: w2109 -> [w2246]
        tunnel: [w2245] -> w2104
        tunnel: w2108 -> [w2245]
        tunnel: [w2244] -> w2103
        tunnel: w2107 -> [w2244]
        tunnel: [w2247] -> w2102
        tunnel: w2106 -> [w2247]
        i -> [w2240]
        stop <- w2226 stop-if-true
        # "Set config to shoot level, Rev, Shoot"
        n937 = global read "Robot Global Data.vi" "Pot 1"() -> (w2248:dbl)
        n938 = call <vilib>:"WPI_MotorControlRefNum Registry Get.vi"("refnum name"="Acquire") -> ("error out"=w2241:errorcluster, "MotorControlDevRef"=w2242:T8)  [unwired: 9 in]
        n939 = call <vilib>:"WPI_MotorControlRefNum Registry Get.vi"("refnum name"="Dart 1") -> ("error out"=w2252:errorcluster, "MotorControlDevRef"=w2251:T8)  [unwired: 9 in]
        n940 = Increment(x=w2240) -> (x+1=w2227:i32)
        n941 = call-poly <vilib>:"PID.vi"("PID gains"=T7 {"proportional gain (Kc)"=1.0, "integral time (Ti, min)"=0.01, "derivative time (Td, min)"=0.0}, "process variable"=w2248, "setpoint"=0.0) -> ("output"=w2253:dbl)  [unwired: 7 in, 1 out]
        n942 = Greater Or Equal?(x=w2227, y=100) -> (x >= y?=w2232:bool)
        n943 = call <vilib>:"WPI_MotorControlSetOutput.vi"("error in (no error)"=w2252, "Output"=w2253, "MotorControlDevRef"=w2251) -> ()  [unwired: 6 in, 3 out]
        n944 = call <vilib>:"WPI_MotorControlSetOutput.vi"("error in (no error)"=w2241, "Output"=-1.0, "MotorControlDevRef"=w2242) -> ()  [unwired: 6 in, 3 out]
        n945 = Select(t=WPI_SolenoidValue."Forward" ("Value"), s=w2232, f=WPI_SolenoidValue."Off" ("Value")) -> (s? t:f=w2235:T6)
        n946 = Wait (ms)(milliseconds to wait=u32 20) -> ()  [unwired: 1 out]
        n947 = call <vilib>:"WPI_SolenoidRefNum Registry Get.vi"("refnum name"="Push") -> ("error out"=w2236:errorcluster, "SolenoidDevRef"=w2237:T16)  [unwired: 9 in]
        n948 = call-poly <vilib>:"WPI_SolenoidSet.vi"("error in (no error)"=w2236, "Value"=w2235, "SolenoidDevRef"=w2237) -> ("error out"=w2228:errorcluster, "SolenoidDevRef"=w2229:T16)  [unwired: 7 in]
        n949 = call-poly <vilib>:"WPI_SolenoidGet.vi"("error in (no error)"=w2228, "SolenoidDevRef"=w2229) -> ("Value"=w2226:bool)  [unwired: 7 in, 2 out]
      }
      n950 = while {
        tunnel: w2105 -> [w2132]
        tunnel: w2104 -> [w2131]
        tunnel: w2103 -> [w2130]
        tunnel: w2102 -> [w2129]
        tunnel: [w2132] -> w2101
        tunnel: [w2131] -> w2100
        tunnel: [w2130] -> w2099
        tunnel: [w2129] -> w2098
        i -> [w2120]
        stop <- w2119 stop-if-true
        # "Reset"
        n951 = call <vilib>:"WPI_SolenoidRefNum Registry Get.vi"("refnum name"="Push") -> ("error out"=w2136:errorcluster, "SolenoidDevRef"=w2137:T16)  [unwired: 9 in]
        n952 = call <vilib>:"WPI_MotorControlRefNum Registry Get.vi"("refnum name"="Dart 1") -> ("error out"=w2127:errorcluster, "MotorControlDevRef"=w2126:T8)  [unwired: 9 in]
        n953 = Increment(x=w2120) -> (x+1=w2133:i32)
        n954 = global read "Robot Global Data.vi" "Pot 1"() -> (w2123:dbl)
        n955 = Greater Or Equal?(x=w2133, y=100) -> (x >= y?=w2119:bool)
        n956 = call-poly <vilib>:"PID.vi"("PID gains"=T7 {"proportional gain (Kc)"=1.0, "integral time (Ti, min)"=0.01, "derivative time (Td, min)"=0.0}, "process variable"=w2123, "setpoint"=0.0) -> ("output"=w2128:dbl)  [unwired: 7 in, 1 out]
        n957 = call <vilib>:"WPI_MotorControlSetOutput.vi"("error in (no error)"=w2127, "Output"=w2128, "MotorControlDevRef"=w2126) -> ()  [unwired: 6 in, 3 out]
        n958 = call-poly <vilib>:"WPI_SolenoidSet.vi"("error in (no error)"=w2136, "Value"=WPI_SolenoidValue."Reverse", "SolenoidDevRef"=w2137) -> ("error out"=w2134:errorcluster, "SolenoidDevRef"=w2135:T16)  [unwired: 7 in]
        n959 = call-poly <vilib>:"WPI_SolenoidGet.vi"("error in (no error)"=w2134, "SolenoidDevRef"=w2135) -> ()  [unwired: 7 in, 3 out]
      }
      n960 = while {
        tunnel: [w2317] -> w2097
        tunnel: w2101 -> [w2317]
        tunnel: [w2316] -> w2096
        tunnel: w2100 -> [w2316]
        tunnel: [w2315] -> w2095
        tunnel: w2099 -> [w2315]
        tunnel: [w2314] -> w2094
        tunnel: w2098 -> [w2314]
        i -> [w2330]
        stop <- w2328 stop-if-true
        n961 = global read "Robot Global Data.vi" "YAW"() -> (w2334:dbl)
        n962 = Increment(x=w2330) -> (x+1=w2332:i32)
        n963 = call-poly <vilib>:"PID.vi"("output range"=cluster{"output high":dbl, "output low":dbl} {"output high"=0.6, "output low"=-0.6}, "PID gains"=T7 {"proportional gain (Kc)"=0.055, "integral time (Ti, min)"=0.0, "derivative time (Td, min)"=0.0}, "process variable"=w2334, "setpoint"=-25.0) -> ("output"=w2324:dbl)  [unwired: 6 in, 1 out]
        n964 = call <vilib>:"WPI_RobotDriveRefNum Registry Get.vi"("refnum name"="RobotDrive") -> ("error out"=w2325:errorcluster, "RobotDriveDevRef"=w2326:T15)  [unwired: 9 in]
        n965 = Negate(x=w2324) -> (-x=w2323:dbl)
        n966 = Greater?(x=w2332, y=180) -> (0:w2328:bool)
        n967 = call-poly <vilib>:"WPI_RobotDriveArcadeDrive.vi"("error in (no error)"=w2325, "Y axis value"=0.0, "X axis value"=w2323, "RobotDriveDevRef"=w2326) -> ()  [unwired: 5 in, 3 out]
        n968 = Wait (ms)(milliseconds to wait=u32 20) -> ()  [unwired: 1 out]
        n969 = call-poly <vilib>:"CTRE_Phoenix_MotorController_Get_Enhanced.vi"("PhoenixMotorControlDevRef"=w2317, "error in"=w2316) -> ("PhoenixMotorControlDevRef"=w2319:T8)  [unwired: 8 in, 5 out]
        n970 = call-poly <vilib>:"CTRE_Phoenix_MotorController_Get_Enhanced.vi"("PhoenixMotorControlDevRef"=w2315, "error in"=w2314) -> ("PhoenixMotorControlDevRef"=w2318:T8)  [unwired: 8 in, 5 out]
        n971 = call "CTRE_Phoenix_MotorControl_SetQuadraturePosition_Enhanced.vi"("New Position"=0, "PhoenixMotorControlDevRef"=w2318) -> ()  [unwired: 8 in, 2 out]
        n972 = call "CTRE_Phoenix_MotorControl_SetQuadraturePosition_Enhanced.vi"("New Position"=0, "PhoenixMotorControlDevRef"=w2319) -> ()  [unwired: 8 in, 2 out]
      }
      n973 = while {
        tunnel: [w2287] -> w2093
        tunnel: w2097 -> [w2287]
        tunnel: [w2286] -> w2092
        tunnel: w2096 -> [w2286]
        tunnel: [w2285] -> w2091
        tunnel: w2095 -> [w2285]
        tunnel: [w2284] -> w2090
        tunnel: w2094 -> [w2284]
        i -> [w2312]
        stop <- w2308 stop-if-true
        # "Drives towards cube, uses pixy cam's \"x\" value to stay on center"
        n974 = Increment(x=w2312) -> (x+1=w2311:i32)
        n975 = Greater Or Equal?(x=w2311, y=100) -> (x >= y?=w2309:bool)
        n976 = call <vilib>:"WPI_DigitalInputRefNum Registry Get.vi"("refnum name"="Color Mark") -> ("DigitalInputDevRef"=w2298:T18)  [unwired: 9 in, 1 out]
        n977 = call <vilib>:"WPI_MotorControlRefNum Registry Get.vi"("refnum name"="Acquire") -> ("error out"=w2295:errorcluster, "MotorControlDevRef"=w2296:T8)  [unwired: 9 in]
        n978 = call <vilib>:"WPI_DigitalInputGetValue.vi"("DigitalInputDevRef"=w2298) -> ("Value"=w2288:bool)  [unwired: 8 in, 2 out]
        n979 = And(x=w2288, y=w2309) -> (x .and. y?=w2308:bool)
        n980 = Wait (ms)(milliseconds to wait=u32 20) -> ()  [unwired: 1 out]
        n981 = Select(t=0.0, s=w2288, f=0.6) -> (s? t:f=w2289:dbl)
        n982 = Select(t=0.0, s=w2288, f=0.6) -> (s? t:f=w2292:dbl)
        n983 = call <vilib>:"WPI_MotorControlSetOutput.vi"("error in (no error)"=w2295, "Output"=w2289, "MotorControlDevRef"=w2296) -> ()  [unwired: 6 in, 3 out]
        n984 = call "PIXY VI.vi"() -> ("X"=w2299:dbl)  [unwired: 14 in, 5 out]
        n985 = call <vilib>:"WPI_RobotDriveRefNum Registry Get.vi"("refnum name"="RobotDrive") -> ("error out"=w2304:errorcluster, "RobotDriveDevRef"=w2305:T15)  [unwired: 9 in]
        n986 = call-poly <vilib>:"PID.vi"("output range"=cluster{"output high":dbl, "output low":dbl} {"output high"=0.4, "output low"=-0.4}, "PID gains"=T7 {"proportional gain (Kc)"=0.11, "integral time (Ti, min)"=0.0, "derivative time (Td, min)"=0.0}, "process variable"=w2299, "setpoint"=0.0) -> ("output"=w2302:dbl)  [unwired: 6 in, 1 out]
        n987 = Negate(x=w2302) -> (-x=w2301:dbl)
        n988 = call-poly <vilib>:"WPI_RobotDriveArcadeDrive.vi"("error in (no error)"=w2304, "Y axis value"=w2292, "X axis value"=w2301, "RobotDriveDevRef"=w2305) -> ()  [unwired: 5 in, 3 out]
      }
      n989 = while {
        tunnel: [w2198] -> w2089
        tunnel: w2093 -> [w2198]
        tunnel: [w2197] -> w2088
        tunnel: w2092 -> [w2197]
        tunnel: [w2200] -> w2087
        tunnel: w2091 -> [w2200]
        tunnel: [w2199] -> w2086
        tunnel: w2090 -> [w2199]
        i -> [w2223]
        stop <- w2219 stop-if-true
        n990 = global read "Robot Global Data.vi" "YAW"() -> (w2208:dbl)
        n991 = call <vilib>:"WPI_RobotDriveRefNum Registry Get.vi"("refnum name"="RobotDrive") -> ("error out"=w2206:errorcluster, "RobotDriveDevRef"=w2207:T15)  [unwired: 9 in]
        n992 = Wait (ms)(milliseconds to wait=u32 20) -> ()  [unwired: 1 out]
        n993 = Increment(x=w2223) -> (x+1=w2222:i32)
        n994 = call-poly <vilib>:"PID.vi"("output range"=cluster{"output high":dbl, "output low":dbl} {"output high"=0.4, "output low"=-0.4}, "PID gains"=T7 {"proportional gain (Kc)"=0.11, "integral time (Ti, min)"=0.0, "derivative time (Td, min)"=0.0}, "process variable"=w2208, "setpoint"=-25.0) -> ("output"=w2202:dbl)  [unwired: 6 in, 1 out]
        n995 = Greater Or Equal?(x=w2222, y=100) -> (x >= y?=w2220:bool)
        n996 = Negate(x=w2202) -> (-x=w2201:dbl)
        n997 = call-poly <vilib>:"CTRE_Phoenix_MotorController_Get_Enhanced.vi"("PhoenixMotorControlDevRef"=w2198, "error in"=w2197) -> ("Quadrature Position"=w2218:i32)  [unwired: 10 in, 3 out]
        n998 = To Double Precision Float(number=w2218) -> (double precision float=w2217:dbl)
        n999 = feedback #17() -> (w2203:dbl)  [unwired: 1 in]
        n1000 = call-poly <vilib>:"WPI_RobotDriveArcadeDrive.vi"("error in (no error)"=w2206, "Y axis value"=w2203, "X axis value"=w2201, "RobotDriveDevRef"=w2207) -> ()  [unwired: 5 in, 3 out]
        n1001 = Absolute Value(x=w2217) -> (abs(x)=w2213:dbl)
        n1002 = Greater Or Equal?(x=w2213, y=115000.0 ("upper limit")) -> (x >= y?=w2204:bool)
        n1003 = And(x=w2204, y=w2220) -> (x .and. y?=w2219:bool)
        n1004 = Select(t=0.0, s=w2204, f=-0.6) -> (s? t:f=w2214:dbl)
        n1005 = feedback-in #17(w2214) -> ()
      }
      n1006 = while {
        tunnel: w2089 -> [w2181]
        tunnel: w2088 -> [w2180]
        tunnel: w2087 -> [w2179]
        tunnel: w2086 -> [w2178]
        tunnel: [w2181] -> w2085
        tunnel: [w2180] -> w2084
        tunnel: [w2179] -> w2083
        tunnel: [w2178] -> w2082
        i -> [w2190]
        stop <- w2188 stop-if-true
        n1007 = global read "Robot Global Data.vi" "YAW"() -> (w2194:dbl)
        n1008 = Increment(x=w2190) -> (x+1=w2192:i32)
        n1009 = call-poly <vilib>:"PID.vi"("output range"=cluster{"output high":dbl, "output low":dbl} {"output high"=0.7, "output low"=-0.7}, "PID gains"=T7 {"proportional gain (Kc)"=0.045, "integral time (Ti, min)"=0.0, "derivative time (Td, min)"=0.0}, "process variable"=w2194, "setpoint"=-90.0) -> ("output"=w2183:dbl)  [unwired: 6 in, 1 out]
        n1010 = call <vilib>:"WPI_RobotDriveRefNum Registry Get.vi"("refnum name"="RobotDrive") -> ("error out"=w2186:errorcluster, "RobotDriveDevRef"=w2187:T15)  [unwired: 9 in]
        n1011 = Greater?(x=w2192, y=200) -> (0:w2188:bool)
        n1012 = Negate(x=w2183) -> (-x=w2182:dbl)
        n1013 = call-poly <vilib>:"WPI_RobotDriveArcadeDrive.vi"("error in (no error)"=w2186, "Y axis value"=0.0, "X axis value"=w2182, "RobotDriveDevRef"=w2187) -> ()  [unwired: 5 in, 3 out]
        n1014 = Wait (ms)(milliseconds to wait=u32 20) -> ()  [unwired: 1 out]
      }
      n1015 = while {
        tunnel: [w2255] -> w2081
        tunnel: w2085 -> [w2255]
        tunnel: w2084 -> [w2254]
        tunnel: [w2254] -> w2080
        tunnel: [w2257] -> w2079
        tunnel: w2083 -> [w2257]
        tunnel: [w2256] -> w2078
        tunnel: w2082 -> [w2256]
        i -> [w2281]
        stop <- w2277 stop-if-true
        n1016 = global read "Robot Global Data.vi" "YAW"() -> (w2265:dbl)
        n1017 = call <vilib>:"WPI_RobotDriveRefNum Registry Get.vi"("refnum name"="RobotDrive") -> ("error out"=w2263:errorcluster, "RobotDriveDevRef"=w2264:T15)  [unwired: 9 in]
        n1018 = Increment(x=w2281) -> (x+1=w2280:i32)
        n1019 = Wait (ms)(milliseconds to wait=u32 20) -> ()  [unwired: 1 out]
        n1020 = call-poly <vilib>:"PID.vi"("output range"=cluster{"output high":dbl, "output low":dbl} {"output high"=0.4, "output low"=-0.4}, "PID gains"=T7 {"proportional gain (Kc)"=0.11, "integral time (Ti, min)"=0.0, "derivative time (Td, min)"=0.0}, "process variable"=w2265, "setpoint"=0.0) -> ("output"=w2261:dbl)  [unwired: 6 in, 1 out]
        n1021 = Greater Or Equal?(x=w2280, y=20) -> (x >= y?=w2278:bool)
        n1022 = Negate(x=w2261) -> (-x=w2260:dbl)
        n1023 = Wait (ms)(milliseconds to wait=u32 20) -> ()  [unwired: 1 out]
        n1024 = call-poly <vilib>:"CTRE_Phoenix_MotorController_Get_Enhanced.vi"("PhoenixMotorControlDevRef"=w2255, "error in"=w2254) -> ("Quadrature Position"=w2276:i32)  [unwired: 10 in, 3 out]
        n1025 = To Double Precision Float(number=w2276) -> (double precision float=w2275:dbl)
        n1026 = feedback #18() -> (w2259:dbl)  [unwired: 1 in]
        n1027 = call-poly <vilib>:"WPI_RobotDriveArcadeDrive.vi"("error in (no error)"=w2263, "Y axis value"=w2259, "X axis value"=w2260, "RobotDriveDevRef"=w2264) -> ()  [unwired: 5 in, 3 out]
        n1028 = Absolute Value(x=w2275) -> (abs(x)=w2271:dbl)
        n1029 = Greater Or Equal?(x=w2271, y=113500.0 ("upper limit")) -> (x >= y?=w2269:bool)
        n1030 = And(x=w2269, y=w2278) -> (x .and. y?=w2277:bool)
        n1031 = Select(t=0.0, s=w2269, f=-0.6) -> (s? t:f=w2272:dbl)
        n1032 = feedback-in #18(w2272) -> ()
      }
      n1033 = while {
        tunnel: [w2143] -> _
        tunnel: w2081 -> [w2143]
        tunnel: [w2142] -> _
        tunnel: w2080 -> [w2142]
        tunnel: [w2141] -> _
        tunnel: w2079 -> [w2141]
        tunnel: [w2140] -> _
        tunnel: w2078 -> [w2140]
        i -> [w2167]
        stop <- w2144 stop-if-true
        # "Set config to shoot level, Rev, Shoot, and reset"
        n1034 = global read "Robot Global Data.vi" "Pot 1"() -> (w2172:dbl)
        n1035 = call <vilib>:"WPI_MotorControlRefNum Registry Get.vi"("refnum name"="Acquire") -> ("error out"=w2169:errorcluster, "MotorControlDevRef"=w2170:T8)  [unwired: 9 in]
        n1036 = call <vilib>:"WPI_MotorControlRefNum Registry Get.vi"("refnum name"="Dart 1") -> ("error out"=w2176:errorcluster, "MotorControlDevRef"=w2175:T8)  [unwired: 9 in]
        n1037 = Increment(x=w2167) -> (x+1=w2168:i32)
        n1038 = call-poly <vilib>:"PID.vi"("PID gains"=T7 {"proportional gain (Kc)"=1.0, "integral time (Ti, min)"=0.01, "derivative time (Td, min)"=0.0}, "process variable"=w2172, "setpoint"=0.0) -> ("output"=w2177:dbl)  [unwired: 7 in, 1 out]
        n1039 = Greater Or Equal?(x=w2168, y=100) -> (x >= y?=w2159:bool)
        n1040 = call <vilib>:"WPI_MotorControlSetOutput.vi"("error in (no error)"=w2176, "Output"=w2177, "MotorControlDevRef"=w2175) -> ()  [unwired: 6 in, 3 out]
        n1041 = call <vilib>:"WPI_MotorControlSetOutput.vi"("error in (no error)"=w2169, "Output"=-1.0, "MotorControlDevRef"=w2170) -> ()  [unwired: 6 in, 3 out]
        n1042 = Select(t=WPI_SolenoidValue."Forward" ("Value"), s=w2159, f=WPI_SolenoidValue."Off" ("Value")) -> (s? t:f=w2162:T6)
        n1043 = Wait (ms)(milliseconds to wait=u32 20) -> ()  [unwired: 1 out]
        n1044 = call <vilib>:"WPI_SolenoidRefNum Registry Get.vi"("refnum name"="Push") -> ("error out"=w2163:errorcluster, "SolenoidDevRef"=w2164:T16)  [unwired: 9 in]
        n1045 = call-poly <vilib>:"WPI_SolenoidSet.vi"("error in (no error)"=w2163, "Value"=w2162, "SolenoidDevRef"=w2164) -> ("error out"=w2155:errorcluster, "SolenoidDevRef"=w2156:T16)  [unwired: 7 in]
        n1046 = call-poly <vilib>:"WPI_SolenoidGet.vi"("error in (no error)"=w2155, "SolenoidDevRef"=w2156) -> ("Value"=w2154:bool)  [unwired: 7 in, 2 out]
        n1047 = And(x=w2159, y=w2154) -> (x .and. y?=w2145:bool)
        n1048 = Select(t=WPI_SolenoidValue."Reverse" ("Value"), s=w2145, f=WPI_SolenoidValue."Off" ("Value")) -> (s? t:f=w2150:T6)
        n1049 = call <vilib>:"WPI_SolenoidRefNum Registry Get.vi"("refnum name"="Push") -> ("error out"=w2151:errorcluster, "SolenoidDevRef"=w2152:T16)  [unwired: 9 in]
        n1050 = call-poly <vilib>:"WPI_SolenoidSet.vi"("error in (no error)"=w2151, "Value"=w2150, "SolenoidDevRef"=w2152) -> ("error out"=w2146:errorcluster, "SolenoidDevRef"=w2147:T16)  [unwired: 7 in]
        n1051 = call-poly <vilib>:"WPI_SolenoidGet.vi"("error in (no error)"=w2146, "SolenoidDevRef"=w2147) -> ("Value"=w2144:bool)  [unwired: 7 in, 2 out]
      }
    }
    frame "Center Place 2 Switch Left" {
      n1052 = call <vilib>:"WPI_MotorControlRefNum Registry Get.vi"("refnum name"="Left Lead") -> ("error out"=w2404:errorcluster, "MotorControlDevRef"=w2405:T8)  [unwired: 9 in]
      n1053 = call <vilib>:"WPI_MotorControlRefNum Registry Get.vi"("refnum name"="Right Lead") -> ("error out"=w2402:errorcluster, "MotorControlDevRef"=w2403:T8)  [unwired: 9 in]
      n1054 = while {
        tunnel: w2405 -> [w2687]
        tunnel: w2404 -> [w2686]
        tunnel: w2403 -> [w2685]
        tunnel: w2402 -> [w2684]
        tunnel: [w2687] -> w2445
        tunnel: [w2686] -> w2444
        tunnel: [w2685] -> w2443
        tunnel: [w2684] -> w2442
        i -> [w2697]
        stop <- w2696 stop-if-true
        n1055 = Increment(x=w2697) -> (x+1=w2699:i32)
        n1056 = Greater?(x=w2699, y=10) -> (0:w2696:bool)
        n1057 = call <vilib>:"CTRE_PigeonIMU_RefNumRegistryGet.vi"("refnum name"="Pigeon") -> ("PigeonIMUDevRef"=w2694:T13)  [unwired: 9 in, 1 out]
        n1058 = call-poly <vilib>:"CTRE_Phoenix_MotorController_Get_Enhanced.vi"("PhoenixMotorControlDevRef"=w2687, "error in"=w2686) -> ("PhoenixMotorControlDevRef"=w2689:T8)  [unwired: 10 in, 3 out]
        n1059 = call-poly <vilib>:"CTRE_Phoenix_MotorController_Get_Enhanced.vi"("PhoenixMotorControlDevRef"=w2685, "error in"=w2684) -> ("PhoenixMotorControlDevRef"=w2688:T8)  [unwired: 10 in, 3 out]
        n1060 = call "CTRE_Phoenix_MotorControl_SetQuadraturePosition_Enhanced.vi"("New Position"=0, "PhoenixMotorControlDevRef"=w2688) -> ()  [unwired: 8 in, 2 out]
        n1061 = call "CTRE_Phoenix_MotorControl_SetQuadraturePosition_Enhanced.vi"("New Position"=0, "PhoenixMotorControlDevRef"=w2689) -> ()  [unwired: 8 in, 2 out]
        n1062 = Wait (ms)(milliseconds to wait=u32 20) -> ()  [unwired: 1 out]
        n1063 = call <vilib>:"CTRE_PigeonIMU_SetYaw.vi"("Value"=0.0, "PigeonIMUDevRef"=w2694) -> ()  [unwired: 8 in, 2 out]
      }
      n1064 = while {
        tunnel: [w2702] -> w2441
        tunnel: w2445 -> [w2702]
        tunnel: [w2703] -> w2440
        tunnel: w2444 -> [w2703]
        tunnel: [w2710] -> w2439
        tunnel: w2443 -> [w2710]
        tunnel: [w2709] -> w2438
        tunnel: w2442 -> [w2709]
        i -> [w2726]
        stop <- w2722 stop-if-true
        n1065 = global read "Robot Global Data.vi" "YAW"() -> (w2711:dbl)
        n1066 = Wait (ms)(milliseconds to wait=u32 20) -> ()  [unwired: 1 out]
        n1067 = call <vilib>:"WPI_RobotDriveRefNum Registry Get.vi"("refnum name"="RobotDrive") -> ("error out"=w2707:errorcluster, "RobotDriveDevRef"=w2708:T15)  [unwired: 9 in]
        n1068 = Increment(x=w2726) -> (x+1=w2725:i32)
        n1069 = call-poly <vilib>:"PID.vi"("output range"=cluster{"output high":dbl, "output low":dbl} {"output high"=0.4, "output low"=-0.4}, "PID gains"=T7 {"proportional gain (Kc)"=0.11, "integral time (Ti, min)"=0.0, "derivative time (Td, min)"=0.0}, "process variable"=w2711, "setpoint"=0.0) -> ("output"=w2701:dbl)  [unwired: 6 in, 1 out]
        n1070 = Greater Or Equal?(x=w2725, y=100) -> (x >= y?=w2723:bool)
        n1071 = Negate(x=w2701) -> (-x=w2700:dbl)
        n1072 = call-poly <vilib>:"CTRE_Phoenix_MotorController_Get_Enhanced.vi"("PhoenixMotorControlDevRef"=w2702, "error in"=w2703) -> ("Quadrature Position"=w2721:i32)  [unwired: 10 in, 3 out]
        n1073 = To Double Precision Float(number=w2721) -> (double precision float=w2720:dbl)
        n1074 = feedback #19() -> (w2704:dbl)  [unwired: 1 in]
        n1075 = call-poly <vilib>:"WPI_RobotDriveArcadeDrive.vi"("error in (no error)"=w2707, "Y axis value"=w2704, "X axis value"=w2700, "RobotDriveDevRef"=w2708) -> ()  [unwired: 5 in, 3 out]
        n1076 = Absolute Value(x=w2720) -> (abs(x)=w2716:dbl)
        n1077 = Greater Or Equal?(x=w2716, y=115000.0 ("upper limit")) -> (x >= y?=w2705:bool)
        n1078 = And(x=w2705, y=w2723) -> (x .and. y?=w2722:bool)
        n1079 = Select(t=0.0, s=w2705, f=-0.8) -> (s? t:f=w2717:dbl)
        n1080 = feedback-in #19(w2717) -> ()
      }
      n1081 = while {
        tunnel: w2441 -> [w2674]
        tunnel: w2440 -> [w2673]
        tunnel: w2439 -> [w2672]
        tunnel: w2438 -> [w2671]
        tunnel: [w2674] -> w2437
        tunnel: [w2673] -> w2436
        tunnel: [w2672] -> w2435
        tunnel: [w2671] -> w2434
        i -> [w2677]
        stop <- w2675 stop-if-true
        n1082 = global read "Robot Global Data.vi" "YAW"() -> (w2681:dbl)
        n1083 = Increment(x=w2677) -> (x+1=w2679:i32)
        n1084 = call-poly <vilib>:"PID.vi"("output range"=cluster{"output high":dbl, "output low":dbl} {"output high"=0.7, "output low"=-0.7}, "PID gains"=T7 {"proportional gain (Kc)"=0.045, "integral time (Ti, min)"=0.0, "derivative time (Td, min)"=0.0}, "process variable"=w2681, "setpoint"=-90.0) -> ("output"=w2666:dbl)  [unwired: 6 in, 1 out]
        n1085 = call <vilib>:"WPI_RobotDriveRefNum Registry Get.vi"("refnum name"="RobotDrive") -> ("error out"=w2669:errorcluster, "RobotDriveDevRef"=w2670:T15)  [unwired: 9 in]
        n1086 = Greater?(x=w2679, y=200) -> (0:w2675:bool)
        n1087 = Negate(x=w2666) -> (-x=w2665:dbl)
        n1088 = call-poly <vilib>:"WPI_RobotDriveArcadeDrive.vi"("error in (no error)"=w2669, "Y axis value"=0.0, "X axis value"=w2665, "RobotDriveDevRef"=w2670) -> ()  [unwired: 5 in, 3 out]
        n1089 = Wait (ms)(milliseconds to wait=u32 20) -> ()  [unwired: 1 out]
      }
      n1090 = while {
        tunnel: [w2574] -> w2433
        tunnel: w2437 -> [w2574]
        tunnel: [w2573] -> w2432
        tunnel: w2436 -> [w2573]
        tunnel: [w2572] -> w2431
        tunnel: w2435 -> [w2572]
        tunnel: [w2575] -> w2430
        tunnel: w2434 -> [w2575]
        i -> [w2568]
        stop <- w2554 stop-if-true
        # "Set config to shoot level, Rev, Shoot"
        n1091 = global read "Robot Global Data.vi" "Pot 1"() -> (w2576:dbl)
        n1092 = call <vilib>:"WPI_MotorControlRefNum Registry Get.vi"("refnum name"="Acquire") -> ("error out"=w2569:errorcluster, "MotorControlDevRef"=w2570:T8)  [unwired: 9 in]
        n1093 = call <vilib>:"WPI_MotorControlRefNum Registry Get.vi"("refnum name"="Dart 1") -> ("error out"=w2580:errorcluster, "MotorControlDevRef"=w2579:T8)  [unwired: 9 in]
        n1094 = Increment(x=w2568) -> (x+1=w2555:i32)
        n1095 = call-poly <vilib>:"PID.vi"("PID gains"=T7 {"proportional gain (Kc)"=1.0, "integral time (Ti, min)"=0.01, "derivative time (Td, min)"=0.0}, "process variable"=w2576, "setpoint"=0.0) -> ("output"=w2581:dbl)  [unwired: 7 in, 1 out]
        n1096 = Greater Or Equal?(x=w2555, y=100) -> (x >= y?=w2560:bool)
        n1097 = call <vilib>:"WPI_MotorControlSetOutput.vi"("error in (no error)"=w2580, "Output"=w2581, "MotorControlDevRef"=w2579) -> ()  [unwired: 6 in, 3 out]
        n1098 = call <vilib>:"WPI_MotorControlSetOutput.vi"("error in (no error)"=w2569, "Output"=-1.0, "MotorControlDevRef"=w2570) -> ()  [unwired: 6 in, 3 out]
        n1099 = Select(t=WPI_SolenoidValue."Forward" ("Value"), s=w2560, f=WPI_SolenoidValue."Off" ("Value")) -> (s? t:f=w2563:T6)
        n1100 = Wait (ms)(milliseconds to wait=u32 20) -> ()  [unwired: 1 out]
        n1101 = call <vilib>:"WPI_SolenoidRefNum Registry Get.vi"("refnum name"="Push") -> ("error out"=w2564:errorcluster, "SolenoidDevRef"=w2565:T16)  [unwired: 9 in]
        n1102 = call-poly <vilib>:"WPI_SolenoidSet.vi"("error in (no error)"=w2564, "Value"=w2563, "SolenoidDevRef"=w2565) -> ("error out"=w2556:errorcluster, "SolenoidDevRef"=w2557:T16)  [unwired: 7 in]
        n1103 = call-poly <vilib>:"WPI_SolenoidGet.vi"("error in (no error)"=w2556, "SolenoidDevRef"=w2557) -> ("Value"=w2554:bool)  [unwired: 7 in, 2 out]
      }
      n1104 = while {
        tunnel: w2433 -> [w2460]
        tunnel: w2432 -> [w2459]
        tunnel: w2431 -> [w2458]
        tunnel: w2430 -> [w2457]
        tunnel: [w2460] -> w2429
        tunnel: [w2459] -> w2428
        tunnel: [w2458] -> w2427
        tunnel: [w2457] -> w2426
        i -> [w2448]
        stop <- w2447 stop-if-true
        # "Reset"
        n1105 = call <vilib>:"WPI_SolenoidRefNum Registry Get.vi"("refnum name"="Push") -> ("error out"=w2464:errorcluster, "SolenoidDevRef"=w2465:T16)  [unwired: 9 in]
        n1106 = call <vilib>:"WPI_MotorControlRefNum Registry Get.vi"("refnum name"="Dart 1") -> ("error out"=w2455:errorcluster, "MotorControlDevRef"=w2454:T8)  [unwired: 9 in]
        n1107 = Increment(x=w2448) -> (x+1=w2461:i32)
        n1108 = global read "Robot Global Data.vi" "Pot 1"() -> (w2451:dbl)
        n1109 = Greater Or Equal?(x=w2461, y=100) -> (x >= y?=w2447:bool)
        n1110 = call-poly <vilib>:"PID.vi"("PID gains"=T7 {"proportional gain (Kc)"=1.0, "integral time (Ti, min)"=0.01, "derivative time (Td, min)"=0.0}, "process variable"=w2451, "setpoint"=0.0) -> ("output"=w2456:dbl)  [unwired: 7 in, 1 out]
        n1111 = call <vilib>:"WPI_MotorControlSetOutput.vi"("error in (no error)"=w2455, "Output"=w2456, "MotorControlDevRef"=w2454) -> ()  [unwired: 6 in, 3 out]
        n1112 = call-poly <vilib>:"WPI_SolenoidSet.vi"("error in (no error)"=w2464, "Value"=WPI_SolenoidValue."Reverse", "SolenoidDevRef"=w2465) -> ("error out"=w2462:errorcluster, "SolenoidDevRef"=w2463:T16)  [unwired: 7 in]
        n1113 = call-poly <vilib>:"WPI_SolenoidGet.vi"("error in (no error)"=w2462, "SolenoidDevRef"=w2463) -> ()  [unwired: 7 in, 3 out]
      }
      n1114 = while {
        tunnel: [w2645] -> w2425
        tunnel: w2429 -> [w2645]
        tunnel: [w2644] -> w2424
        tunnel: w2428 -> [w2644]
        tunnel: [w2643] -> w2423
        tunnel: w2427 -> [w2643]
        tunnel: [w2642] -> w2422
        tunnel: w2426 -> [w2642]
        i -> [w2658]
        stop <- w2656 stop-if-true
        n1115 = global read "Robot Global Data.vi" "YAW"() -> (w2662:dbl)
        n1116 = Increment(x=w2658) -> (x+1=w2660:i32)
        n1117 = call-poly <vilib>:"PID.vi"("output range"=cluster{"output high":dbl, "output low":dbl} {"output high"=0.6, "output low"=-0.6}, "PID gains"=T7 {"proportional gain (Kc)"=0.055, "integral time (Ti, min)"=0.0, "derivative time (Td, min)"=0.0}, "process variable"=w2662, "setpoint"=-25.0) -> ("output"=w2652:dbl)  [unwired: 6 in, 1 out]
        n1118 = call <vilib>:"WPI_RobotDriveRefNum Registry Get.vi"("refnum name"="RobotDrive") -> ("error out"=w2653:errorcluster, "RobotDriveDevRef"=w2654:T15)  [unwired: 9 in]
        n1119 = Negate(x=w2652) -> (-x=w2651:dbl)
        n1120 = Greater?(x=w2660, y=180) -> (0:w2656:bool)
        n1121 = call-poly <vilib>:"WPI_RobotDriveArcadeDrive.vi"("error in (no error)"=w2653, "Y axis value"=0.0, "X axis value"=w2651, "RobotDriveDevRef"=w2654) -> ()  [unwired: 5 in, 3 out]
        n1122 = Wait (ms)(milliseconds to wait=u32 20) -> ()  [unwired: 1 out]
        n1123 = call-poly <vilib>:"CTRE_Phoenix_MotorController_Get_Enhanced.vi"("PhoenixMotorControlDevRef"=w2645, "error in"=w2644) -> ("PhoenixMotorControlDevRef"=w2647:T8)  [unwired: 8 in, 5 out]
        n1124 = call-poly <vilib>:"CTRE_Phoenix_MotorController_Get_Enhanced.vi"("PhoenixMotorControlDevRef"=w2643, "error in"=w2642) -> ("PhoenixMotorControlDevRef"=w2646:T8)  [unwired: 8 in, 5 out]
        n1125 = call "CTRE_Phoenix_MotorControl_SetQuadraturePosition_Enhanced.vi"("New Position"=0, "PhoenixMotorControlDevRef"=w2646) -> ()  [unwired: 8 in, 2 out]
        n1126 = call "CTRE_Phoenix_MotorControl_SetQuadraturePosition_Enhanced.vi"("New Position"=0, "PhoenixMotorControlDevRef"=w2647) -> ()  [unwired: 8 in, 2 out]
      }
      n1127 = while {
        tunnel: [w2615] -> w2421
        tunnel: w2425 -> [w2615]
        tunnel: [w2614] -> w2420
        tunnel: w2424 -> [w2614]
        tunnel: [w2613] -> w2419
        tunnel: w2423 -> [w2613]
        tunnel: [w2612] -> w2418
        tunnel: w2422 -> [w2612]
        i -> [w2640]
        stop <- w2636 stop-if-true
        # "Drives towards cube, uses pixy cam's \"x\" value to stay on center"
        n1128 = Increment(x=w2640) -> (x+1=w2639:i32)
        n1129 = Greater Or Equal?(x=w2639, y=100) -> (x >= y?=w2637:bool)
        n1130 = call <vilib>:"WPI_DigitalInputRefNum Registry Get.vi"("refnum name"="Color Mark") -> ("DigitalInputDevRef"=w2626:T18)  [unwired: 9 in, 1 out]
        n1131 = call <vilib>:"WPI_MotorControlRefNum Registry Get.vi"("refnum name"="Acquire") -> ("error out"=w2623:errorcluster, "MotorControlDevRef"=w2624:T8)  [unwired: 9 in]
        n1132 = call <vilib>:"WPI_DigitalInputGetValue.vi"("DigitalInputDevRef"=w2626) -> ("Value"=w2616:bool)  [unwired: 8 in, 2 out]
        n1133 = And(x=w2616, y=w2637) -> (x .and. y?=w2636:bool)
        n1134 = Wait (ms)(milliseconds to wait=u32 20) -> ()  [unwired: 1 out]
        n1135 = Select(t=0.0, s=w2616, f=0.6) -> (s? t:f=w2617:dbl)
        n1136 = Select(t=0.0, s=w2616, f=0.6) -> (s? t:f=w2620:dbl)
        n1137 = call <vilib>:"WPI_MotorControlSetOutput.vi"("error in (no error)"=w2623, "Output"=w2617, "MotorControlDevRef"=w2624) -> ()  [unwired: 6 in, 3 out]
        n1138 = call "PIXY VI.vi"() -> ("X"=w2627:dbl)  [unwired: 14 in, 5 out]
        n1139 = call <vilib>:"WPI_RobotDriveRefNum Registry Get.vi"("refnum name"="RobotDrive") -> ("error out"=w2632:errorcluster, "RobotDriveDevRef"=w2633:T15)  [unwired: 9 in]
        n1140 = call-poly <vilib>:"PID.vi"("output range"=cluster{"output high":dbl, "output low":dbl} {"output high"=0.4, "output low"=-0.4}, "PID gains"=T7 {"proportional gain (Kc)"=0.11, "integral time (Ti, min)"=0.0, "derivative time (Td, min)"=0.0}, "process variable"=w2627, "setpoint"=0.0) -> ("output"=w2630:dbl)  [unwired: 6 in, 1 out]
        n1141 = Negate(x=w2630) -> (-x=w2629:dbl)
        n1142 = call-poly <vilib>:"WPI_RobotDriveArcadeDrive.vi"("error in (no error)"=w2632, "Y axis value"=w2620, "X axis value"=w2629, "RobotDriveDevRef"=w2633) -> ()  [unwired: 5 in, 3 out]
      }
      n1143 = while {
        tunnel: [w2526] -> w2417
        tunnel: w2421 -> [w2526]
        tunnel: [w2525] -> w2416
        tunnel: w2420 -> [w2525]
        tunnel: [w2528] -> w2415
        tunnel: w2419 -> [w2528]
        tunnel: [w2527] -> w2414
        tunnel: w2418 -> [w2527]
        i -> [w2551]
        stop <- w2547 stop-if-true
        n1144 = global read "Robot Global Data.vi" "YAW"() -> (w2536:dbl)
        n1145 = call <vilib>:"WPI_RobotDriveRefNum Registry Get.vi"("refnum name"="RobotDrive") -> ("error out"=w2534:errorcluster, "RobotDriveDevRef"=w2535:T15)  [unwired: 9 in]
        n1146 = Wait (ms)(milliseconds to wait=u32 20) -> ()  [unwired: 1 out]
        n1147 = Increment(x=w2551) -> (x+1=w2550:i32)
        n1148 = call-poly <vilib>:"PID.vi"("output range"=cluster{"output high":dbl, "output low":dbl} {"output high"=0.4, "output low"=-0.4}, "PID gains"=T7 {"proportional gain (Kc)"=0.11, "integral time (Ti, min)"=0.0, "derivative time (Td, min)"=0.0}, "process variable"=w2536, "setpoint"=-25.0) -> ("output"=w2530:dbl)  [unwired: 6 in, 1 out]
        n1149 = Greater Or Equal?(x=w2550, y=100) -> (x >= y?=w2548:bool)
        n1150 = Negate(x=w2530) -> (-x=w2529:dbl)
        n1151 = call-poly <vilib>:"CTRE_Phoenix_MotorController_Get_Enhanced.vi"("PhoenixMotorControlDevRef"=w2526, "error in"=w2525) -> ("Quadrature Position"=w2546:i32)  [unwired: 10 in, 3 out]
        n1152 = To Double Precision Float(number=w2546) -> (double precision float=w2545:dbl)
        n1153 = feedback #20() -> (w2531:dbl)  [unwired: 1 in]
        n1154 = call-poly <vilib>:"WPI_RobotDriveArcadeDrive.vi"("error in (no error)"=w2534, "Y axis value"=w2531, "X axis value"=w2529, "RobotDriveDevRef"=w2535) -> ()  [unwired: 5 in, 3 out]
        n1155 = Absolute Value(x=w2545) -> (abs(x)=w2541:dbl)
        n1156 = Greater Or Equal?(x=w2541, y=115000.0 ("upper limit")) -> (x >= y?=w2532:bool)
        n1157 = And(x=w2532, y=w2548) -> (x .and. y?=w2547:bool)
        n1158 = Select(t=0.0, s=w2532, f=-0.6) -> (s? t:f=w2542:dbl)
        n1159 = feedback-in #20(w2542) -> ()
      }
      n1160 = while {
        tunnel: w2417 -> [w2509]
        tunnel: w2416 -> [w2508]
        tunnel: w2415 -> [w2507]
        tunnel: w2414 -> [w2506]
        tunnel: [w2509] -> w2413
        tunnel: [w2508] -> w2412
        tunnel: [w2507] -> w2411
        tunnel: [w2506] -> w2410
        i -> [w2518]
        stop <- w2516 stop-if-true
        n1161 = global read "Robot Global Data.vi" "YAW"() -> (w2522:dbl)
        n1162 = Increment(x=w2518) -> (x+1=w2520:i32)
        n1163 = call-poly <vilib>:"PID.vi"("output range"=cluster{"output high":dbl, "output low":dbl} {"output high"=0.7, "output low"=-0.7}, "PID gains"=T7 {"proportional gain (Kc)"=0.045, "integral time (Ti, min)"=0.0, "derivative time (Td, min)"=0.0}, "process variable"=w2522, "setpoint"=-90.0) -> ("output"=w2511:dbl)  [unwired: 6 in, 1 out]
        n1164 = call <vilib>:"WPI_RobotDriveRefNum Registry Get.vi"("refnum name"="RobotDrive") -> ("error out"=w2514:errorcluster, "RobotDriveDevRef"=w2515:T15)  [unwired: 9 in]
        n1165 = Greater?(x=w2520, y=200) -> (0:w2516:bool)
        n1166 = Negate(x=w2511) -> (-x=w2510:dbl)
        n1167 = call-poly <vilib>:"WPI_RobotDriveArcadeDrive.vi"("error in (no error)"=w2514, "Y axis value"=0.0, "X axis value"=w2510, "RobotDriveDevRef"=w2515) -> ()  [unwired: 5 in, 3 out]
        n1168 = Wait (ms)(milliseconds to wait=u32 20) -> ()  [unwired: 1 out]
      }
      n1169 = while {
        tunnel: [w2583] -> w2409
        tunnel: w2413 -> [w2583]
        tunnel: w2412 -> [w2582]
        tunnel: [w2582] -> w2408
        tunnel: [w2585] -> w2407
        tunnel: w2411 -> [w2585]
        tunnel: [w2584] -> w2406
        tunnel: w2410 -> [w2584]
        i -> [w2609]
        stop <- w2605 stop-if-true
        n1170 = global read "Robot Global Data.vi" "YAW"() -> (w2593:dbl)
        n1171 = call <vilib>:"WPI_RobotDriveRefNum Registry Get.vi"("refnum name"="RobotDrive") -> ("error out"=w2591:errorcluster, "RobotDriveDevRef"=w2592:T15)  [unwired: 9 in]
        n1172 = Increment(x=w2609) -> (x+1=w2608:i32)
        n1173 = Wait (ms)(milliseconds to wait=u32 20) -> ()  [unwired: 1 out]
        n1174 = call-poly <vilib>:"PID.vi"("output range"=cluster{"output high":dbl, "output low":dbl} {"output high"=0.4, "output low"=-0.4}, "PID gains"=T7 {"proportional gain (Kc)"=0.11, "integral time (Ti, min)"=0.0, "derivative time (Td, min)"=0.0}, "process variable"=w2593, "setpoint"=0.0) -> ("output"=w2589:dbl)  [unwired: 6 in, 1 out]
        n1175 = Greater Or Equal?(x=w2608, y=20) -> (x >= y?=w2606:bool)
        n1176 = Negate(x=w2589) -> (-x=w2588:dbl)
        n1177 = Wait (ms)(milliseconds to wait=u32 20) -> ()  [unwired: 1 out]
        n1178 = call-poly <vilib>:"CTRE_Phoenix_MotorController_Get_Enhanced.vi"("PhoenixMotorControlDevRef"=w2583, "error in"=w2582) -> ("Quadrature Position"=w2604:i32)  [unwired: 10 in, 3 out]
        n1179 = To Double Precision Float(number=w2604) -> (double precision float=w2603:dbl)
        n1180 = feedback #21() -> (w2587:dbl)  [unwired: 1 in]
        n1181 = call-poly <vilib>:"WPI_RobotDriveArcadeDrive.vi"("error in (no error)"=w2591, "Y axis value"=w2587, "X axis value"=w2588, "RobotDriveDevRef"=w2592) -> ()  [unwired: 5 in, 3 out]
        n1182 = Absolute Value(x=w2603) -> (abs(x)=w2599:dbl)
        n1183 = Greater Or Equal?(x=w2599, y=113500.0 ("upper limit")) -> (x >= y?=w2597:bool)
        n1184 = And(x=w2597, y=w2606) -> (x .and. y?=w2605:bool)
        n1185 = Select(t=0.0, s=w2597, f=-0.6) -> (s? t:f=w2600:dbl)
        n1186 = feedback-in #21(w2600) -> ()
      }
      n1187 = while {
        tunnel: [w2471] -> _
        tunnel: w2409 -> [w2471]
        tunnel: [w2470] -> _
        tunnel: w2408 -> [w2470]
        tunnel: [w2469] -> _
        tunnel: w2407 -> [w2469]
        tunnel: [w2468] -> _
        tunnel: w2406 -> [w2468]
        i -> [w2495]
        stop <- w2472 stop-if-true
        # "Set config to shoot level, Rev, Shoot, and reset"
        n1188 = global read "Robot Global Data.vi" "Pot 1"() -> (w2500:dbl)
        n1189 = call <vilib>:"WPI_MotorControlRefNum Registry Get.vi"("refnum name"="Acquire") -> ("error out"=w2497:errorcluster, "MotorControlDevRef"=w2498:T8)  [unwired: 9 in]
        n1190 = call <vilib>:"WPI_MotorControlRefNum Registry Get.vi"("refnum name"="Dart 1") -> ("error out"=w2504:errorcluster, "MotorControlDevRef"=w2503:T8)  [unwired: 9 in]
        n1191 = Increment(x=w2495) -> (x+1=w2496:i32)
        n1192 = call-poly <vilib>:"PID.vi"("PID gains"=T7 {"proportional gain (Kc)"=1.0, "integral time (Ti, min)"=0.01, "derivative time (Td, min)"=0.0}, "process variable"=w2500, "setpoint"=0.0) -> ("output"=w2505:dbl)  [unwired: 7 in, 1 out]
        n1193 = Greater Or Equal?(x=w2496, y=100) -> (x >= y?=w2487:bool)
        n1194 = call <vilib>:"WPI_MotorControlSetOutput.vi"("error in (no error)"=w2504, "Output"=w2505, "MotorControlDevRef"=w2503) -> ()  [unwired: 6 in, 3 out]
        n1195 = call <vilib>:"WPI_MotorControlSetOutput.vi"("error in (no error)"=w2497, "Output"=-1.0, "MotorControlDevRef"=w2498) -> ()  [unwired: 6 in, 3 out]
        n1196 = Select(t=WPI_SolenoidValue."Forward" ("Value"), s=w2487, f=WPI_SolenoidValue."Off" ("Value")) -> (s? t:f=w2490:T6)
        n1197 = Wait (ms)(milliseconds to wait=u32 20) -> ()  [unwired: 1 out]
        n1198 = call <vilib>:"WPI_SolenoidRefNum Registry Get.vi"("refnum name"="Push") -> ("error out"=w2491:errorcluster, "SolenoidDevRef"=w2492:T16)  [unwired: 9 in]
        n1199 = call-poly <vilib>:"WPI_SolenoidSet.vi"("error in (no error)"=w2491, "Value"=w2490, "SolenoidDevRef"=w2492) -> ("error out"=w2483:errorcluster, "SolenoidDevRef"=w2484:T16)  [unwired: 7 in]
        n1200 = call-poly <vilib>:"WPI_SolenoidGet.vi"("error in (no error)"=w2483, "SolenoidDevRef"=w2484) -> ("Value"=w2482:bool)  [unwired: 7 in, 2 out]
        n1201 = And(x=w2487, y=w2482) -> (x .and. y?=w2473:bool)
        n1202 = Select(t=WPI_SolenoidValue."Reverse" ("Value"), s=w2473, f=WPI_SolenoidValue."Off" ("Value")) -> (s? t:f=w2478:T6)
        n1203 = call <vilib>:"WPI_SolenoidRefNum Registry Get.vi"("refnum name"="Push") -> ("error out"=w2479:errorcluster, "SolenoidDevRef"=w2480:T16)  [unwired: 9 in]
        n1204 = call-poly <vilib>:"WPI_SolenoidSet.vi"("error in (no error)"=w2479, "Value"=w2478, "SolenoidDevRef"=w2480) -> ("error out"=w2474:errorcluster, "SolenoidDevRef"=w2475:T16)  [unwired: 7 in]
        n1205 = call-poly <vilib>:"WPI_SolenoidGet.vi"("error in (no error)"=w2474, "SolenoidDevRef"=w2475) -> ("Value"=w2472:bool)  [unwired: 7 in, 2 out]
      }
    }
    frame "Center Place 1 Switch Left" {
      n1206 = call <vilib>:"WPI_MotorControlRefNum Registry Get.vi"("refnum name"="Left Lead") -> ("error out"=w2732:errorcluster, "MotorControlDevRef"=w2733:T8)  [unwired: 9 in]
      n1207 = call <vilib>:"WPI_MotorControlRefNum Registry Get.vi"("refnum name"="Right Lead") -> ("error out"=w2730:errorcluster, "MotorControlDevRef"=w2731:T8)  [unwired: 9 in]
      n1208 = while {
        tunnel: w2733 -> [w3015]
        tunnel: w2732 -> [w3014]
        tunnel: w2731 -> [w3013]
        tunnel: w2730 -> [w3012]
        tunnel: [w3015] -> w2773
        tunnel: [w3014] -> w2772
        tunnel: [w3013] -> w2771
        tunnel: [w3012] -> w2770
        i -> [w3025]
        stop <- w3024 stop-if-true
        n1209 = Increment(x=w3025) -> (x+1=w3027:i32)
        n1210 = Greater?(x=w3027, y=10) -> (0:w3024:bool)
        n1211 = call <vilib>:"CTRE_PigeonIMU_RefNumRegistryGet.vi"("refnum name"="Pigeon") -> ("PigeonIMUDevRef"=w3022:T13)  [unwired: 9 in, 1 out]
        n1212 = call-poly <vilib>:"CTRE_Phoenix_MotorController_Get_Enhanced.vi"("PhoenixMotorControlDevRef"=w3015, "error in"=w3014) -> ("PhoenixMotorControlDevRef"=w3017:T8)  [unwired: 10 in, 3 out]
        n1213 = call-poly <vilib>:"CTRE_Phoenix_MotorController_Get_Enhanced.vi"("PhoenixMotorControlDevRef"=w3013, "error in"=w3012) -> ("PhoenixMotorControlDevRef"=w3016:T8)  [unwired: 10 in, 3 out]
        n1214 = call "CTRE_Phoenix_MotorControl_SetQuadraturePosition_Enhanced.vi"("New Position"=0, "PhoenixMotorControlDevRef"=w3016) -> ()  [unwired: 8 in, 2 out]
        n1215 = call "CTRE_Phoenix_MotorControl_SetQuadraturePosition_Enhanced.vi"("New Position"=0, "PhoenixMotorControlDevRef"=w3017) -> ()  [unwired: 8 in, 2 out]
        n1216 = Wait (ms)(milliseconds to wait=u32 20) -> ()  [unwired: 1 out]
        n1217 = call <vilib>:"CTRE_PigeonIMU_SetYaw.vi"("Value"=0.0, "PigeonIMUDevRef"=w3022) -> ()  [unwired: 8 in, 2 out]
      }
      n1218 = while {
        tunnel: [w3030] -> w2769
        tunnel: w2773 -> [w3030]
        tunnel: [w3031] -> w2768
        tunnel: w2772 -> [w3031]
        tunnel: [w3038] -> w2767
        tunnel: w2771 -> [w3038]
        tunnel: [w3037] -> w2766
        tunnel: w2770 -> [w3037]
        i -> [w3054]
        stop <- w3050 stop-if-true
        n1219 = global read "Robot Global Data.vi" "YAW"() -> (w3039:dbl)
        n1220 = Wait (ms)(milliseconds to wait=u32 20) -> ()  [unwired: 1 out]
        n1221 = call <vilib>:"WPI_RobotDriveRefNum Registry Get.vi"("refnum name"="RobotDrive") -> ("error out"=w3035:errorcluster, "RobotDriveDevRef"=w3036:T15)  [unwired: 9 in]
        n1222 = Increment(x=w3054) -> (x+1=w3053:i32)
        n1223 = call-poly <vilib>:"PID.vi"("output range"=cluster{"output high":dbl, "output low":dbl} {"output high"=0.4, "output low"=-0.4}, "PID gains"=T7 {"proportional gain (Kc)"=0.11, "integral time (Ti, min)"=0.0, "derivative time (Td, min)"=0.0}, "process variable"=w3039, "setpoint"=0.0) -> ("output"=w3029:dbl)  [unwired: 6 in, 1 out]
        n1224 = Greater Or Equal?(x=w3053, y=100) -> (x >= y?=w3051:bool)
        n1225 = Negate(x=w3029) -> (-x=w3028:dbl)
        n1226 = call-poly <vilib>:"CTRE_Phoenix_MotorController_Get_Enhanced.vi"("PhoenixMotorControlDevRef"=w3030, "error in"=w3031) -> ("Quadrature Position"=w3049:i32)  [unwired: 10 in, 3 out]
        n1227 = To Double Precision Float(number=w3049) -> (double precision float=w3048:dbl)
        n1228 = feedback #22() -> (w3032:dbl)  [unwired: 1 in]
        n1229 = call-poly <vilib>:"WPI_RobotDriveArcadeDrive.vi"("error in (no error)"=w3035, "Y axis value"=w3032, "X axis value"=w3028, "RobotDriveDevRef"=w3036) -> ()  [unwired: 5 in, 3 out]
        n1230 = Absolute Value(x=w3048) -> (abs(x)=w3044:dbl)
        n1231 = Greater Or Equal?(x=w3044, y=115000.0 ("upper limit")) -> (x >= y?=w3033:bool)
        n1232 = And(x=w3033, y=w3051) -> (x .and. y?=w3050:bool)
        n1233 = Select(t=0.0, s=w3033, f=-0.8) -> (s? t:f=w3045:dbl)
        n1234 = feedback-in #22(w3045) -> ()
      }
      n1235 = while {
        tunnel: w2769 -> [w3002]
        tunnel: w2768 -> [w3001]
        tunnel: w2767 -> [w3000]
        tunnel: w2766 -> [w2999]
        tunnel: [w3002] -> w2765
        tunnel: [w3001] -> w2764
        tunnel: [w3000] -> w2763
        tunnel: [w2999] -> w2762
        i -> [w3005]
        stop <- w3003 stop-if-true
        n1236 = global read "Robot Global Data.vi" "YAW"() -> (w3009:dbl)
        n1237 = Increment(x=w3005) -> (x+1=w3007:i32)
        n1238 = call-poly <vilib>:"PID.vi"("output range"=cluster{"output high":dbl, "output low":dbl} {"output high"=0.7, "output low"=-0.7}, "PID gains"=T7 {"proportional gain (Kc)"=0.045, "integral time (Ti, min)"=0.0, "derivative time (Td, min)"=0.0}, "process variable"=w3009, "setpoint"=-90.0) -> ("output"=w2994:dbl)  [unwired: 6 in, 1 out]
        n1239 = call <vilib>:"WPI_RobotDriveRefNum Registry Get.vi"("refnum name"="RobotDrive") -> ("error out"=w2997:errorcluster, "RobotDriveDevRef"=w2998:T15)  [unwired: 9 in]
        n1240 = Greater?(x=w3007, y=200) -> (0:w3003:bool)
        n1241 = Negate(x=w2994) -> (-x=w2993:dbl)
        n1242 = call-poly <vilib>:"WPI_RobotDriveArcadeDrive.vi"("error in (no error)"=w2997, "Y axis value"=0.0, "X axis value"=w2993, "RobotDriveDevRef"=w2998) -> ()  [unwired: 5 in, 3 out]
        n1243 = Wait (ms)(milliseconds to wait=u32 20) -> ()  [unwired: 1 out]
      }
      n1244 = while {
        tunnel: [w2902] -> w2761
        tunnel: w2765 -> [w2902]
        tunnel: [w2901] -> w2760
        tunnel: w2764 -> [w2901]
        tunnel: [w2900] -> w2759
        tunnel: w2763 -> [w2900]
        tunnel: [w2903] -> w2758
        tunnel: w2762 -> [w2903]
        i -> [w2896]
        stop <- w2882 stop-if-true
        # "Set config to shoot level, Rev, Shoot"
        n1245 = global read "Robot Global Data.vi" "Pot 1"() -> (w2904:dbl)
        n1246 = call <vilib>:"WPI_MotorControlRefNum Registry Get.vi"("refnum name"="Acquire") -> ("error out"=w2897:errorcluster, "MotorControlDevRef"=w2898:T8)  [unwired: 9 in]
        n1247 = call <vilib>:"WPI_MotorControlRefNum Registry Get.vi"("refnum name"="Dart 1") -> ("error out"=w2908:errorcluster, "MotorControlDevRef"=w2907:T8)  [unwired: 9 in]
        n1248 = Increment(x=w2896) -> (x+1=w2883:i32)
        n1249 = call-poly <vilib>:"PID.vi"("PID gains"=T7 {"proportional gain (Kc)"=1.0, "integral time (Ti, min)"=0.01, "derivative time (Td, min)"=0.0}, "process variable"=w2904, "setpoint"=0.0) -> ("output"=w2909:dbl)  [unwired: 7 in, 1 out]
        n1250 = Greater Or Equal?(x=w2883, y=100) -> (x >= y?=w2888:bool)
        n1251 = call <vilib>:"WPI_MotorControlSetOutput.vi"("error in (no error)"=w2908, "Output"=w2909, "MotorControlDevRef"=w2907) -> ()  [unwired: 6 in, 3 out]
        n1252 = call <vilib>:"WPI_MotorControlSetOutput.vi"("error in (no error)"=w2897, "Output"=-1.0, "MotorControlDevRef"=w2898) -> ()  [unwired: 6 in, 3 out]
        n1253 = Select(t=WPI_SolenoidValue."Forward" ("Value"), s=w2888, f=WPI_SolenoidValue."Off" ("Value")) -> (s? t:f=w2891:T6)
        n1254 = Wait (ms)(milliseconds to wait=u32 20) -> ()  [unwired: 1 out]
        n1255 = call <vilib>:"WPI_SolenoidRefNum Registry Get.vi"("refnum name"="Push") -> ("error out"=w2892:errorcluster, "SolenoidDevRef"=w2893:T16)  [unwired: 9 in]
        n1256 = call-poly <vilib>:"WPI_SolenoidSet.vi"("error in (no error)"=w2892, "Value"=w2891, "SolenoidDevRef"=w2893) -> ("error out"=w2884:errorcluster, "SolenoidDevRef"=w2885:T16)  [unwired: 7 in]
        n1257 = call-poly <vilib>:"WPI_SolenoidGet.vi"("error in (no error)"=w2884, "SolenoidDevRef"=w2885) -> ("Value"=w2882:bool)  [unwired: 7 in, 2 out]
      }
      n1258 = while {
        tunnel: w2761 -> [w2788]
        tunnel: w2760 -> [w2787]
        tunnel: w2759 -> [w2786]
        tunnel: w2758 -> [w2785]
        tunnel: [w2788] -> w2757
        tunnel: [w2787] -> w2756
        tunnel: [w2786] -> w2755
        tunnel: [w2785] -> w2754
        i -> [w2776]
        stop <- w2775 stop-if-true
        # "Reset"
        n1259 = call <vilib>:"WPI_SolenoidRefNum Registry Get.vi"("refnum name"="Push") -> ("error out"=w2792:errorcluster, "SolenoidDevRef"=w2793:T16)  [unwired: 9 in]
        n1260 = call <vilib>:"WPI_MotorControlRefNum Registry Get.vi"("refnum name"="Dart 1") -> ("error out"=w2783:errorcluster, "MotorControlDevRef"=w2782:T8)  [unwired: 9 in]
        n1261 = Increment(x=w2776) -> (x+1=w2789:i32)
        n1262 = global read "Robot Global Data.vi" "Pot 1"() -> (w2779:dbl)
        n1263 = Greater Or Equal?(x=w2789, y=100) -> (x >= y?=w2775:bool)
        n1264 = call-poly <vilib>:"PID.vi"("PID gains"=T7 {"proportional gain (Kc)"=1.0, "integral time (Ti, min)"=0.01, "derivative time (Td, min)"=0.0}, "process variable"=w2779, "setpoint"=0.0) -> ("output"=w2784:dbl)  [unwired: 7 in, 1 out]
        n1265 = call <vilib>:"WPI_MotorControlSetOutput.vi"("error in (no error)"=w2783, "Output"=w2784, "MotorControlDevRef"=w2782) -> ()  [unwired: 6 in, 3 out]
        n1266 = call-poly <vilib>:"WPI_SolenoidSet.vi"("error in (no error)"=w2792, "Value"=WPI_SolenoidValue."Reverse", "SolenoidDevRef"=w2793) -> ("error out"=w2790:errorcluster, "SolenoidDevRef"=w2791:T16)  [unwired: 7 in]
        n1267 = call-poly <vilib>:"WPI_SolenoidGet.vi"("error in (no error)"=w2790, "SolenoidDevRef"=w2791) -> ()  [unwired: 7 in, 3 out]
      }
      n1268 = while {
        tunnel: [w2973] -> w2753
        tunnel: w2757 -> [w2973]
        tunnel: [w2972] -> w2752
        tunnel: w2756 -> [w2972]
        tunnel: [w2971] -> w2751
        tunnel: w2755 -> [w2971]
        tunnel: [w2970] -> w2750
        tunnel: w2754 -> [w2970]
        i -> [w2986]
        stop <- w2984 stop-if-true
        n1269 = global read "Robot Global Data.vi" "YAW"() -> (w2990:dbl)
        n1270 = Increment(x=w2986) -> (x+1=w2988:i32)
        n1271 = call-poly <vilib>:"PID.vi"("output range"=cluster{"output high":dbl, "output low":dbl} {"output high"=0.6, "output low"=-0.6}, "PID gains"=T7 {"proportional gain (Kc)"=0.055, "integral time (Ti, min)"=0.0, "derivative time (Td, min)"=0.0}, "process variable"=w2990, "setpoint"=-25.0) -> ("output"=w2980:dbl)  [unwired: 6 in, 1 out]
        n1272 = call <vilib>:"WPI_RobotDriveRefNum Registry Get.vi"("refnum name"="RobotDrive") -> ("error out"=w2981:errorcluster, "RobotDriveDevRef"=w2982:T15)  [unwired: 9 in]
        n1273 = Negate(x=w2980) -> (-x=w2979:dbl)
        n1274 = Greater?(x=w2988, y=180) -> (0:w2984:bool)
        n1275 = call-poly <vilib>:"WPI_RobotDriveArcadeDrive.vi"("error in (no error)"=w2981, "Y axis value"=0.0, "X axis value"=w2979, "RobotDriveDevRef"=w2982) -> ()  [unwired: 5 in, 3 out]
        n1276 = Wait (ms)(milliseconds to wait=u32 20) -> ()  [unwired: 1 out]
        n1277 = call-poly <vilib>:"CTRE_Phoenix_MotorController_Get_Enhanced.vi"("PhoenixMotorControlDevRef"=w2973, "error in"=w2972) -> ("PhoenixMotorControlDevRef"=w2975:T8)  [unwired: 8 in, 5 out]
        n1278 = call-poly <vilib>:"CTRE_Phoenix_MotorController_Get_Enhanced.vi"("PhoenixMotorControlDevRef"=w2971, "error in"=w2970) -> ("PhoenixMotorControlDevRef"=w2974:T8)  [unwired: 8 in, 5 out]
        n1279 = call "CTRE_Phoenix_MotorControl_SetQuadraturePosition_Enhanced.vi"("New Position"=0, "PhoenixMotorControlDevRef"=w2974) -> ()  [unwired: 8 in, 2 out]
        n1280 = call "CTRE_Phoenix_MotorControl_SetQuadraturePosition_Enhanced.vi"("New Position"=0, "PhoenixMotorControlDevRef"=w2975) -> ()  [unwired: 8 in, 2 out]
      }
      n1281 = while {
        tunnel: [w2943] -> w2749
        tunnel: w2753 -> [w2943]
        tunnel: [w2942] -> w2748
        tunnel: w2752 -> [w2942]
        tunnel: [w2941] -> w2747
        tunnel: w2751 -> [w2941]
        tunnel: [w2940] -> w2746
        tunnel: w2750 -> [w2940]
        i -> [w2968]
        stop <- w2964 stop-if-true
        # "Drives towards cube, uses pixy cam's \"x\" value to stay on center"
        n1282 = Increment(x=w2968) -> (x+1=w2967:i32)
        n1283 = Greater Or Equal?(x=w2967, y=100) -> (x >= y?=w2965:bool)
        n1284 = call <vilib>:"WPI_DigitalInputRefNum Registry Get.vi"("refnum name"="Color Mark") -> ("DigitalInputDevRef"=w2954:T18)  [unwired: 9 in, 1 out]
        n1285 = call <vilib>:"WPI_MotorControlRefNum Registry Get.vi"("refnum name"="Acquire") -> ("error out"=w2951:errorcluster, "MotorControlDevRef"=w2952:T8)  [unwired: 9 in]
        n1286 = call <vilib>:"WPI_DigitalInputGetValue.vi"("DigitalInputDevRef"=w2954) -> ("Value"=w2944:bool)  [unwired: 8 in, 2 out]
        n1287 = And(x=w2944, y=w2965) -> (x .and. y?=w2964:bool)
        n1288 = Wait (ms)(milliseconds to wait=u32 20) -> ()  [unwired: 1 out]
        n1289 = Select(t=0.0, s=w2944, f=0.6) -> (s? t:f=w2945:dbl)
        n1290 = Select(t=0.0, s=w2944, f=0.6) -> (s? t:f=w2948:dbl)
        n1291 = call <vilib>:"WPI_MotorControlSetOutput.vi"("error in (no error)"=w2951, "Output"=w2945, "MotorControlDevRef"=w2952) -> ()  [unwired: 6 in, 3 out]
        n1292 = call "PIXY VI.vi"() -> ("X"=w2955:dbl)  [unwired: 14 in, 5 out]
        n1293 = call <vilib>:"WPI_RobotDriveRefNum Registry Get.vi"("refnum name"="RobotDrive") -> ("error out"=w2960:errorcluster, "RobotDriveDevRef"=w2961:T15)  [unwired: 9 in]
        n1294 = call-poly <vilib>:"PID.vi"("output range"=cluster{"output high":dbl, "output low":dbl} {"output high"=0.4, "output low"=-0.4}, "PID gains"=T7 {"proportional gain (Kc)"=0.11, "integral time (Ti, min)"=0.0, "derivative time (Td, min)"=0.0}, "process variable"=w2955, "setpoint"=0.0) -> ("output"=w2958:dbl)  [unwired: 6 in, 1 out]
        n1295 = Negate(x=w2958) -> (-x=w2957:dbl)
        n1296 = call-poly <vilib>:"WPI_RobotDriveArcadeDrive.vi"("error in (no error)"=w2960, "Y axis value"=w2948, "X axis value"=w2957, "RobotDriveDevRef"=w2961) -> ()  [unwired: 5 in, 3 out]
      }
      n1297 = while {
        tunnel: [w2854] -> w2745
        tunnel: w2749 -> [w2854]
        tunnel: [w2853] -> w2744
        tunnel: w2748 -> [w2853]
        tunnel: [w2856] -> w2743
        tunnel: w2747 -> [w2856]
        tunnel: [w2855] -> w2742
        tunnel: w2746 -> [w2855]
        i -> [w2879]
        stop <- w2875 stop-if-true
        n1298 = global read "Robot Global Data.vi" "YAW"() -> (w2864:dbl)
        n1299 = call <vilib>:"WPI_RobotDriveRefNum Registry Get.vi"("refnum name"="RobotDrive") -> ("error out"=w2862:errorcluster, "RobotDriveDevRef"=w2863:T15)  [unwired: 9 in]
        n1300 = Wait (ms)(milliseconds to wait=u32 20) -> ()  [unwired: 1 out]
        n1301 = Increment(x=w2879) -> (x+1=w2878:i32)
        n1302 = call-poly <vilib>:"PID.vi"("output range"=cluster{"output high":dbl, "output low":dbl} {"output high"=0.4, "output low"=-0.4}, "PID gains"=T7 {"proportional gain (Kc)"=0.11, "integral time (Ti, min)"=0.0, "derivative time (Td, min)"=0.0}, "process variable"=w2864, "setpoint"=-25.0) -> ("output"=w2858:dbl)  [unwired: 6 in, 1 out]
        n1303 = Greater Or Equal?(x=w2878, y=100) -> (x >= y?=w2876:bool)
        n1304 = Negate(x=w2858) -> (-x=w2857:dbl)
        n1305 = call-poly <vilib>:"CTRE_Phoenix_MotorController_Get_Enhanced.vi"("PhoenixMotorControlDevRef"=w2854, "error in"=w2853) -> ("Quadrature Position"=w2874:i32)  [unwired: 10 in, 3 out]
        n1306 = To Double Precision Float(number=w2874) -> (double precision float=w2873:dbl)
        n1307 = feedback #23() -> (w2859:dbl)  [unwired: 1 in]
        n1308 = call-poly <vilib>:"WPI_RobotDriveArcadeDrive.vi"("error in (no error)"=w2862, "Y axis value"=w2859, "X axis value"=w2857, "RobotDriveDevRef"=w2863) -> ()  [unwired: 5 in, 3 out]
        n1309 = Absolute Value(x=w2873) -> (abs(x)=w2869:dbl)
        n1310 = Greater Or Equal?(x=w2869, y=115000.0 ("upper limit")) -> (x >= y?=w2860:bool)
        n1311 = And(x=w2860, y=w2876) -> (x .and. y?=w2875:bool)
        n1312 = Select(t=0.0, s=w2860, f=-0.6) -> (s? t:f=w2870:dbl)
        n1313 = feedback-in #23(w2870) -> ()
      }
      n1314 = while {
        tunnel: w2745 -> [w2837]
        tunnel: w2744 -> [w2836]
        tunnel: w2743 -> [w2835]
        tunnel: w2742 -> [w2834]
        tunnel: [w2837] -> w2741
        tunnel: [w2836] -> w2740
        tunnel: [w2835] -> w2739
        tunnel: [w2834] -> w2738
        i -> [w2846]
        stop <- w2844 stop-if-true
        n1315 = global read "Robot Global Data.vi" "YAW"() -> (w2850:dbl)
        n1316 = Increment(x=w2846) -> (x+1=w2848:i32)
        n1317 = call-poly <vilib>:"PID.vi"("output range"=cluster{"output high":dbl, "output low":dbl} {"output high"=0.7, "output low"=-0.7}, "PID gains"=T7 {"proportional gain (Kc)"=0.045, "integral time (Ti, min)"=0.0, "derivative time (Td, min)"=0.0}, "process variable"=w2850, "setpoint"=-90.0) -> ("output"=w2839:dbl)  [unwired: 6 in, 1 out]
        n1318 = call <vilib>:"WPI_RobotDriveRefNum Registry Get.vi"("refnum name"="RobotDrive") -> ("error out"=w2842:errorcluster, "RobotDriveDevRef"=w2843:T15)  [unwired: 9 in]
        n1319 = Greater?(x=w2848, y=200) -> (0:w2844:bool)
        n1320 = Negate(x=w2839) -> (-x=w2838:dbl)
        n1321 = call-poly <vilib>:"WPI_RobotDriveArcadeDrive.vi"("error in (no error)"=w2842, "Y axis value"=0.0, "X axis value"=w2838, "RobotDriveDevRef"=w2843) -> ()  [unwired: 5 in, 3 out]
        n1322 = Wait (ms)(milliseconds to wait=u32 20) -> ()  [unwired: 1 out]
      }
      n1323 = while {
        tunnel: [w2911] -> w2737
        tunnel: w2741 -> [w2911]
        tunnel: w2740 -> [w2910]
        tunnel: [w2910] -> w2736
        tunnel: [w2913] -> w2735
        tunnel: w2739 -> [w2913]
        tunnel: [w2912] -> w2734
        tunnel: w2738 -> [w2912]
        i -> [w2937]
        stop <- w2933 stop-if-true
        n1324 = global read "Robot Global Data.vi" "YAW"() -> (w2921:dbl)
        n1325 = call <vilib>:"WPI_RobotDriveRefNum Registry Get.vi"("refnum name"="RobotDrive") -> ("error out"=w2919:errorcluster, "RobotDriveDevRef"=w2920:T15)  [unwired: 9 in]
        n1326 = Increment(x=w2937) -> (x+1=w2936:i32)
        n1327 = Wait (ms)(milliseconds to wait=u32 20) -> ()  [unwired: 1 out]
        n1328 = call-poly <vilib>:"PID.vi"("output range"=cluster{"output high":dbl, "output low":dbl} {"output high"=0.4, "output low"=-0.4}, "PID gains"=T7 {"proportional gain (Kc)"=0.11, "integral time (Ti, min)"=0.0, "derivative time (Td, min)"=0.0}, "process variable"=w2921, "setpoint"=0.0) -> ("output"=w2917:dbl)  [unwired: 6 in, 1 out]
        n1329 = Greater Or Equal?(x=w2936, y=20) -> (x >= y?=w2934:bool)
        n1330 = Negate(x=w2917) -> (-x=w2916:dbl)
        n1331 = Wait (ms)(milliseconds to wait=u32 20) -> ()  [unwired: 1 out]
        n1332 = call-poly <vilib>:"CTRE_Phoenix_MotorController_Get_Enhanced.vi"("PhoenixMotorControlDevRef"=w2911, "error in"=w2910) -> ("Quadrature Position"=w2932:i32)  [unwired: 10 in, 3 out]
        n1333 = To Double Precision Float(number=w2932) -> (double precision float=w2931:dbl)
        n1334 = feedback #24() -> (w2915:dbl)  [unwired: 1 in]
        n1335 = call-poly <vilib>:"WPI_RobotDriveArcadeDrive.vi"("error in (no error)"=w2919, "Y axis value"=w2915, "X axis value"=w2916, "RobotDriveDevRef"=w2920) -> ()  [unwired: 5 in, 3 out]
        n1336 = Absolute Value(x=w2931) -> (abs(x)=w2927:dbl)
        n1337 = Greater Or Equal?(x=w2927, y=113500.0 ("upper limit")) -> (x >= y?=w2925:bool)
        n1338 = And(x=w2925, y=w2934) -> (x .and. y?=w2933:bool)
        n1339 = Select(t=0.0, s=w2925, f=-0.6) -> (s? t:f=w2928:dbl)
        n1340 = feedback-in #24(w2928) -> ()
      }
      n1341 = while {
        tunnel: [w2799] -> _
        tunnel: w2737 -> [w2799]
        tunnel: [w2798] -> _
        tunnel: w2736 -> [w2798]
        tunnel: [w2797] -> _
        tunnel: w2735 -> [w2797]
        tunnel: [w2796] -> _
        tunnel: w2734 -> [w2796]
        i -> [w2823]
        stop <- w2800 stop-if-true
        # "Set config to shoot level, Rev, Shoot, and reset"
        n1342 = global read "Robot Global Data.vi" "Pot 1"() -> (w2828:dbl)
        n1343 = call <vilib>:"WPI_MotorControlRefNum Registry Get.vi"("refnum name"="Acquire") -> ("error out"=w2825:errorcluster, "MotorControlDevRef"=w2826:T8)  [unwired: 9 in]
        n1344 = call <vilib>:"WPI_MotorControlRefNum Registry Get.vi"("refnum name"="Dart 1") -> ("error out"=w2832:errorcluster, "MotorControlDevRef"=w2831:T8)  [unwired: 9 in]
        n1345 = Increment(x=w2823) -> (x+1=w2824:i32)
        n1346 = call-poly <vilib>:"PID.vi"("PID gains"=T7 {"proportional gain (Kc)"=1.0, "integral time (Ti, min)"=0.01, "derivative time (Td, min)"=0.0}, "process variable"=w2828, "setpoint"=0.0) -> ("output"=w2833:dbl)  [unwired: 7 in, 1 out]
        n1347 = Greater Or Equal?(x=w2824, y=100) -> (x >= y?=w2815:bool)
        n1348 = call <vilib>:"WPI_MotorControlSetOutput.vi"("error in (no error)"=w2832, "Output"=w2833, "MotorControlDevRef"=w2831) -> ()  [unwired: 6 in, 3 out]
        n1349 = call <vilib>:"WPI_MotorControlSetOutput.vi"("error in (no error)"=w2825, "Output"=-1.0, "MotorControlDevRef"=w2826) -> ()  [unwired: 6 in, 3 out]
        n1350 = Select(t=WPI_SolenoidValue."Forward" ("Value"), s=w2815, f=WPI_SolenoidValue."Off" ("Value")) -> (s? t:f=w2818:T6)
        n1351 = Wait (ms)(milliseconds to wait=u32 20) -> ()  [unwired: 1 out]
        n1352 = call <vilib>:"WPI_SolenoidRefNum Registry Get.vi"("refnum name"="Push") -> ("error out"=w2819:errorcluster, "SolenoidDevRef"=w2820:T16)  [unwired: 9 in]
        n1353 = call-poly <vilib>:"WPI_SolenoidSet.vi"("error in (no error)"=w2819, "Value"=w2818, "SolenoidDevRef"=w2820) -> ("error out"=w2811:errorcluster, "SolenoidDevRef"=w2812:T16)  [unwired: 7 in]
        n1354 = call-poly <vilib>:"WPI_SolenoidGet.vi"("error in (no error)"=w2811, "SolenoidDevRef"=w2812) -> ("Value"=w2810:bool)  [unwired: 7 in, 2 out]
        n1355 = And(x=w2815, y=w2810) -> (x .and. y?=w2801:bool)
        n1356 = Select(t=WPI_SolenoidValue."Reverse" ("Value"), s=w2801, f=WPI_SolenoidValue."Off" ("Value")) -> (s? t:f=w2806:T6)
        n1357 = call <vilib>:"WPI_SolenoidRefNum Registry Get.vi"("refnum name"="Push") -> ("error out"=w2807:errorcluster, "SolenoidDevRef"=w2808:T16)  [unwired: 9 in]
        n1358 = call-poly <vilib>:"WPI_SolenoidSet.vi"("error in (no error)"=w2807, "Value"=w2806, "SolenoidDevRef"=w2808) -> ("error out"=w2802:errorcluster, "SolenoidDevRef"=w2803:T16)  [unwired: 7 in]
        n1359 = call-poly <vilib>:"WPI_SolenoidGet.vi"("error in (no error)"=w2802, "SolenoidDevRef"=w2803) -> ("Value"=w2800:bool)  [unwired: 7 in, 2 out]
      }
    }
    frame "Do Nothing" {
      # "WHOO NOTHING."
    }
    frame "Center Place 2 Switch Right" {
      # "DONE"
      n1360 = call <vilib>:"WPI_MotorControlRefNum Registry Get.vi"("refnum name"="Left Lead") -> ("error out"=w3060:errorcluster, "MotorControlDevRef"=w3061:T8)  [unwired: 9 in]
      n1361 = call <vilib>:"WPI_MotorControlRefNum Registry Get.vi"("refnum name"="Right Lead") -> ("error out"=w3058:errorcluster, "MotorControlDevRef"=w3059:T8)  [unwired: 9 in]
      n1362 = while {
        tunnel: w3061 -> [w3343]
        tunnel: w3060 -> [w3342]
        tunnel: w3059 -> [w3341]
        tunnel: w3058 -> [w3340]
        tunnel: [w3343] -> w3101
        tunnel: [w3342] -> w3100
        tunnel: [w3341] -> w3099
        tunnel: [w3340] -> w3098
        i -> [w3353]
        stop <- w3352 stop-if-true
        n1363 = Increment(x=w3353) -> (x+1=w3355:i32)
        n1364 = Greater?(x=w3355, y=10) -> (0:w3352:bool)
        n1365 = call <vilib>:"CTRE_PigeonIMU_RefNumRegistryGet.vi"("refnum name"="Pigeon") -> ("PigeonIMUDevRef"=w3350:T13)  [unwired: 9 in, 1 out]
        n1366 = call-poly <vilib>:"CTRE_Phoenix_MotorController_Get_Enhanced.vi"("PhoenixMotorControlDevRef"=w3343, "error in"=w3342) -> ("PhoenixMotorControlDevRef"=w3345:T8)  [unwired: 10 in, 3 out]
        n1367 = call-poly <vilib>:"CTRE_Phoenix_MotorController_Get_Enhanced.vi"("PhoenixMotorControlDevRef"=w3341, "error in"=w3340) -> ("PhoenixMotorControlDevRef"=w3344:T8)  [unwired: 10 in, 3 out]
        n1368 = call "CTRE_Phoenix_MotorControl_SetQuadraturePosition_Enhanced.vi"("New Position"=0, "PhoenixMotorControlDevRef"=w3344) -> ()  [unwired: 8 in, 2 out]
        n1369 = call "CTRE_Phoenix_MotorControl_SetQuadraturePosition_Enhanced.vi"("New Position"=0, "PhoenixMotorControlDevRef"=w3345) -> ()  [unwired: 8 in, 2 out]
        n1370 = Wait (ms)(milliseconds to wait=u32 20) -> ()  [unwired: 1 out]
        n1371 = call <vilib>:"CTRE_PigeonIMU_SetYaw.vi"("Value"=0.0, "PigeonIMUDevRef"=w3350) -> ()  [unwired: 8 in, 2 out]
      }
      n1372 = while {
        tunnel: [w3358] -> w3097
        tunnel: w3101 -> [w3358]
        tunnel: [w3359] -> w3096
        tunnel: w3100 -> [w3359]
        tunnel: [w3366] -> w3095
        tunnel: w3099 -> [w3366]
        tunnel: [w3365] -> w3094
        tunnel: w3098 -> [w3365]
        i -> [w3382]
        stop <- w3378 stop-if-true
        n1373 = global read "Robot Global Data.vi" "YAW"() -> (w3367:dbl)
        n1374 = Wait (ms)(milliseconds to wait=u32 20) -> ()  [unwired: 1 out]
        n1375 = call <vilib>:"WPI_RobotDriveRefNum Registry Get.vi"("refnum name"="RobotDrive") -> ("error out"=w3363:errorcluster, "RobotDriveDevRef"=w3364:T15)  [unwired: 9 in]
        n1376 = Increment(x=w3382) -> (x+1=w3381:i32)
        n1377 = call-poly <vilib>:"PID.vi"("output range"=cluster{"output high":dbl, "output low":dbl} {"output high"=0.4, "output low"=-0.4}, "PID gains"=T7 {"proportional gain (Kc)"=0.11, "integral time (Ti, min)"=0.0, "derivative time (Td, min)"=0.0}, "process variable"=w3367, "setpoint"=0.0) -> ("output"=w3357:dbl)  [unwired: 6 in, 1 out]
        n1378 = Greater Or Equal?(x=w3381, y=100) -> (x >= y?=w3379:bool)
        n1379 = Negate(x=w3357) -> (-x=w3356:dbl)
        n1380 = call-poly <vilib>:"CTRE_Phoenix_MotorController_Get_Enhanced.vi"("PhoenixMotorControlDevRef"=w3358, "error in"=w3359) -> ("Quadrature Position"=w3377:i32)  [unwired: 10 in, 3 out]
        n1381 = To Double Precision Float(number=w3377) -> (double precision float=w3376:dbl)
        n1382 = feedback #25() -> (w3360:dbl)  [unwired: 1 in]
        n1383 = call-poly <vilib>:"WPI_RobotDriveArcadeDrive.vi"("error in (no error)"=w3363, "Y axis value"=w3360, "X axis value"=w3356, "RobotDriveDevRef"=w3364) -> ()  [unwired: 5 in, 3 out]
        n1384 = Absolute Value(x=w3376) -> (abs(x)=w3372:dbl)
        n1385 = Greater Or Equal?(x=w3372, y=115000.0 ("upper limit")) -> (x >= y?=w3361:bool)
        n1386 = And(x=w3361, y=w3379) -> (x .and. y?=w3378:bool)
        n1387 = Select(t=0.0, s=w3361, f=-0.8) -> (s? t:f=w3373:dbl)
        n1388 = feedback-in #25(w3373) -> ()
      }
      n1389 = while {
        tunnel: w3097 -> [w3330]
        tunnel: w3096 -> [w3329]
        tunnel: w3095 -> [w3328]
        tunnel: w3094 -> [w3327]
        tunnel: [w3330] -> w3093
        tunnel: [w3329] -> w3092
        tunnel: [w3328] -> w3091
        tunnel: [w3327] -> w3090
        i -> [w3333]
        stop <- w3331 stop-if-true
        n1390 = global read "Robot Global Data.vi" "YAW"() -> (w3337:dbl)
        n1391 = Increment(x=w3333) -> (x+1=w3335:i32)
        n1392 = call-poly <vilib>:"PID.vi"("output range"=cluster{"output high":dbl, "output low":dbl} {"output high"=0.7, "output low"=-0.7}, "PID gains"=T7 {"proportional gain (Kc)"=0.045, "integral time (Ti, min)"=0.0, "derivative time (Td, min)"=0.0}, "process variable"=w3337, "setpoint"=-90.0) -> ("output"=w3322:dbl)  [unwired: 6 in, 1 out]
        n1393 = call <vilib>:"WPI_RobotDriveRefNum Registry Get.vi"("refnum name"="RobotDrive") -> ("error out"=w3325:errorcluster, "RobotDriveDevRef"=w3326:T15)  [unwired: 9 in]
        n1394 = Greater?(x=w3335, y=200) -> (0:w3331:bool)
        n1395 = Negate(x=w3322) -> (-x=w3321:dbl)
        n1396 = call-poly <vilib>:"WPI_RobotDriveArcadeDrive.vi"("error in (no error)"=w3325, "Y axis value"=0.0, "X axis value"=w3321, "RobotDriveDevRef"=w3326) -> ()  [unwired: 5 in, 3 out]
        n1397 = Wait (ms)(milliseconds to wait=u32 20) -> ()  [unwired: 1 out]
      }
      n1398 = while {
        tunnel: [w3230] -> w3089
        tunnel: w3093 -> [w3230]
        tunnel: [w3229] -> w3088
        tunnel: w3092 -> [w3229]
        tunnel: [w3228] -> w3087
        tunnel: w3091 -> [w3228]
        tunnel: [w3231] -> w3086
        tunnel: w3090 -> [w3231]
        i -> [w3224]
        stop <- w3210 stop-if-true
        # "Set config to shoot level, Rev, Shoot"
        n1399 = global read "Robot Global Data.vi" "Pot 1"() -> (w3232:dbl)
        n1400 = call <vilib>:"WPI_MotorControlRefNum Registry Get.vi"("refnum name"="Acquire") -> ("error out"=w3225:errorcluster, "MotorControlDevRef"=w3226:T8)  [unwired: 9 in]
        n1401 = call <vilib>:"WPI_MotorControlRefNum Registry Get.vi"("refnum name"="Dart 1") -> ("error out"=w3236:errorcluster, "MotorControlDevRef"=w3235:T8)  [unwired: 9 in]
        n1402 = Increment(x=w3224) -> (x+1=w3211:i32)
        n1403 = call-poly <vilib>:"PID.vi"("PID gains"=T7 {"proportional gain (Kc)"=1.0, "integral time (Ti, min)"=0.01, "derivative time (Td, min)"=0.0}, "process variable"=w3232, "setpoint"=0.0) -> ("output"=w3237:dbl)  [unwired: 7 in, 1 out]
        n1404 = Greater Or Equal?(x=w3211, y=100) -> (x >= y?=w3216:bool)
        n1405 = call <vilib>:"WPI_MotorControlSetOutput.vi"("error in (no error)"=w3236, "Output"=w3237, "MotorControlDevRef"=w3235) -> ()  [unwired: 6 in, 3 out]
        n1406 = call <vilib>:"WPI_MotorControlSetOutput.vi"("error in (no error)"=w3225, "Output"=-1.0, "MotorControlDevRef"=w3226) -> ()  [unwired: 6 in, 3 out]
        n1407 = Select(t=WPI_SolenoidValue."Forward" ("Value"), s=w3216, f=WPI_SolenoidValue."Off" ("Value")) -> (s? t:f=w3219:T6)
        n1408 = Wait (ms)(milliseconds to wait=u32 20) -> ()  [unwired: 1 out]
        n1409 = call <vilib>:"WPI_SolenoidRefNum Registry Get.vi"("refnum name"="Push") -> ("error out"=w3220:errorcluster, "SolenoidDevRef"=w3221:T16)  [unwired: 9 in]
        n1410 = call-poly <vilib>:"WPI_SolenoidSet.vi"("error in (no error)"=w3220, "Value"=w3219, "SolenoidDevRef"=w3221) -> ("error out"=w3212:errorcluster, "SolenoidDevRef"=w3213:T16)  [unwired: 7 in]
        n1411 = call-poly <vilib>:"WPI_SolenoidGet.vi"("error in (no error)"=w3212, "SolenoidDevRef"=w3213) -> ("Value"=w3210:bool)  [unwired: 7 in, 2 out]
      }
      n1412 = while {
        tunnel: w3089 -> [w3116]
        tunnel: w3088 -> [w3115]
        tunnel: w3087 -> [w3114]
        tunnel: w3086 -> [w3113]
        tunnel: [w3116] -> w3085
        tunnel: [w3115] -> w3084
        tunnel: [w3114] -> w3083
        tunnel: [w3113] -> w3082
        i -> [w3104]
        stop <- w3103 stop-if-true
        # "Reset"
        n1413 = call <vilib>:"WPI_SolenoidRefNum Registry Get.vi"("refnum name"="Push") -> ("error out"=w3120:errorcluster, "SolenoidDevRef"=w3121:T16)  [unwired: 9 in]
        n1414 = call <vilib>:"WPI_MotorControlRefNum Registry Get.vi"("refnum name"="Dart 1") -> ("error out"=w3111:errorcluster, "MotorControlDevRef"=w3110:T8)  [unwired: 9 in]
        n1415 = Increment(x=w3104) -> (x+1=w3117:i32)
        n1416 = global read "Robot Global Data.vi" "Pot 1"() -> (w3107:dbl)
        n1417 = Greater Or Equal?(x=w3117, y=100) -> (x >= y?=w3103:bool)
        n1418 = call-poly <vilib>:"PID.vi"("PID gains"=T7 {"proportional gain (Kc)"=1.0, "integral time (Ti, min)"=0.01, "derivative time (Td, min)"=0.0}, "process variable"=w3107, "setpoint"=0.0) -> ("output"=w3112:dbl)  [unwired: 7 in, 1 out]
        n1419 = call <vilib>:"WPI_MotorControlSetOutput.vi"("error in (no error)"=w3111, "Output"=w3112, "MotorControlDevRef"=w3110) -> ()  [unwired: 6 in, 3 out]
        n1420 = call-poly <vilib>:"WPI_SolenoidSet.vi"("error in (no error)"=w3120, "Value"=WPI_SolenoidValue."Reverse", "SolenoidDevRef"=w3121) -> ("error out"=w3118:errorcluster, "SolenoidDevRef"=w3119:T16)  [unwired: 7 in]
        n1421 = call-poly <vilib>:"WPI_SolenoidGet.vi"("error in (no error)"=w3118, "SolenoidDevRef"=w3119) -> ()  [unwired: 7 in, 3 out]
      }
      n1422 = while {
        tunnel: [w3301] -> w3081
        tunnel: w3085 -> [w3301]
        tunnel: [w3300] -> w3080
        tunnel: w3084 -> [w3300]
        tunnel: [w3299] -> w3079
        tunnel: w3083 -> [w3299]
        tunnel: [w3298] -> w3078
        tunnel: w3082 -> [w3298]
        i -> [w3314]
        stop <- w3312 stop-if-true
        n1423 = global read "Robot Global Data.vi" "YAW"() -> (w3318:dbl)
        n1424 = Increment(x=w3314) -> (x+1=w3316:i32)
        n1425 = call-poly <vilib>:"PID.vi"("output range"=cluster{"output high":dbl, "output low":dbl} {"output high"=0.6, "output low"=-0.6}, "PID gains"=T7 {"proportional gain (Kc)"=0.055, "integral time (Ti, min)"=0.0, "derivative time (Td, min)"=0.0}, "process variable"=w3318, "setpoint"=-25.0) -> ("output"=w3308:dbl)  [unwired: 6 in, 1 out]
        n1426 = call <vilib>:"WPI_RobotDriveRefNum Registry Get.vi"("refnum name"="RobotDrive") -> ("error out"=w3309:errorcluster, "RobotDriveDevRef"=w3310:T15)  [unwired: 9 in]
        n1427 = Negate(x=w3308) -> (-x=w3307:dbl)
        n1428 = Greater?(x=w3316, y=180) -> (0:w3312:bool)
        n1429 = call-poly <vilib>:"WPI_RobotDriveArcadeDrive.vi"("error in (no error)"=w3309, "Y axis value"=0.0, "X axis value"=w3307, "RobotDriveDevRef"=w3310) -> ()  [unwired: 5 in, 3 out]
        n1430 = Wait (ms)(milliseconds to wait=u32 20) -> ()  [unwired: 1 out]
        n1431 = call-poly <vilib>:"CTRE_Phoenix_MotorController_Get_Enhanced.vi"("PhoenixMotorControlDevRef"=w3301, "error in"=w3300) -> ("PhoenixMotorControlDevRef"=w3303:T8)  [unwired: 8 in, 5 out]
        n1432 = call-poly <vilib>:"CTRE_Phoenix_MotorController_Get_Enhanced.vi"("PhoenixMotorControlDevRef"=w3299, "error in"=w3298) -> ("PhoenixMotorControlDevRef"=w3302:T8)  [unwired: 8 in, 5 out]
        n1433 = call "CTRE_Phoenix_MotorControl_SetQuadraturePosition_Enhanced.vi"("New Position"=0, "PhoenixMotorControlDevRef"=w3302) -> ()  [unwired: 8 in, 2 out]
        n1434 = call "CTRE_Phoenix_MotorControl_SetQuadraturePosition_Enhanced.vi"("New Position"=0, "PhoenixMotorControlDevRef"=w3303) -> ()  [unwired: 8 in, 2 out]
      }
      n1435 = while {
        tunnel: [w3271] -> w3077
        tunnel: w3081 -> [w3271]
        tunnel: [w3270] -> w3076
        tunnel: w3080 -> [w3270]
        tunnel: [w3269] -> w3075
        tunnel: w3079 -> [w3269]
        tunnel: [w3268] -> w3074
        tunnel: w3078 -> [w3268]
        i -> [w3296]
        stop <- w3292 stop-if-true
        # "Drives towards cube, uses pixy cam's \"x\" value to stay on center"
        n1436 = Increment(x=w3296) -> (x+1=w3295:i32)
        n1437 = Greater Or Equal?(x=w3295, y=100) -> (x >= y?=w3293:bool)
        n1438 = call <vilib>:"WPI_DigitalInputRefNum Registry Get.vi"("refnum name"="Color Mark") -> ("DigitalInputDevRef"=w3282:T18)  [unwired: 9 in, 1 out]
        n1439 = call <vilib>:"WPI_MotorControlRefNum Registry Get.vi"("refnum name"="Acquire") -> ("error out"=w3279:errorcluster, "MotorControlDevRef"=w3280:T8)  [unwired: 9 in]
        n1440 = call <vilib>:"WPI_DigitalInputGetValue.vi"("DigitalInputDevRef"=w3282) -> ("Value"=w3272:bool)  [unwired: 8 in, 2 out]
        n1441 = And(x=w3272, y=w3293) -> (x .and. y?=w3292:bool)
        n1442 = Wait (ms)(milliseconds to wait=u32 20) -> ()  [unwired: 1 out]
        n1443 = Select(t=0.0, s=w3272, f=0.6) -> (s? t:f=w3273:dbl)
        n1444 = Select(t=0.0, s=w3272, f=0.6) -> (s? t:f=w3276:dbl)
        n1445 = call <vilib>:"WPI_MotorControlSetOutput.vi"("error in (no error)"=w3279, "Output"=w3273, "MotorControlDevRef"=w3280) -> ()  [unwired: 6 in, 3 out]
        n1446 = call "PIXY VI.vi"() -> ("X"=w3283:dbl)  [unwired: 14 in, 5 out]
        n1447 = call <vilib>:"WPI_RobotDriveRefNum Registry Get.vi"("refnum name"="RobotDrive") -> ("error out"=w3288:errorcluster, "RobotDriveDevRef"=w3289:T15)  [unwired: 9 in]
        n1448 = call-poly <vilib>:"PID.vi"("output range"=cluster{"output high":dbl, "output low":dbl} {"output high"=0.4, "output low"=-0.4}, "PID gains"=T7 {"proportional gain (Kc)"=0.11, "integral time (Ti, min)"=0.0, "derivative time (Td, min)"=0.0}, "process variable"=w3283, "setpoint"=0.0) -> ("output"=w3286:dbl)  [unwired: 6 in, 1 out]
        n1449 = Negate(x=w3286) -> (-x=w3285:dbl)
        n1450 = call-poly <vilib>:"WPI_RobotDriveArcadeDrive.vi"("error in (no error)"=w3288, "Y axis value"=w3276, "X axis value"=w3285, "RobotDriveDevRef"=w3289) -> ()  [unwired: 5 in, 3 out]
      }
      n1451 = while {
        tunnel: [w3182] -> w3073
        tunnel: w3077 -> [w3182]
        tunnel: [w3181] -> w3072
        tunnel: w3076 -> [w3181]
        tunnel: [w3184] -> w3071
        tunnel: w3075 -> [w3184]
        tunnel: [w3183] -> w3070
        tunnel: w3074 -> [w3183]
        i -> [w3207]
        stop <- w3203 stop-if-true
        n1452 = global read "Robot Global Data.vi" "YAW"() -> (w3192:dbl)
        n1453 = call <vilib>:"WPI_RobotDriveRefNum Registry Get.vi"("refnum name"="RobotDrive") -> ("error out"=w3190:errorcluster, "RobotDriveDevRef"=w3191:T15)  [unwired: 9 in]
        n1454 = Wait (ms)(milliseconds to wait=u32 20) -> ()  [unwired: 1 out]
        n1455 = Increment(x=w3207) -> (x+1=w3206:i32)
        n1456 = call-poly <vilib>:"PID.vi"("output range"=cluster{"output high":dbl, "output low":dbl} {"output high"=0.4, "output low"=-0.4}, "PID gains"=T7 {"proportional gain (Kc)"=0.11, "integral time (Ti, min)"=0.0, "derivative time (Td, min)"=0.0}, "process variable"=w3192, "setpoint"=-25.0) -> ("output"=w3186:dbl)  [unwired: 6 in, 1 out]
        n1457 = Greater Or Equal?(x=w3206, y=100) -> (x >= y?=w3204:bool)
        n1458 = Negate(x=w3186) -> (-x=w3185:dbl)
        n1459 = call-poly <vilib>:"CTRE_Phoenix_MotorController_Get_Enhanced.vi"("PhoenixMotorControlDevRef"=w3182, "error in"=w3181) -> ("Quadrature Position"=w3202:i32)  [unwired: 10 in, 3 out]
        n1460 = To Double Precision Float(number=w3202) -> (double precision float=w3201:dbl)
        n1461 = feedback #26() -> (w3187:dbl)  [unwired: 1 in]
        n1462 = call-poly <vilib>:"WPI_RobotDriveArcadeDrive.vi"("error in (no error)"=w3190, "Y axis value"=w3187, "X axis value"=w3185, "RobotDriveDevRef"=w3191) -> ()  [unwired: 5 in, 3 out]
        n1463 = Absolute Value(x=w3201) -> (abs(x)=w3197:dbl)
        n1464 = Greater Or Equal?(x=w3197, y=115000.0 ("upper limit")) -> (x >= y?=w3188:bool)
        n1465 = And(x=w3188, y=w3204) -> (x .and. y?=w3203:bool)
        n1466 = Select(t=0.0, s=w3188, f=-0.6) -> (s? t:f=w3198:dbl)
        n1467 = feedback-in #26(w3198) -> ()
      }
      n1468 = while {
        tunnel: w3073 -> [w3165]
        tunnel: w3072 -> [w3164]
        tunnel: w3071 -> [w3163]
        tunnel: w3070 -> [w3162]
        tunnel: [w3165] -> w3069
        tunnel: [w3164] -> w3068
        tunnel: [w3163] -> w3067
        tunnel: [w3162] -> w3066
        i -> [w3174]
        stop <- w3172 stop-if-true
        n1469 = global read "Robot Global Data.vi" "YAW"() -> (w3178:dbl)
        n1470 = Increment(x=w3174) -> (x+1=w3176:i32)
        n1471 = call-poly <vilib>:"PID.vi"("output range"=cluster{"output high":dbl, "output low":dbl} {"output high"=0.7, "output low"=-0.7}, "PID gains"=T7 {"proportional gain (Kc)"=0.045, "integral time (Ti, min)"=0.0, "derivative time (Td, min)"=0.0}, "process variable"=w3178, "setpoint"=-90.0) -> ("output"=w3167:dbl)  [unwired: 6 in, 1 out]
        n1472 = call <vilib>:"WPI_RobotDriveRefNum Registry Get.vi"("refnum name"="RobotDrive") -> ("error out"=w3170:errorcluster, "RobotDriveDevRef"=w3171:T15)  [unwired: 9 in]
        n1473 = Greater?(x=w3176, y=200) -> (0:w3172:bool)
        n1474 = Negate(x=w3167) -> (-x=w3166:dbl)
        n1475 = call-poly <vilib>:"WPI_RobotDriveArcadeDrive.vi"("error in (no error)"=w3170, "Y axis value"=0.0, "X axis value"=w3166, "RobotDriveDevRef"=w3171) -> ()  [unwired: 5 in, 3 out]
        n1476 = Wait (ms)(milliseconds to wait=u32 20) -> ()  [unwired: 1 out]
      }
      n1477 = while {
        tunnel: [w3239] -> w3065
        tunnel: w3069 -> [w3239]
        tunnel: w3068 -> [w3238]
        tunnel: [w3238] -> w3064
        tunnel: [w3241] -> w3063
        tunnel: w3067 -> [w3241]
        tunnel: [w3240] -> w3062
        tunnel: w3066 -> [w3240]
        i -> [w3265]
        stop <- w3261 stop-if-true
        n1478 = global read "Robot Global Data.vi" "YAW"() -> (w3249:dbl)
        n1479 = call <vilib>:"WPI_RobotDriveRefNum Registry Get.vi"("refnum name"="RobotDrive") -> ("error out"=w3247:errorcluster, "RobotDriveDevRef"=w3248:T15)  [unwired: 9 in]
        n1480 = Increment(x=w3265) -> (x+1=w3264:i32)
        n1481 = Wait (ms)(milliseconds to wait=u32 20) -> ()  [unwired: 1 out]
        n1482 = call-poly <vilib>:"PID.vi"("output range"=cluster{"output high":dbl, "output low":dbl} {"output high"=0.4, "output low"=-0.4}, "PID gains"=T7 {"proportional gain (Kc)"=0.11, "integral time (Ti, min)"=0.0, "derivative time (Td, min)"=0.0}, "process variable"=w3249, "setpoint"=0.0) -> ("output"=w3245:dbl)  [unwired: 6 in, 1 out]
        n1483 = Greater Or Equal?(x=w3264, y=20) -> (x >= y?=w3262:bool)
        n1484 = Negate(x=w3245) -> (-x=w3244:dbl)
        n1485 = Wait (ms)(milliseconds to wait=u32 20) -> ()  [unwired: 1 out]
        n1486 = call-poly <vilib>:"CTRE_Phoenix_MotorController_Get_Enhanced.vi"("PhoenixMotorControlDevRef"=w3239, "error in"=w3238) -> ("Quadrature Position"=w3260:i32)  [unwired: 10 in, 3 out]
        n1487 = To Double Precision Float(number=w3260) -> (double precision float=w3259:dbl)
        n1488 = feedback #27() -> (w3243:dbl)  [unwired: 1 in]
        n1489 = call-poly <vilib>:"WPI_RobotDriveArcadeDrive.vi"("error in (no error)"=w3247, "Y axis value"=w3243, "X axis value"=w3244, "RobotDriveDevRef"=w3248) -> ()  [unwired: 5 in, 3 out]
        n1490 = Absolute Value(x=w3259) -> (abs(x)=w3255:dbl)
        n1491 = Greater Or Equal?(x=w3255, y=113500.0 ("upper limit")) -> (x >= y?=w3253:bool)
        n1492 = And(x=w3253, y=w3262) -> (x .and. y?=w3261:bool)
        n1493 = Select(t=0.0, s=w3253, f=-0.6) -> (s? t:f=w3256:dbl)
        n1494 = feedback-in #27(w3256) -> ()
      }
      n1495 = while {
        tunnel: [w3127] -> _
        tunnel: w3065 -> [w3127]
        tunnel: [w3126] -> _
        tunnel: w3064 -> [w3126]
        tunnel: [w3125] -> _
        tunnel: w3063 -> [w3125]
        tunnel: [w3124] -> _
        tunnel: w3062 -> [w3124]
        i -> [w3151]
        stop <- w3128 stop-if-true
        # "Set config to shoot level, Rev, Shoot, and reset"
        n1496 = global read "Robot Global Data.vi" "Pot 1"() -> (w3156:dbl)
        n1497 = call <vilib>:"WPI_MotorControlRefNum Registry Get.vi"("refnum name"="Acquire") -> ("error out"=w3153:errorcluster, "MotorControlDevRef"=w3154:T8)  [unwired: 9 in]
        n1498 = call <vilib>:"WPI_MotorControlRefNum Registry Get.vi"("refnum name"="Dart 1") -> ("error out"=w3160:errorcluster, "MotorControlDevRef"=w3159:T8)  [unwired: 9 in]
        n1499 = Increment(x=w3151) -> (x+1=w3152:i32)
        n1500 = call-poly <vilib>:"PID.vi"("PID gains"=T7 {"proportional gain (Kc)"=1.0, "integral time (Ti, min)"=0.01, "derivative time (Td, min)"=0.0}, "process variable"=w3156, "setpoint"=0.0) -> ("output"=w3161:dbl)  [unwired: 7 in, 1 out]
        n1501 = Greater Or Equal?(x=w3152, y=100) -> (x >= y?=w3143:bool)
        n1502 = call <vilib>:"WPI_MotorControlSetOutput.vi"("error in (no error)"=w3160, "Output"=w3161, "MotorControlDevRef"=w3159) -> ()  [unwired: 6 in, 3 out]
        n1503 = call <vilib>:"WPI_MotorControlSetOutput.vi"("error in (no error)"=w3153, "Output"=-1.0, "MotorControlDevRef"=w3154) -> ()  [unwired: 6 in, 3 out]
        n1504 = Select(t=WPI_SolenoidValue."Forward" ("Value"), s=w3143, f=WPI_SolenoidValue."Off" ("Value")) -> (s? t:f=w3146:T6)
        n1505 = Wait (ms)(milliseconds to wait=u32 20) -> ()  [unwired: 1 out]
        n1506 = call <vilib>:"WPI_SolenoidRefNum Registry Get.vi"("refnum name"="Push") -> ("error out"=w3147:errorcluster, "SolenoidDevRef"=w3148:T16)  [unwired: 9 in]
        n1507 = call-poly <vilib>:"WPI_SolenoidSet.vi"("error in (no error)"=w3147, "Value"=w3146, "SolenoidDevRef"=w3148) -> ("error out"=w3139:errorcluster, "SolenoidDevRef"=w3140:T16)  [unwired: 7 in]
        n1508 = call-poly <vilib>:"WPI_SolenoidGet.vi"("error in (no error)"=w3139, "SolenoidDevRef"=w3140) -> ("Value"=w3138:bool)  [unwired: 7 in, 2 out]
        n1509 = And(x=w3143, y=w3138) -> (x .and. y?=w3129:bool)
        n1510 = Select(t=WPI_SolenoidValue."Reverse" ("Value"), s=w3129, f=WPI_SolenoidValue."Off" ("Value")) -> (s? t:f=w3134:T6)
        n1511 = call <vilib>:"WPI_SolenoidRefNum Registry Get.vi"("refnum name"="Push") -> ("error out"=w3135:errorcluster, "SolenoidDevRef"=w3136:T16)  [unwired: 9 in]
        n1512 = call-poly <vilib>:"WPI_SolenoidSet.vi"("error in (no error)"=w3135, "Value"=w3134, "SolenoidDevRef"=w3136) -> ("error out"=w3130:errorcluster, "SolenoidDevRef"=w3131:T16)  [unwired: 7 in]
        n1513 = call-poly <vilib>:"WPI_SolenoidGet.vi"("error in (no error)"=w3130, "SolenoidDevRef"=w3131) -> ("Value"=w3128:bool)  [unwired: 7 in, 2 out]
      }
    }
    frame "Place Scale Left" {
      # "done"
      n1514 = call <vilib>:"WPI_MotorControlRefNum Registry Get.vi"("refnum name"="Left Lead") -> ("error out"=w3388:errorcluster, "MotorControlDevRef"=w3389:T8)  [unwired: 9 in]
      n1515 = call <vilib>:"WPI_MotorControlRefNum Registry Get.vi"("refnum name"="Right Lead") -> ("error out"=w3386:errorcluster, "MotorControlDevRef"=w3387:T8)  [unwired: 9 in]
      n1516 = while {
        tunnel: w3389 -> [w3478]
        tunnel: w3388 -> [w3477]
        tunnel: w3387 -> [w3476]
        tunnel: w3386 -> [w3475]
        tunnel: [w3478] -> w3405
        tunnel: [w3477] -> w3404
        tunnel: [w3476] -> w3403
        tunnel: [w3475] -> w3402
        i -> [w3488]
        stop <- w3487 stop-if-true
        n1517 = Increment(x=w3488) -> (x+1=w3490:i32)
        n1518 = Greater?(x=w3490, y=10) -> (0:w3487:bool)
        n1519 = call <vilib>:"CTRE_PigeonIMU_RefNumRegistryGet.vi"("refnum name"="Pigeon") -> ("PigeonIMUDevRef"=w3485:T13)  [unwired: 9 in, 1 out]
        n1520 = call-poly <vilib>:"CTRE_Phoenix_MotorController_Get_Enhanced.vi"("PhoenixMotorControlDevRef"=w3478, "error in"=w3477) -> ("PhoenixMotorControlDevRef"=w3480:T8)  [unwired: 10 in, 3 out]
        n1521 = call-poly <vilib>:"CTRE_Phoenix_MotorController_Get_Enhanced.vi"("PhoenixMotorControlDevRef"=w3476, "error in"=w3475) -> ("PhoenixMotorControlDevRef"=w3479:T8)  [unwired: 10 in, 3 out]
        n1522 = call "CTRE_Phoenix_MotorControl_SetQuadraturePosition_Enhanced.vi"("New Position"=0, "PhoenixMotorControlDevRef"=w3479) -> ()  [unwired: 8 in, 2 out]
        n1523 = call "CTRE_Phoenix_MotorControl_SetQuadraturePosition_Enhanced.vi"("New Position"=0, "PhoenixMotorControlDevRef"=w3480) -> ()  [unwired: 8 in, 2 out]
        n1524 = Wait (ms)(milliseconds to wait=u32 20) -> ()  [unwired: 1 out]
        n1525 = call <vilib>:"CTRE_PigeonIMU_SetYaw.vi"("Value"=0.0, "PigeonIMUDevRef"=w3485) -> ()  [unwired: 8 in, 2 out]
      }
      n1526 = while {
        tunnel: [w3493] -> w3401
        tunnel: w3405 -> [w3493]
        tunnel: [w3494] -> w3400
        tunnel: w3404 -> [w3494]
        tunnel: [w3501] -> w3399
        tunnel: w3403 -> [w3501]
        tunnel: [w3500] -> w3398
        tunnel: w3402 -> [w3500]
        i -> [w3517]
        stop <- w3513 stop-if-true
        n1527 = global read "Robot Global Data.vi" "YAW"() -> (w3502:dbl)
        n1528 = Wait (ms)(milliseconds to wait=u32 20) -> ()  [unwired: 1 out]
        n1529 = call <vilib>:"WPI_RobotDriveRefNum Registry Get.vi"("refnum name"="RobotDrive") -> ("error out"=w3498:errorcluster, "RobotDriveDevRef"=w3499:T15)  [unwired: 9 in]
        n1530 = Increment(x=w3517) -> (x+1=w3516:i32)
        n1531 = call-poly <vilib>:"PID.vi"("output range"=cluster{"output high":dbl, "output low":dbl} {"output high"=0.4, "output low"=-0.4}, "PID gains"=T7 {"proportional gain (Kc)"=0.11, "integral time (Ti, min)"=0.0, "derivative time (Td, min)"=0.0}, "process variable"=w3502, "setpoint"=0.0) -> ("output"=w3492:dbl)  [unwired: 6 in, 1 out]
        n1532 = Greater Or Equal?(x=w3516, y=100) -> (x >= y?=w3514:bool)
        n1533 = Negate(x=w3492) -> (-x=w3491:dbl)
        n1534 = call-poly <vilib>:"CTRE_Phoenix_MotorController_Get_Enhanced.vi"("PhoenixMotorControlDevRef"=w3493, "error in"=w3494) -> ("Quadrature Position"=w3512:i32)  [unwired: 10 in, 3 out]
        n1535 = To Double Precision Float(number=w3512) -> (double precision float=w3511:dbl)
        n1536 = feedback #28() -> (w3495:dbl)  [unwired: 1 in]
        n1537 = call-poly <vilib>:"WPI_RobotDriveArcadeDrive.vi"("error in (no error)"=w3498, "Y axis value"=w3495, "X axis value"=w3491, "RobotDriveDevRef"=w3499) -> ()  [unwired: 5 in, 3 out]
        n1538 = Absolute Value(x=w3511) -> (abs(x)=w3507:dbl)
        n1539 = Greater Or Equal?(x=w3507, y=115000.0 ("upper limit")) -> (x >= y?=w3496:bool)
        n1540 = And(x=w3496, y=w3514) -> (x .and. y?=w3513:bool)
        n1541 = Select(t=0.0, s=w3496, f=-0.8) -> (s? t:f=w3508:dbl)
        n1542 = feedback-in #28(w3508) -> ()
      }
      n1543 = while {
        tunnel: w3401 -> [w3465]
        tunnel: w3400 -> [w3464]
        tunnel: w3399 -> [w3463]
        tunnel: w3398 -> [w3462]
        tunnel: [w3465] -> w3397
        tunnel: [w3464] -> w3396
        tunnel: [w3463] -> w3395
        tunnel: [w3462] -> w3394
        i -> [w3468]
        stop <- w3466 stop-if-true
        n1544 = global read "Robot Global Data.vi" "YAW"() -> (w3472:dbl)
        n1545 = Increment(x=w3468) -> (x+1=w3470:i32)
        n1546 = call-poly <vilib>:"PID.vi"("output range"=cluster{"output high":dbl, "output low":dbl} {"output high"=0.7, "output low"=-0.7}, "PID gains"=T7 {"proportional gain (Kc)"=0.045, "integral time (Ti, min)"=0.0, "derivative time (Td, min)"=0.0}, "process variable"=w3472, "setpoint"=-90.0) -> ("output"=w3457:dbl)  [unwired: 6 in, 1 out]
        n1547 = call <vilib>:"WPI_RobotDriveRefNum Registry Get.vi"("refnum name"="RobotDrive") -> ("error out"=w3460:errorcluster, "RobotDriveDevRef"=w3461:T15)  [unwired: 9 in]
        n1548 = Greater?(x=w3470, y=200) -> (0:w3466:bool)
        n1549 = Negate(x=w3457) -> (-x=w3456:dbl)
        n1550 = call-poly <vilib>:"WPI_RobotDriveArcadeDrive.vi"("error in (no error)"=w3460, "Y axis value"=0.0, "X axis value"=w3456, "RobotDriveDevRef"=w3461) -> ()  [unwired: 5 in, 3 out]
        n1551 = Wait (ms)(milliseconds to wait=u32 20) -> ()  [unwired: 1 out]
      }
      n1552 = while {
        tunnel: [w3448] -> w3393
        tunnel: w3397 -> [w3448]
        tunnel: [w3447] -> w3392
        tunnel: w3396 -> [w3447]
        tunnel: [w3446] -> w3391
        tunnel: w3395 -> [w3446]
        tunnel: [w3449] -> w3390
        tunnel: w3394 -> [w3449]
        i -> [w3442]
        stop <- w3428 stop-if-true
        # "Set config to shoot level, Rev, Shoot"
        n1553 = global read "Robot Global Data.vi" "Pot 1"() -> (w3450:dbl)
        n1554 = call <vilib>:"WPI_MotorControlRefNum Registry Get.vi"("refnum name"="Acquire") -> ("error out"=w3443:errorcluster, "MotorControlDevRef"=w3444:T8)  [unwired: 9 in]
        n1555 = call <vilib>:"WPI_MotorControlRefNum Registry Get.vi"("refnum name"="Dart 1") -> ("error out"=w3454:errorcluster, "MotorControlDevRef"=w3453:T8)  [unwired: 9 in]
        n1556 = Increment(x=w3442) -> (x+1=w3429:i32)
        n1557 = call-poly <vilib>:"PID.vi"("PID gains"=T7 {"proportional gain (Kc)"=1.0, "integral time (Ti, min)"=0.01, "derivative time (Td, min)"=0.0}, "process variable"=w3450, "setpoint"=0.0) -> ("output"=w3455:dbl)  [unwired: 7 in, 1 out]
        n1558 = Greater Or Equal?(x=w3429, y=100) -> (x >= y?=w3434:bool)
        n1559 = call <vilib>:"WPI_MotorControlSetOutput.vi"("error in (no error)"=w3454, "Output"=w3455, "MotorControlDevRef"=w3453) -> ()  [unwired: 6 in, 3 out]
        n1560 = call <vilib>:"WPI_MotorControlSetOutput.vi"("error in (no error)"=w3443, "Output"=-1.0, "MotorControlDevRef"=w3444) -> ()  [unwired: 6 in, 3 out]
        n1561 = Select(t=WPI_SolenoidValue."Forward" ("Value"), s=w3434, f=WPI_SolenoidValue."Off" ("Value")) -> (s? t:f=w3437:T6)
        n1562 = Wait (ms)(milliseconds to wait=u32 20) -> ()  [unwired: 1 out]
        n1563 = call <vilib>:"WPI_SolenoidRefNum Registry Get.vi"("refnum name"="Push") -> ("error out"=w3438:errorcluster, "SolenoidDevRef"=w3439:T16)  [unwired: 9 in]
        n1564 = call-poly <vilib>:"WPI_SolenoidSet.vi"("error in (no error)"=w3438, "Value"=w3437, "SolenoidDevRef"=w3439) -> ("error out"=w3430:errorcluster, "SolenoidDevRef"=w3431:T16)  [unwired: 7 in]
        n1565 = call-poly <vilib>:"WPI_SolenoidGet.vi"("error in (no error)"=w3430, "SolenoidDevRef"=w3431) -> ("Value"=w3428:bool)  [unwired: 7 in, 2 out]
      }
      n1566 = while {
        tunnel: w3393 -> [w3420]
        tunnel: w3392 -> [w3419]
        tunnel: w3391 -> [w3418]
        tunnel: w3390 -> [w3417]
        tunnel: [w3420] -> _
        tunnel: [w3419] -> _
        tunnel: [w3418] -> _
        tunnel: [w3417] -> _
        i -> [w3408]
        stop <- w3407 stop-if-true
        # "Reset"
        n1567 = call <vilib>:"WPI_SolenoidRefNum Registry Get.vi"("refnum name"="Push") -> ("error out"=w3424:errorcluster, "SolenoidDevRef"=w3425:T16)  [unwired: 9 in]
        n1568 = call <vilib>:"WPI_MotorControlRefNum Registry Get.vi"("refnum name"="Dart 1") -> ("error out"=w3415:errorcluster, "MotorControlDevRef"=w3414:T8)  [unwired: 9 in]
        n1569 = Increment(x=w3408) -> (x+1=w3421:i32)
        n1570 = global read "Robot Global Data.vi" "Pot 1"() -> (w3411:dbl)
        n1571 = Greater Or Equal?(x=w3421, y=100) -> (x >= y?=w3407:bool)
        n1572 = call-poly <vilib>:"PID.vi"("PID gains"=T7 {"proportional gain (Kc)"=1.0, "integral time (Ti, min)"=0.01, "derivative time (Td, min)"=0.0}, "process variable"=w3411, "setpoint"=0.0) -> ("output"=w3416:dbl)  [unwired: 7 in, 1 out]
        n1573 = call <vilib>:"WPI_MotorControlSetOutput.vi"("error in (no error)"=w3415, "Output"=w3416, "MotorControlDevRef"=w3414) -> ()  [unwired: 6 in, 3 out]
        n1574 = call-poly <vilib>:"WPI_SolenoidSet.vi"("error in (no error)"=w3424, "Value"=WPI_SolenoidValue."Reverse", "SolenoidDevRef"=w3425) -> ("error out"=w3422:errorcluster, "SolenoidDevRef"=w3423:T16)  [unwired: 7 in]
        n1575 = call-poly <vilib>:"WPI_SolenoidGet.vi"("error in (no error)"=w3422, "SolenoidDevRef"=w3423) -> ()  [unwired: 7 in, 3 out]
      }
    }
    frame "Place Switch and Scale Left" {
      # "DONE"
      n1576 = call <vilib>:"WPI_MotorControlRefNum Registry Get.vi"("refnum name"="Left Lead") -> ("error out"=w3571:errorcluster, "MotorControlDevRef"=w3572:T8)  [unwired: 9 in]
      n1577 = call <vilib>:"WPI_MotorControlRefNum Registry Get.vi"("refnum name"="Right Lead") -> ("error out"=w3569:errorcluster, "MotorControlDevRef"=w3570:T8)  [unwired: 9 in]
      n1578 = while {
        tunnel: w3572 -> [w3894]
        tunnel: w3571 -> [w3893]
        tunnel: w3570 -> [w3892]
        tunnel: w3569 -> [w3891]
        tunnel: [w3894] -> w3580
        tunnel: [w3893] -> w3579
        tunnel: [w3892] -> w3578
        tunnel: [w3891] -> w3577
        i -> [w3904]
        stop <- w3903 stop-if-true
        n1579 = Increment(x=w3904) -> (x+1=w3906:i32)
        n1580 = Greater?(x=w3906, y=10) -> (0:w3903:bool)
        n1581 = call <vilib>:"CTRE_PigeonIMU_RefNumRegistryGet.vi"("refnum name"="Pigeon") -> ("PigeonIMUDevRef"=w3901:T13)  [unwired: 9 in, 1 out]
        n1582 = call-poly <vilib>:"CTRE_Phoenix_MotorController_Get_Enhanced.vi"("PhoenixMotorControlDevRef"=w3894, "error in"=w3893) -> ("PhoenixMotorControlDevRef"=w3896:T8)  [unwired: 10 in, 3 out]
        n1583 = call-poly <vilib>:"CTRE_Phoenix_MotorController_Get_Enhanced.vi"("PhoenixMotorControlDevRef"=w3892, "error in"=w3891) -> ("PhoenixMotorControlDevRef"=w3895:T8)  [unwired: 10 in, 3 out]
        n1584 = call "CTRE_Phoenix_MotorControl_SetQuadraturePosition_Enhanced.vi"("New Position"=0, "PhoenixMotorControlDevRef"=w3895) -> ()  [unwired: 8 in, 2 out]
        n1585 = call "CTRE_Phoenix_MotorControl_SetQuadraturePosition_Enhanced.vi"("New Position"=0, "PhoenixMotorControlDevRef"=w3896) -> ()  [unwired: 8 in, 2 out]
        n1586 = Wait (ms)(milliseconds to wait=u32 20) -> ()  [unwired: 1 out]
        n1587 = call <vilib>:"CTRE_PigeonIMU_SetYaw.vi"("Value"=0.0, "PigeonIMUDevRef"=w3901) -> ()  [unwired: 8 in, 2 out]
      }
      n1588 = while {
        tunnel: [w3909] -> w3576
        tunnel: w3580 -> [w3909]
        tunnel: [w3910] -> w3575
        tunnel: w3579 -> [w3910]
        tunnel: [w3917] -> w3574
        tunnel: w3578 -> [w3917]
        tunnel: [w3916] -> w3573
        tunnel: w3577 -> [w3916]
        i -> [w3933]
        stop <- w3929 stop-if-true
        n1589 = global read "Robot Global Data.vi" "YAW"() -> (w3918:dbl)
        n1590 = Wait (ms)(milliseconds to wait=u32 20) -> ()  [unwired: 1 out]
        n1591 = call <vilib>:"WPI_RobotDriveRefNum Registry Get.vi"("refnum name"="RobotDrive") -> ("error out"=w3914:errorcluster, "RobotDriveDevRef"=w3915:T15)  [unwired: 9 in]
        n1592 = Increment(x=w3933) -> (x+1=w3932:i32)
        n1593 = call-poly <vilib>:"PID.vi"("output range"=cluster{"output high":dbl, "output low":dbl} {"output high"=0.4, "output low"=-0.4}, "PID gains"=T7 {"proportional gain (Kc)"=0.11, "integral time (Ti, min)"=0.0, "derivative time (Td, min)"=0.0}, "process variable"=w3918, "setpoint"=0.0) -> ("output"=w3908:dbl)  [unwired: 6 in, 1 out]
        n1594 = Greater Or Equal?(x=w3932, y=100) -> (x >= y?=w3930:bool)
        n1595 = Negate(x=w3908) -> (-x=w3907:dbl)
        n1596 = call-poly <vilib>:"CTRE_Phoenix_MotorController_Get_Enhanced.vi"("PhoenixMotorControlDevRef"=w3909, "error in"=w3910) -> ("Quadrature Position"=w3928:i32)  [unwired: 10 in, 3 out]
        n1597 = To Double Precision Float(number=w3928) -> (double precision float=w3927:dbl)
        n1598 = feedback #29() -> (w3911:dbl)  [unwired: 1 in]
        n1599 = call-poly <vilib>:"WPI_RobotDriveArcadeDrive.vi"("error in (no error)"=w3914, "Y axis value"=w3911, "X axis value"=w3907, "RobotDriveDevRef"=w3915) -> ()  [unwired: 5 in, 3 out]
        n1600 = Absolute Value(x=w3927) -> (abs(x)=w3923:dbl)
        n1601 = Greater Or Equal?(x=w3923, y=115000.0 ("upper limit")) -> (x >= y?=w3912:bool)
        n1602 = And(x=w3912, y=w3930) -> (x .and. y?=w3929:bool)
        n1603 = Select(t=0.0, s=w3912, f=-0.8) -> (s? t:f=w3924:dbl)
        n1604 = feedback-in #29(w3924) -> ()
      }
      n1605 = while {
        tunnel: w3576 -> [w3881]
        tunnel: w3575 -> [w3880]
        tunnel: w3574 -> [w3879]
        tunnel: w3573 -> [w3878]
        tunnel: [w3881] -> w3558
        tunnel: [w3880] -> w3557
        tunnel: [w3879] -> w3556
        tunnel: [w3878] -> w3555
        i -> [w3884]
        stop <- w3882 stop-if-true
        n1606 = global read "Robot Global Data.vi" "YAW"() -> (w3888:dbl)
        n1607 = Increment(x=w3884) -> (x+1=w3886:i32)
        n1608 = call-poly <vilib>:"PID.vi"("output range"=cluster{"output high":dbl, "output low":dbl} {"output high"=0.7, "output low"=-0.7}, "PID gains"=T7 {"proportional gain (Kc)"=0.045, "integral time (Ti, min)"=0.0, "derivative time (Td, min)"=0.0}, "process variable"=w3888, "setpoint"=-90.0) -> ("output"=w3873:dbl)  [unwired: 6 in, 1 out]
        n1609 = call <vilib>:"WPI_RobotDriveRefNum Registry Get.vi"("refnum name"="RobotDrive") -> ("error out"=w3876:errorcluster, "RobotDriveDevRef"=w3877:T15)  [unwired: 9 in]
        n1610 = Greater?(x=w3886, y=200) -> (0:w3882:bool)
        n1611 = Negate(x=w3873) -> (-x=w3872:dbl)
        n1612 = call-poly <vilib>:"WPI_RobotDriveArcadeDrive.vi"("error in (no error)"=w3876, "Y axis value"=25.0, "X axis value"=w3872, "RobotDriveDevRef"=w3877) -> ()  [unwired: 5 in, 3 out]
        n1613 = Wait (ms)(milliseconds to wait=u32 20) -> ()  [unwired: 1 out]
      }
      n1614 = while {
        tunnel: [w3623] -> w3562
        tunnel: w3558 -> [w3623]
        tunnel: [w3622] -> w3561
        tunnel: w3557 -> [w3622]
        tunnel: [w3621] -> w3560
        tunnel: w3556 -> [w3621]
        tunnel: [w3624] -> w3559
        tunnel: w3555 -> [w3624]
        i -> [w3617]
        stop <- w3603 stop-if-true
        # "Set config to shoot level, Rev, Shoot"
        n1615 = global read "Robot Global Data.vi" "Pot 1"() -> (w3625:dbl)
        n1616 = call <vilib>:"WPI_MotorControlRefNum Registry Get.vi"("refnum name"="Acquire") -> ("error out"=w3618:errorcluster, "MotorControlDevRef"=w3619:T8)  [unwired: 9 in]
        n1617 = call <vilib>:"WPI_MotorControlRefNum Registry Get.vi"("refnum name"="Dart 1") -> ("error out"=w3629:errorcluster, "MotorControlDevRef"=w3628:T8)  [unwired: 9 in]
        n1618 = Increment(x=w3617) -> (x+1=w3604:i32)
        n1619 = call-poly <vilib>:"PID.vi"("PID gains"=T7 {"proportional gain (Kc)"=1.0, "integral time (Ti, min)"=0.01, "derivative time (Td, min)"=0.0}, "process variable"=w3625, "setpoint"=0.0) -> ("output"=w3630:dbl)  [unwired: 7 in, 1 out]
        n1620 = Greater Or Equal?(x=w3604, y=100) -> (x >= y?=w3609:bool)
        n1621 = call <vilib>:"WPI_MotorControlSetOutput.vi"("error in (no error)"=w3629, "Output"=w3630, "MotorControlDevRef"=w3628) -> ()  [unwired: 6 in, 3 out]
        n1622 = call <vilib>:"WPI_MotorControlSetOutput.vi"("error in (no error)"=w3618, "Output"=-1.0, "MotorControlDevRef"=w3619) -> ()  [unwired: 6 in, 3 out]
        n1623 = Select(t=WPI_SolenoidValue."Forward" ("Value"), s=w3609, f=WPI_SolenoidValue."Off" ("Value")) -> (s? t:f=w3612:T6)
        n1624 = Wait (ms)(milliseconds to wait=u32 20) -> ()  [unwired: 1 out]
        n1625 = call <vilib>:"WPI_SolenoidRefNum Registry Get.vi"("refnum name"="Push") -> ("error out"=w3613:errorcluster, "SolenoidDevRef"=w3614:T16)  [unwired: 9 in]
        n1626 = call-poly <vilib>:"WPI_SolenoidSet.vi"("error in (no error)"=w3613, "Value"=w3612, "SolenoidDevRef"=w3614) -> ("error out"=w3605:errorcluster, "SolenoidDevRef"=w3606:T16)  [unwired: 7 in]
        n1627 = call-poly <vilib>:"WPI_SolenoidGet.vi"("error in (no error)"=w3605, "SolenoidDevRef"=w3606) -> ("Value"=w3603:bool)  [unwired: 7 in, 2 out]
      }
      n1628 = while {
        tunnel: w3562 -> [w3595]
        tunnel: w3561 -> [w3594]
        tunnel: w3560 -> [w3593]
        tunnel: w3559 -> [w3592]
        tunnel: [w3595] -> w3554
        tunnel: [w3594] -> w3553
        tunnel: [w3593] -> w3552
        tunnel: [w3592] -> w3551
        i -> [w3583]
        stop <- w3582 stop-if-true
        # "Reset"
        n1629 = call <vilib>:"WPI_SolenoidRefNum Registry Get.vi"("refnum name"="Push") -> ("error out"=w3599:errorcluster, "SolenoidDevRef"=w3600:T16)  [unwired: 9 in]
        n1630 = call <vilib>:"WPI_MotorControlRefNum Registry Get.vi"("refnum name"="Dart 1") -> ("error out"=w3590:errorcluster, "MotorControlDevRef"=w3589:T8)  [unwired: 9 in]
        n1631 = Increment(x=w3583) -> (x+1=w3596:i32)
        n1632 = global read "Robot Global Data.vi" "Pot 1"() -> (w3586:dbl)
        n1633 = call-poly <vilib>:"PID.vi"("PID gains"=T7 {"proportional gain (Kc)"=1.0, "integral time (Ti, min)"=0.01, "derivative time (Td, min)"=0.0}, "process variable"=w3586, "setpoint"=0.0) -> ("output"=w3591:dbl)  [unwired: 7 in, 1 out]
        n1634 = call <vilib>:"WPI_MotorControlSetOutput.vi"("error in (no error)"=w3590, "Output"=w3591, "MotorControlDevRef"=w3589) -> ()  [unwired: 6 in, 3 out]
        n1635 = call-poly <vilib>:"WPI_SolenoidSet.vi"("error in (no error)"=w3599, "Value"=WPI_SolenoidValue."Reverse", "SolenoidDevRef"=w3600) -> ("error out"=w3597:errorcluster, "SolenoidDevRef"=w3598:T16)  [unwired: 7 in]
        n1636 = Greater Or Equal?(x=w3596, y=100) -> (x >= y?=w3582:bool)
        n1637 = call-poly <vilib>:"WPI_SolenoidGet.vi"("error in (no error)"=w3597, "SolenoidDevRef"=w3598) -> ()  [unwired: 7 in, 3 out]
      }
      n1638 = while {
        tunnel: w3554 -> [w3812]
        tunnel: w3553 -> [w3811]
        tunnel: w3552 -> [w3810]
        tunnel: w3551 -> [w3809]
        tunnel: [w3812] -> w3550
        tunnel: [w3811] -> w3549
        tunnel: [w3810] -> w3547
        tunnel: [w3809] -> w3548
        i -> [w3815]
        stop <- w3813 stop-if-true
        n1639 = global read "Robot Global Data.vi" "YAW"() -> (w3819:dbl)
        n1640 = Increment(x=w3815) -> (x+1=w3817:i32)
        n1641 = call-poly <vilib>:"PID.vi"("output range"=cluster{"output high":dbl, "output low":dbl} {"output high"=0.7, "output low"=-0.7}, "PID gains"=T7 {"proportional gain (Kc)"=0.045, "integral time (Ti, min)"=0.0, "derivative time (Td, min)"=0.0}, "process variable"=w3819, "setpoint"=0.0) -> ("output"=w3804:dbl)  [unwired: 6 in, 1 out]
        n1642 = call <vilib>:"WPI_RobotDriveRefNum Registry Get.vi"("refnum name"="RobotDrive") -> ("error out"=w3807:errorcluster, "RobotDriveDevRef"=w3808:T15)  [unwired: 9 in]
        n1643 = Greater?(x=w3817, y=200) -> (0:w3813:bool)
        n1644 = Negate(x=w3804) -> (-x=w3803:dbl)
        n1645 = call-poly <vilib>:"WPI_RobotDriveArcadeDrive.vi"("error in (no error)"=w3807, "Y axis value"=25.0, "X axis value"=w3803, "RobotDriveDevRef"=w3808) -> ()  [unwired: 5 in, 3 out]
        n1646 = Wait (ms)(milliseconds to wait=u32 20) -> ()  [unwired: 1 out]
      }
      n1647 = while {
        tunnel: [w3777] -> w3546
        tunnel: w3550 -> [w3777]
        tunnel: [w3778] -> w3545
        tunnel: w3549 -> [w3778]
        tunnel: [w3785] -> w3544
        tunnel: w3547 -> [w3785]
        tunnel: [w3784] -> w3543
        tunnel: w3548 -> [w3784]
        i -> [w3801]
        stop <- w3797 stop-if-true
        n1648 = global read "Robot Global Data.vi" "YAW"() -> (w3786:dbl)
        n1649 = Wait (ms)(milliseconds to wait=u32 20) -> ()  [unwired: 1 out]
        n1650 = call <vilib>:"WPI_RobotDriveRefNum Registry Get.vi"("refnum name"="RobotDrive") -> ("error out"=w3782:errorcluster, "RobotDriveDevRef"=w3783:T15)  [unwired: 9 in]
        n1651 = Increment(x=w3801) -> (x+1=w3800:i32)
        n1652 = call-poly <vilib>:"PID.vi"("output range"=cluster{"output high":dbl, "output low":dbl} {"output high"=0.4, "output low"=-0.4}, "PID gains"=T7 {"proportional gain (Kc)"=0.11, "integral time (Ti, min)"=0.0, "derivative time (Td, min)"=0.0}, "process variable"=w3786, "setpoint"=0.0) -> ("output"=w3776:dbl)  [unwired: 6 in, 1 out]
        n1653 = Greater Or Equal?(x=w3800, y=100) -> (x >= y?=w3798:bool)
        n1654 = Negate(x=w3776) -> (-x=w3775:dbl)
        n1655 = call-poly <vilib>:"CTRE_Phoenix_MotorController_Get_Enhanced.vi"("PhoenixMotorControlDevRef"=w3777, "error in"=w3778) -> ("Quadrature Position"=w3796:i32)  [unwired: 10 in, 3 out]
        n1656 = To Double Precision Float(number=w3796) -> (double precision float=w3795:dbl)
        n1657 = feedback #30() -> (w3779:dbl)  [unwired: 1 in]
        n1658 = call-poly <vilib>:"WPI_RobotDriveArcadeDrive.vi"("error in (no error)"=w3782, "Y axis value"=w3779, "X axis value"=w3775, "RobotDriveDevRef"=w3783) -> ()  [unwired: 5 in, 3 out]
        n1659 = Absolute Value(x=w3795) -> (abs(x)=w3791:dbl)
        n1660 = Greater Or Equal?(x=w3791, y=115000.0 ("upper limit")) -> (x >= y?=w3780:bool)
        n1661 = And(x=w3780, y=w3798) -> (x .and. y?=w3797:bool)
        n1662 = Select(t=0.0, s=w3780, f=-0.8) -> (s? t:f=w3792:dbl)
        n1663 = feedback-in #30(w3792) -> ()
      }
      n1664 = while {
        tunnel: w3546 -> [w3765]
        tunnel: w3545 -> [w3764]
        tunnel: w3544 -> [w3763]
        tunnel: w3543 -> [w3762]
        tunnel: [w3765] -> w3542
        tunnel: [w3764] -> w3541
        tunnel: [w3763] -> w3540
        tunnel: [w3762] -> w3539
        i -> [w3768]
        stop <- w3766 stop-if-true
        n1665 = global read "Robot Global Data.vi" "YAW"() -> (w3772:dbl)
        n1666 = Increment(x=w3768) -> (x+1=w3770:i32)
        n1667 = call-poly <vilib>:"PID.vi"("output range"=cluster{"output high":dbl, "output low":dbl} {"output high"=0.7, "output low"=-0.7}, "PID gains"=T7 {"proportional gain (Kc)"=0.045, "integral time (Ti, min)"=0.0, "derivative time (Td, min)"=0.0}, "process variable"=w3772, "setpoint"=-90.0) -> ("output"=w3757:dbl)  [unwired: 6 in, 1 out]
        n1668 = call <vilib>:"WPI_RobotDriveRefNum Registry Get.vi"("refnum name"="RobotDrive") -> ("error out"=w3760:errorcluster, "RobotDriveDevRef"=w3761:T15)  [unwired: 9 in]
        n1669 = Greater?(x=w3770, y=200) -> (0:w3766:bool)
        n1670 = Negate(x=w3757) -> (-x=w3756:dbl)
        n1671 = call-poly <vilib>:"WPI_RobotDriveArcadeDrive.vi"("error in (no error)"=w3760, "Y axis value"=25.0, "X axis value"=w3756, "RobotDriveDevRef"=w3761) -> ()  [unwired: 5 in, 3 out]
        n1672 = Wait (ms)(milliseconds to wait=u32 20) -> ()  [unwired: 1 out]
      }
      n1673 = while {
        tunnel: [w3729] -> w3538
        tunnel: w3542 -> [w3729]
        tunnel: [w3728] -> w3537
        tunnel: w3541 -> [w3728]
        tunnel: [w3727] -> w3536
        tunnel: w3540 -> [w3727]
        tunnel: [w3726] -> w3535
        tunnel: w3539 -> [w3726]
        i -> [w3754]
        stop <- w3750 stop-if-true
        # "Drives towards cube, uses pixy cam's \"x\" value to stay on center"
        n1674 = Increment(x=w3754) -> (x+1=w3753:i32)
        n1675 = Greater Or Equal?(x=w3753, y=100) -> (x >= y?=w3751:bool)
        n1676 = call <vilib>:"WPI_DigitalInputRefNum Registry Get.vi"("refnum name"="Color Mark") -> ("DigitalInputDevRef"=w3740:T18)  [unwired: 9 in, 1 out]
        n1677 = call <vilib>:"WPI_MotorControlRefNum Registry Get.vi"("refnum name"="Acquire") -> ("error out"=w3737:errorcluster, "MotorControlDevRef"=w3738:T8)  [unwired: 9 in]
        n1678 = call <vilib>:"WPI_DigitalInputGetValue.vi"("DigitalInputDevRef"=w3740) -> ("Value"=w3730:bool)  [unwired: 8 in, 2 out]
        n1679 = And(x=w3730, y=w3751) -> (x .and. y?=w3750:bool)
        n1680 = Wait (ms)(milliseconds to wait=u32 20) -> ()  [unwired: 1 out]
        n1681 = Select(t=0.0, s=w3730, f=0.6) -> (s? t:f=w3731:dbl)
        n1682 = Select(t=0.0, s=w3730, f=0.6) -> (s? t:f=w3734:dbl)
        n1683 = call <vilib>:"WPI_MotorControlSetOutput.vi"("error in (no error)"=w3737, "Output"=w3731, "MotorControlDevRef"=w3738) -> ()  [unwired: 6 in, 3 out]
        n1684 = call "PIXY VI.vi"() -> ("X"=w3741:dbl)  [unwired: 14 in, 5 out]
        n1685 = call <vilib>:"WPI_RobotDriveRefNum Registry Get.vi"("refnum name"="RobotDrive") -> ("error out"=w3746:errorcluster, "RobotDriveDevRef"=w3747:T15)  [unwired: 9 in]
        n1686 = call-poly <vilib>:"PID.vi"("output range"=cluster{"output high":dbl, "output low":dbl} {"output high"=0.4, "output low"=-0.4}, "PID gains"=T7 {"proportional gain (Kc)"=0.11, "integral time (Ti, min)"=0.0, "derivative time (Td, min)"=0.0}, "process variable"=w3741, "setpoint"=0.0) -> ("output"=w3744:dbl)  [unwired: 6 in, 1 out]
        n1687 = Negate(x=w3744) -> (-x=w3743:dbl)
        n1688 = call-poly <vilib>:"WPI_RobotDriveArcadeDrive.vi"("error in (no error)"=w3746, "Y axis value"=w3734, "X axis value"=w3743, "RobotDriveDevRef"=w3747) -> ()  [unwired: 5 in, 3 out]
      }
      n1689 = while {
        tunnel: [w3699] -> w3534
        tunnel: w3538 -> [w3699]
        tunnel: [w3700] -> w3533
        tunnel: w3537 -> [w3700]
        tunnel: [w3707] -> w3532
        tunnel: w3536 -> [w3707]
        tunnel: [w3706] -> w3531
        tunnel: w3535 -> [w3706]
        i -> [w3723]
        stop <- w3719 stop-if-true
        n1690 = global read "Robot Global Data.vi" "YAW"() -> (w3708:dbl)
        n1691 = Wait (ms)(milliseconds to wait=u32 20) -> ()  [unwired: 1 out]
        n1692 = call <vilib>:"WPI_RobotDriveRefNum Registry Get.vi"("refnum name"="RobotDrive") -> ("error out"=w3704:errorcluster, "RobotDriveDevRef"=w3705:T15)  [unwired: 9 in]
        n1693 = Increment(x=w3723) -> (x+1=w3722:i32)
        n1694 = call-poly <vilib>:"PID.vi"("output range"=cluster{"output high":dbl, "output low":dbl} {"output high"=0.4, "output low"=-0.4}, "PID gains"=T7 {"proportional gain (Kc)"=0.11, "integral time (Ti, min)"=0.0, "derivative time (Td, min)"=0.0}, "process variable"=w3708, "setpoint"=0.0) -> ("output"=w3698:dbl)  [unwired: 6 in, 1 out]
        n1695 = Greater Or Equal?(x=w3722, y=100) -> (x >= y?=w3720:bool)
        n1696 = Negate(x=w3698) -> (-x=w3697:dbl)
        n1697 = call-poly <vilib>:"CTRE_Phoenix_MotorController_Get_Enhanced.vi"("PhoenixMotorControlDevRef"=w3699, "error in"=w3700) -> ("Quadrature Position"=w3718:i32)  [unwired: 10 in, 3 out]
        n1698 = To Double Precision Float(number=w3718) -> (double precision float=w3717:dbl)
        n1699 = feedback #31() -> (w3701:dbl)  [unwired: 1 in]
        n1700 = call-poly <vilib>:"WPI_RobotDriveArcadeDrive.vi"("error in (no error)"=w3704, "Y axis value"=w3701, "X axis value"=w3697, "RobotDriveDevRef"=w3705) -> ()  [unwired: 5 in, 3 out]
        n1701 = Absolute Value(x=w3717) -> (abs(x)=w3713:dbl)
        n1702 = Greater Or Equal?(x=w3713, y=115000.0 ("upper limit")) -> (x >= y?=w3702:bool)
        n1703 = And(x=w3702, y=w3720) -> (x .and. y?=w3719:bool)
        n1704 = Select(t=0.0, s=w3702, f=-0.8) -> (s? t:f=w3714:dbl)
        n1705 = feedback-in #31(w3714) -> ()
      }
      n1706 = while {
        tunnel: w3534 -> [w3687]
        tunnel: w3533 -> [w3686]
        tunnel: w3532 -> [w3685]
        tunnel: w3531 -> [w3684]
        tunnel: [w3687] -> w3530
        tunnel: [w3686] -> w3529
        tunnel: [w3685] -> w3528
        tunnel: [w3684] -> w3527
        i -> [w3690]
        stop <- w3688 stop-if-true
        n1707 = global read "Robot Global Data.vi" "YAW"() -> (w3694:dbl)
        n1708 = Increment(x=w3690) -> (x+1=w3692:i32)
        n1709 = call-poly <vilib>:"PID.vi"("output range"=cluster{"output high":dbl, "output low":dbl} {"output high"=0.7, "output low"=-0.7}, "PID gains"=T7 {"proportional gain (Kc)"=0.045, "integral time (Ti, min)"=0.0, "derivative time (Td, min)"=0.0}, "process variable"=w3694, "setpoint"=0.0) -> ("output"=w3679:dbl)  [unwired: 6 in, 1 out]
        n1710 = call <vilib>:"WPI_RobotDriveRefNum Registry Get.vi"("refnum name"="RobotDrive") -> ("error out"=w3682:errorcluster, "RobotDriveDevRef"=w3683:T15)  [unwired: 9 in]
        n1711 = Greater?(x=w3692, y=200) -> (0:w3688:bool)
        n1712 = Negate(x=w3679) -> (-x=w3678:dbl)
        n1713 = call-poly <vilib>:"WPI_RobotDriveArcadeDrive.vi"("error in (no error)"=w3682, "Y axis value"=25.0, "X axis value"=w3678, "RobotDriveDevRef"=w3683) -> ()  [unwired: 5 in, 3 out]
        n1714 = Wait (ms)(milliseconds to wait=u32 20) -> ()  [unwired: 1 out]
      }
      n1715 = while {
        tunnel: [w3652] -> w3526
        tunnel: w3530 -> [w3652]
        tunnel: [w3653] -> w3525
        tunnel: w3529 -> [w3653]
        tunnel: [w3660] -> w3524
        tunnel: w3528 -> [w3660]
        tunnel: [w3659] -> w3523
        tunnel: w3527 -> [w3659]
        i -> [w3676]
        stop <- w3672 stop-if-true
        n1716 = global read "Robot Global Data.vi" "YAW"() -> (w3661:dbl)
        n1717 = Wait (ms)(milliseconds to wait=u32 20) -> ()  [unwired: 1 out]
        n1718 = call <vilib>:"WPI_RobotDriveRefNum Registry Get.vi"("refnum name"="RobotDrive") -> ("error out"=w3657:errorcluster, "RobotDriveDevRef"=w3658:T15)  [unwired: 9 in]
        n1719 = Increment(x=w3676) -> (x+1=w3675:i32)
        n1720 = call-poly <vilib>:"PID.vi"("output range"=cluster{"output high":dbl, "output low":dbl} {"output high"=0.4, "output low"=-0.4}, "PID gains"=T7 {"proportional gain (Kc)"=0.11, "integral time (Ti, min)"=0.0, "derivative time (Td, min)"=0.0}, "process variable"=w3661, "setpoint"=0.0) -> ("output"=w3651:dbl)  [unwired: 6 in, 1 out]
        n1721 = Greater Or Equal?(x=w3675, y=100) -> (x >= y?=w3673:bool)
        n1722 = Negate(x=w3651) -> (-x=w3650:dbl)
        n1723 = call-poly <vilib>:"CTRE_Phoenix_MotorController_Get_Enhanced.vi"("PhoenixMotorControlDevRef"=w3652, "error in"=w3653) -> ("Quadrature Position"=w3671:i32)  [unwired: 10 in, 3 out]
        n1724 = To Double Precision Float(number=w3671) -> (double precision float=w3670:dbl)
        n1725 = feedback #32() -> (w3654:dbl)  [unwired: 1 in]
        n1726 = call-poly <vilib>:"WPI_RobotDriveArcadeDrive.vi"("error in (no error)"=w3657, "Y axis value"=w3654, "X axis value"=w3650, "RobotDriveDevRef"=w3658) -> ()  [unwired: 5 in, 3 out]
        n1727 = Absolute Value(x=w3670) -> (abs(x)=w3666:dbl)
        n1728 = Greater Or Equal?(x=w3666, y=115000.0 ("upper limit")) -> (x >= y?=w3655:bool)
        n1729 = And(x=w3655, y=w3673) -> (x .and. y?=w3672:bool)
        n1730 = Select(t=0.0, s=w3655, f=-0.8) -> (s? t:f=w3667:dbl)
        n1731 = feedback-in #32(w3667) -> ()
      }
      n1732 = while {
        tunnel: w3526 -> [w3640]
        tunnel: w3525 -> [w3639]
        tunnel: w3524 -> [w3638]
        tunnel: w3523 -> [w3637]
        tunnel: [w3640] -> w3522
        tunnel: [w3639] -> w3521
        tunnel: [w3638] -> w3520
        tunnel: [w3637] -> w3519
        i -> [w3643]
        stop <- w3641 stop-if-true
        n1733 = global read "Robot Global Data.vi" "YAW"() -> (w3647:dbl)
        n1734 = Increment(x=w3643) -> (x+1=w3645:i32)
        n1735 = call-poly <vilib>:"PID.vi"("output range"=cluster{"output high":dbl, "output low":dbl} {"output high"=0.7, "output low"=-0.7}, "PID gains"=T7 {"proportional gain (Kc)"=0.045, "integral time (Ti, min)"=0.0, "derivative time (Td, min)"=0.0}, "process variable"=w3647, "setpoint"=-90.0) -> ("output"=w3632:dbl)  [unwired: 6 in, 1 out]
        n1736 = call <vilib>:"WPI_RobotDriveRefNum Registry Get.vi"("refnum name"="RobotDrive") -> ("error out"=w3635:errorcluster, "RobotDriveDevRef"=w3636:T15)  [unwired: 9 in]
        n1737 = Greater?(x=w3645, y=200) -> (0:w3641:bool)
        n1738 = Negate(x=w3632) -> (-x=w3631:dbl)
        n1739 = call-poly <vilib>:"WPI_RobotDriveArcadeDrive.vi"("error in (no error)"=w3635, "Y axis value"=25.0, "X axis value"=w3631, "RobotDriveDevRef"=w3636) -> ()  [unwired: 5 in, 3 out]
        n1740 = Wait (ms)(milliseconds to wait=u32 20) -> ()  [unwired: 1 out]
      }
      n1741 = while {
        tunnel: [w3864] -> w3566
        tunnel: w3522 -> [w3864]
        tunnel: [w3863] -> w3565
        tunnel: w3521 -> [w3863]
        tunnel: [w3862] -> w3564
        tunnel: w3520 -> [w3862]
        tunnel: [w3865] -> w3563
        tunnel: w3519 -> [w3865]
        i -> [w3858]
        stop <- w3844 stop-if-true
        # "Set config to shoot level, Rev, Shoot"
        n1742 = global read "Robot Global Data.vi" "Pot 1"() -> (w3866:dbl)
        n1743 = call <vilib>:"WPI_MotorControlRefNum Registry Get.vi"("refnum name"="Acquire") -> ("error out"=w3859:errorcluster, "MotorControlDevRef"=w3860:T8)  [unwired: 9 in]
        n1744 = call <vilib>:"WPI_MotorControlRefNum Registry Get.vi"("refnum name"="Dart 1") -> ("error out"=w3870:errorcluster, "MotorControlDevRef"=w3869:T8)  [unwired: 9 in]
        n1745 = Increment(x=w3858) -> (x+1=w3845:i32)
        n1746 = call-poly <vilib>:"PID.vi"("PID gains"=T7 {"proportional gain (Kc)"=1.0, "integral time (Ti, min)"=0.01, "derivative time (Td, min)"=0.0}, "process variable"=w3866, "setpoint"=0.0) -> ("output"=w3871:dbl)  [unwired: 7 in, 1 out]
        n1747 = Greater Or Equal?(x=w3845, y=100) -> (x >= y?=w3850:bool)
        n1748 = call <vilib>:"WPI_MotorControlSetOutput.vi"("error in (no error)"=w3870, "Output"=w3871, "MotorControlDevRef"=w3869) -> ()  [unwired: 6 in, 3 out]
        n1749 = call <vilib>:"WPI_MotorControlSetOutput.vi"("error in (no error)"=w3859, "Output"=-1.0, "MotorControlDevRef"=w3860) -> ()  [unwired: 6 in, 3 out]
        n1750 = Select(t=WPI_SolenoidValue."Forward" ("Value"), s=w3850, f=WPI_SolenoidValue."Off" ("Value")) -> (s? t:f=w3853:T6)
        n1751 = Wait (ms)(milliseconds to wait=u32 20) -> ()  [unwired: 1 out]
        n1752 = call <vilib>:"WPI_SolenoidRefNum Registry Get.vi"("refnum name"="Push") -> ("error out"=w3854:errorcluster, "SolenoidDevRef"=w3855:T16)  [unwired: 9 in]
        n1753 = call-poly <vilib>:"WPI_SolenoidSet.vi"("error in (no error)"=w3854, "Value"=w3853, "SolenoidDevRef"=w3855) -> ("error out"=w3846:errorcluster, "SolenoidDevRef"=w3847:T16)  [unwired: 7 in]
        n1754 = call-poly <vilib>:"WPI_SolenoidGet.vi"("error in (no error)"=w3846, "SolenoidDevRef"=w3847) -> ("Value"=w3844:bool)  [unwired: 7 in, 2 out]
      }
      n1755 = while {
        tunnel: w3566 -> [w3836]
        tunnel: w3565 -> [w3835]
        tunnel: w3564 -> [w3834]
        tunnel: w3563 -> [w3833]
        tunnel: [w3836] -> _
        tunnel: [w3835] -> _
        tunnel: [w3834] -> _
        tunnel: [w3833] -> _
        i -> [w3824]
        stop <- w3823 stop-if-true
        # "Reset"
        n1756 = call <vilib>:"WPI_SolenoidRefNum Registry Get.vi"("refnum name"="Push") -> ("error out"=w3840:errorcluster, "SolenoidDevRef"=w3841:T16)  [unwired: 9 in]
        n1757 = call <vilib>:"WPI_MotorControlRefNum Registry Get.vi"("refnum name"="Dart 1") -> ("error out"=w3831:errorcluster, "MotorControlDevRef"=w3830:T8)  [unwired: 9 in]
        n1758 = Increment(x=w3824) -> (x+1=w3837:i32)
        n1759 = global read "Robot Global Data.vi" "Pot 1"() -> (w3827:dbl)
        n1760 = Greater Or Equal?(x=w3837, y=100) -> (x >= y?=w3823:bool)
        n1761 = call-poly <vilib>:"PID.vi"("PID gains"=T7 {"proportional gain (Kc)"=1.0, "integral time (Ti, min)"=0.01, "derivative time (Td, min)"=0.0}, "process variable"=w3827, "setpoint"=0.0) -> ("output"=w3832:dbl)  [unwired: 7 in, 1 out]
        n1762 = call <vilib>:"WPI_MotorControlSetOutput.vi"("error in (no error)"=w3831, "Output"=w3832, "MotorControlDevRef"=w3830) -> ()  [unwired: 6 in, 3 out]
        n1763 = call-poly <vilib>:"WPI_SolenoidSet.vi"("error in (no error)"=w3840, "Value"=WPI_SolenoidValue."Reverse", "SolenoidDevRef"=w3841) -> ("error out"=w3838:errorcluster, "SolenoidDevRef"=w3839:T16)  [unwired: 7 in]
        n1764 = call-poly <vilib>:"WPI_SolenoidGet.vi"("error in (no error)"=w3838, "SolenoidDevRef"=w3839) -> ()  [unwired: 7 in, 3 out]
      }
    }
    frame "Drive forward" {
      # "done"
      n1765 = call <vilib>:"WPI_MotorControlRefNum Registry Get.vi"("refnum name"="Left Lead") -> ("error out"=w3939:errorcluster, "MotorControlDevRef"=w3940:T8)  [unwired: 9 in]
      n1766 = call <vilib>:"WPI_MotorControlRefNum Registry Get.vi"("refnum name"="Right Lead") -> ("error out"=w3937:errorcluster, "MotorControlDevRef"=w3938:T8)  [unwired: 9 in]
      n1767 = while {
        tunnel: w3940 -> [w3948]
        tunnel: w3939 -> [w3947]
        tunnel: w3938 -> [w3946]
        tunnel: w3937 -> [w3945]
        tunnel: [w3948] -> w3944
        tunnel: [w3947] -> w3943
        tunnel: [w3946] -> w3942
        tunnel: [w3945] -> w3941
        i -> [w3958]
        stop <- w3957 stop-if-true
        n1768 = Increment(x=w3958) -> (x+1=w3960:i32)
        n1769 = Greater?(x=w3960, y=10) -> (0:w3957:bool)
        n1770 = call <vilib>:"CTRE_PigeonIMU_RefNumRegistryGet.vi"("refnum name"="Pigeon") -> ("PigeonIMUDevRef"=w3955:T13)  [unwired: 9 in, 1 out]
        n1771 = call-poly <vilib>:"CTRE_Phoenix_MotorController_Get_Enhanced.vi"("PhoenixMotorControlDevRef"=w3948, "error in"=w3947) -> ("PhoenixMotorControlDevRef"=w3950:T8)  [unwired: 10 in, 3 out]
        n1772 = call-poly <vilib>:"CTRE_Phoenix_MotorController_Get_Enhanced.vi"("PhoenixMotorControlDevRef"=w3946, "error in"=w3945) -> ("PhoenixMotorControlDevRef"=w3949:T8)  [unwired: 10 in, 3 out]
        n1773 = call "CTRE_Phoenix_MotorControl_SetQuadraturePosition_Enhanced.vi"("New Position"=0, "PhoenixMotorControlDevRef"=w3949) -> ()  [unwired: 8 in, 2 out]
        n1774 = call "CTRE_Phoenix_MotorControl_SetQuadraturePosition_Enhanced.vi"("New Position"=0, "PhoenixMotorControlDevRef"=w3950) -> ()  [unwired: 8 in, 2 out]
        n1775 = Wait (ms)(milliseconds to wait=u32 20) -> ()  [unwired: 1 out]
        n1776 = call <vilib>:"CTRE_PigeonIMU_SetYaw.vi"("Value"=0.0, "PigeonIMUDevRef"=w3955) -> ()  [unwired: 8 in, 2 out]
      }
      n1777 = while {
        tunnel: [w3963] -> _
        tunnel: w3944 -> [w3963]
        tunnel: [w3964] -> _
        tunnel: w3943 -> [w3964]
        tunnel: [w3971] -> _
        tunnel: w3942 -> [w3971]
        tunnel: [w3970] -> _
        tunnel: w3941 -> [w3970]
        i -> [w3987]
        stop <- w3983 stop-if-true
        n1778 = global read "Robot Global Data.vi" "YAW"() -> (w3972:dbl)
        n1779 = Wait (ms)(milliseconds to wait=u32 20) -> ()  [unwired: 1 out]
        n1780 = call <vilib>:"WPI_RobotDriveRefNum Registry Get.vi"("refnum name"="RobotDrive") -> ("error out"=w3968:errorcluster, "RobotDriveDevRef"=w3969:T15)  [unwired: 9 in]
        n1781 = Increment(x=w3987) -> (x+1=w3986:i32)
        n1782 = call-poly <vilib>:"PID.vi"("output range"=cluster{"output high":dbl, "output low":dbl} {"output high"=0.4, "output low"=-0.4}, "PID gains"=T7 {"proportional gain (Kc)"=0.11, "integral time (Ti, min)"=0.0, "derivative time (Td, min)"=0.0}, "process variable"=w3972, "setpoint"=0.0) -> ("output"=w3962:dbl)  [unwired: 6 in, 1 out]
        n1783 = Greater Or Equal?(x=w3986, y=100) -> (x >= y?=w3984:bool)
        n1784 = Negate(x=w3962) -> (-x=w3961:dbl)
        n1785 = call-poly <vilib>:"CTRE_Phoenix_MotorController_Get_Enhanced.vi"("PhoenixMotorControlDevRef"=w3963, "error in"=w3964) -> ("Quadrature Position"=w3982:i32)  [unwired: 10 in, 3 out]
        n1786 = To Double Precision Float(number=w3982) -> (double precision float=w3981:dbl)
        n1787 = feedback #33() -> (w3965:dbl)  [unwired: 1 in]
        n1788 = call-poly <vilib>:"WPI_RobotDriveArcadeDrive.vi"("error in (no error)"=w3968, "Y axis value"=w3965, "X axis value"=w3961, "RobotDriveDevRef"=w3969) -> ()  [unwired: 5 in, 3 out]
        n1789 = Absolute Value(x=w3981) -> (abs(x)=w3977:dbl)
        n1790 = Greater Or Equal?(x=w3977, y=115000.0 ("upper limit")) -> (x >= y?=w3966:bool)
        n1791 = And(x=w3966, y=w3984) -> (x .and. y?=w3983:bool)
        n1792 = Select(t=0.0, s=w3966, f=-0.8) -> (s? t:f=w3978:dbl)
        n1793 = feedback-in #33(w3978) -> ()
      }
    }
  }
  n1794 = Format Into String(w11) -> (resulting string=→"Robots Decision 2":string)  [unwired: 3 in, 1 out]
  n1795 = while {
    stop <- FALSE stop-if-true
    n1796 = call <vilib>:"WPI_DriverStationReport Robot Code State.vi"("Autonomous"=TRUE) -> ()  [unwired: 10 in, 1 out]
    n1797 = Wait (ms)(milliseconds to wait=u32 20) -> ()  [unwired: 1 out]
  }
  n1798 = call <vilib>:"WPI_DriverStationGet Alliance Info.vi"() -> ()  [unwired: 12 out]
  n1799 = call <vilib>:"WPI_JoystickRefNum Registry Get.vi"("refnum name"="Joystick 0") -> ("JoystickDevRef"=w49:T2)  [unwired: 1 in, 9 out]
  n1800 = call <vilib>:"WPI_JoystickGetValues.vi"("JoystickDevRef"=w49) -> ("Axes"=w46:dbl[])  [unwired: 6 in, 4 out]
  n1801 = call-poly <vilib>:"NT Read Value.vi"("Name"="Auto Selector") -> ()  [unwired: 9 in, 2 out]
  n1802 = call-poly <vilib>:"NT Write Value.vi"("Numeric Array"=w46, "Name"="Joystick 0/Axes") -> ()  [unwired: 9 in, 1 out]
  n1803 = Index Array(array=w46, index=2) -> ()  [unwired: 1 out]
